vi "Download_LatexPackages_GetPackageList.vi"() -> (3 "Array 2":string[](array[string]))   [LabVIEW 2014]
uses:
  <vilib>/httpClient/LabVIEWHTTPClient.lvlib
  <vilib>/regexp/Match Regular Expression.xnode
panel:
  out "Array 3":string[](array[string])
  out "Array":i32[](array[numeric])
  out "Array String":string[][](array[string])
  out "body":string
  out "headers":string
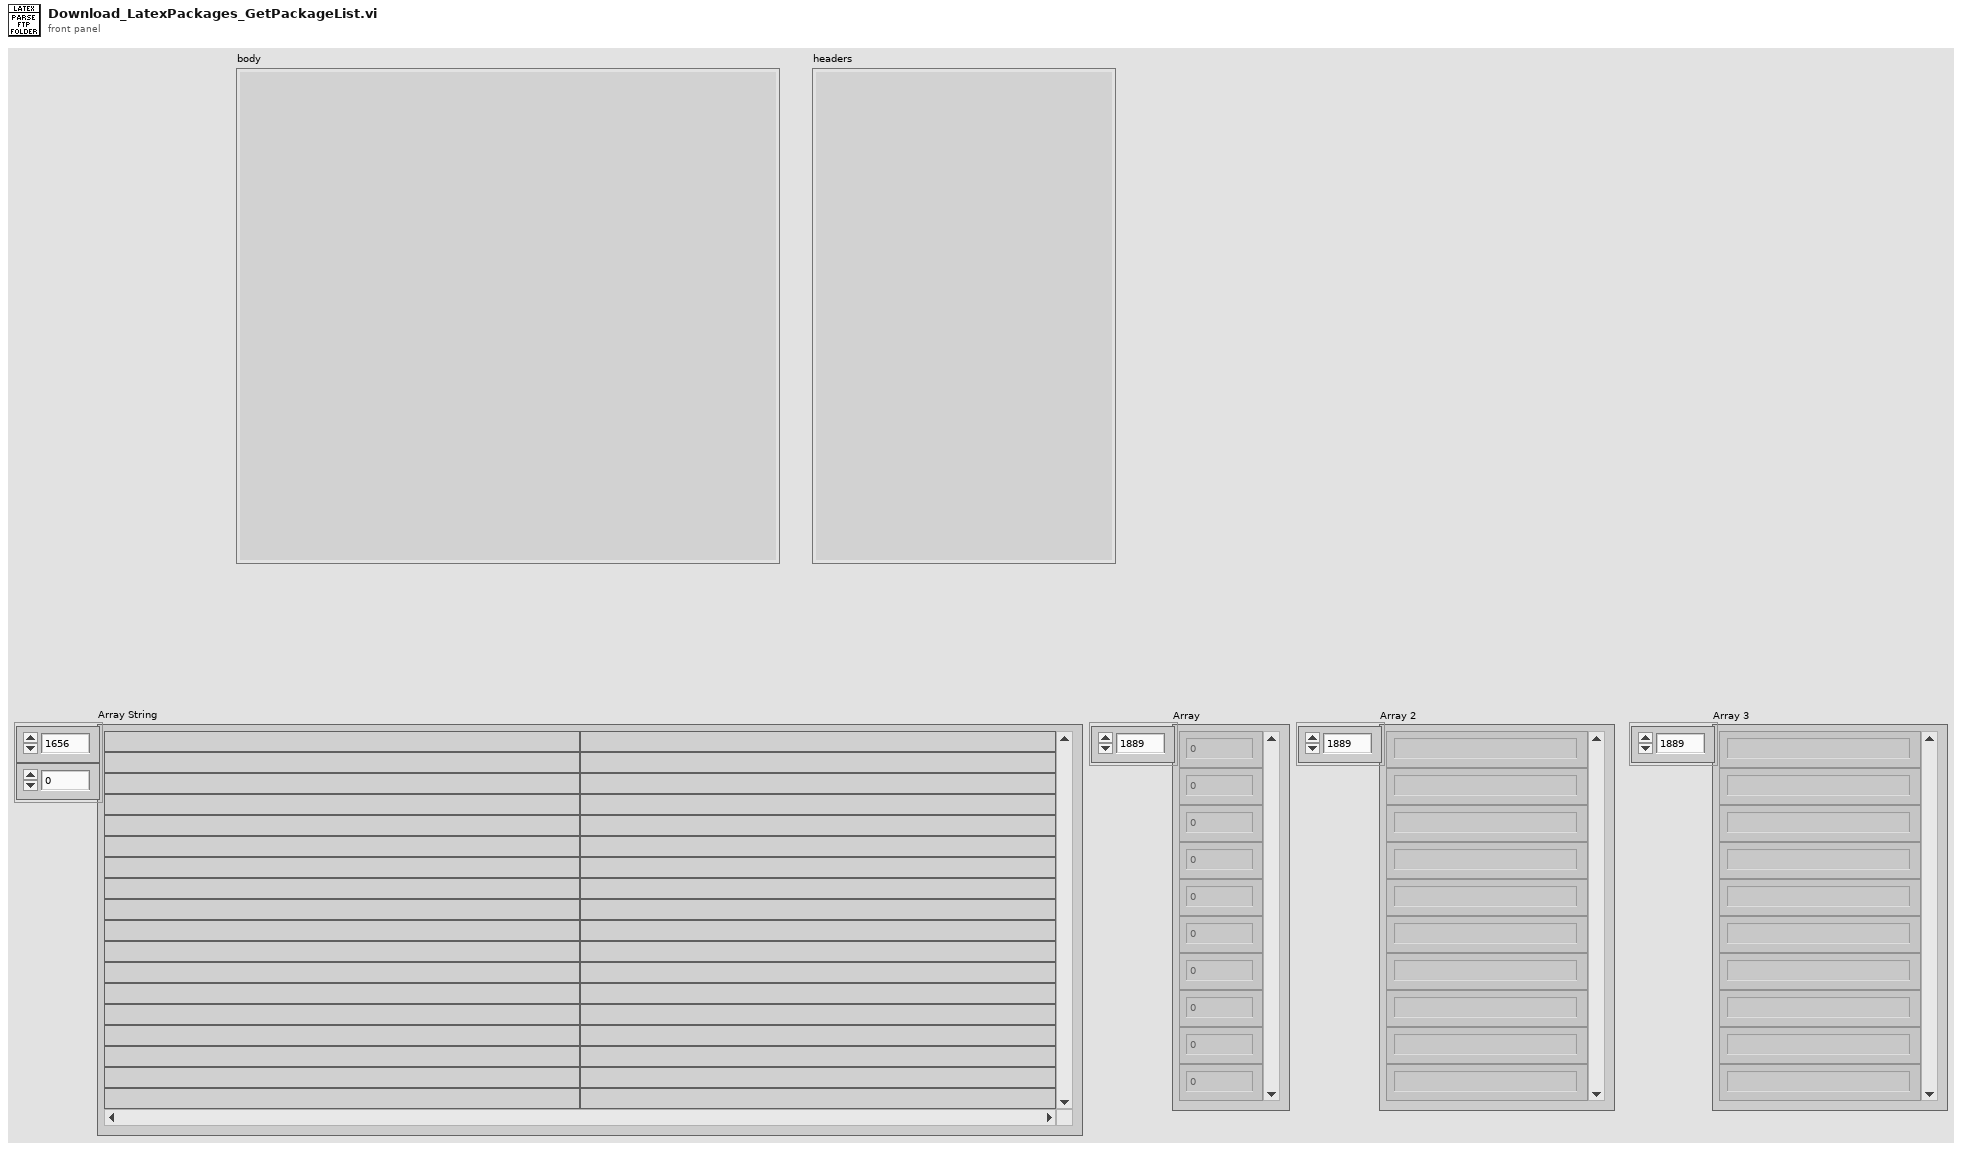
[diagram p1: front panel]
types:
  T1 = typedef "LabVIEWHTTPClient.lvlib/ClientHandle.ctl" = refnum<k1>
diagram:
  (unwired) "[a-zA-z0-9]+\\.zip" ("regular expression")
  w11 = "\nIndex of /ftp/pub/mirror/ctan/macros/latex/contrib\n\nIcon  Name                               Last modified      Size  Description[DIR] Parent Directory                                        -   \n[   ] 12many.zip                         09-Apr-2005 19:47  374K  \n[DIR] 12many/                            09-Apr-2005 19:47    -   \n[   ] ESIEEcv.zip                        29-Apr-2009 20:27  137K  \n[DIR] ESIEEcv/                           29-Apr-2009 20:33    -   \n[DIR] GuIT/                              19-Aug-2012 10:33    -   \n[   ] IEEEconf.zip                       05-Apr-2009 23:09  191K  \n[DIR] IEEEconf/                          05-Apr-2009 23:13    -   \n[   ] IEEEtran.zip                       28-Aug-2015 21:33  1.6M  \n[DIR] IEEEtran/                          28-Aug-2015 21:33    -   \n[   ] LingTrees.zip                      09-Mar-2006 02:00  177K  \n[DIR] LingTrees/                         09-Dec-2013 19:31    -   \n[   ] SIstyle.zip                        16-Jul-2008 15:58  387K  \n[DIR] SIstyle/                           16-Jul-2008 16:03    -   \n[   ] SIunits.zip                        02-Dec-2007 14:15  289K  \n[DIR] SIunits/                           02-Dec-2007 14:23    -   \n[   ] Tabbing.zip                        14-Feb-2010 11:53  215K  \n[DIR] Tabbing/                           14-Feb-2010 12:03    -   \n[   ] TeXemplar.zip                      28-Apr-2005 00:48  7.8K  \n[DIR] TeXemplar/                         01-Feb-2005 20:43    -   \n[   ] a0poster.zip                       28-Apr-2005 00:38  138K  \n[DIR] a0poster/                          01-Feb-2005 20:43    -   \n[DIR] a4/                                23-Jan-2006 08:44    -   \n[   ] a4wide.zip                         05-Jan-2011 01:38  131K  \n[DIR] a4wide/                            05-Jan-2011 02:03    -   \n[   ] a5comb.zip                         13-Feb-2010 22:17   90K  \n[DIR] a5comb/                            13-Feb-2010 22:23    -   \n[   ] aastex.zip                         02-Mar-2016 21:30  1.4M  \n[DIR] aastex/                            02-Mar-2016 21:30    -   \n[   ] abc.zip                            15-May-2016 20:08  281K  \n[DIR] abc/                               15-May-2016 20:08    -   \n[   ] abnt.zip                           31-Oct-2017 16:27   93K  \n[DIR] abnt/                              31-Oct-2017 16:27    -   \n[   ] abntex2.zip                        27-Feb-2016 15:29  6.5M  \n[DIR] abntex2/                           27-Feb-2016 15:29    -   \n[   ] abraces.zip                        31-Aug-2012 11:28  195K  \n[DIR] abraces/                           31-Aug-2012 11:33    -   \n[   ] abstract.zip                       02-Sep-2009 10:13  154K  \n[DIR] abstract/                          02-Sep-2009 10:23    -   \n[   ] achemso.zip                        05-Feb-2018 23:08  872K  \n[DIR] achemso/                           05-Feb-2018 23:08    -   \n[   ] acmart.zip                         07-Feb-2018 20:26  9.5M  \n[DIR] acmart/                            07-Feb-2018 20:26    -   \n[   ] acmconf.zip                        14-May-2008 20:12  103K  \n[DIR] acmconf/                           14-May-2008 19:13    -   \n[   ] acro.zip                           30-Jan-2018 20:37  601K  \n[DIR] acro/                              30-Jan-2018 20:37    -   \n[   ] acroflex.zip                       29-Aug-2016 17:01  1.3M  \n[DIR] acroflex/                          29-Aug-2016 17:01    -   \n[   ] acromake.zip                       15-Feb-2010 23:37  158K  \n[DIR] acromake/                          15-Feb-2010 23:43    -   \n[   ] acronym.zip                        21-Mar-2015 18:51  278K  \n[DIR] acronym/                           21-Mar-2015 18:51    -   \n[   ] acroterm.zip                       19-Nov-2010 14:07  159K  \n[DIR] acroterm/                          19-Nov-2010 14:13    -   \n[   ] acrotex.zip                        01-Mar-2018 17:18  2.9M  \n[DIR] acrotex/                           01-Mar-2018 17:18    -   \n[   ] actuarialangle.zip                 11-Apr-2017 18:43  108K  \n[DIR] actuarialangle/                    11-Apr-2017 18:43    -   \n[   ] actuarialsymbol.zip                14-Jun-2017 22:33  352K  \n[DIR] actuarialsymbol/                   14-Jun-2017 22:33    -   \n[   ] addfont.zip                        01-Sep-2016 13:30  105K  \n[DIR] addfont/                           01-Sep-2016 13:30    -   \n[   ] addlines.zip                       08-Jul-2015 05:24  139K  \n[DIR] addlines/                          08-Jul-2015 05:24    -   \n[   ] adfathesis.zip                     28-Apr-2005 00:49  148K  \n[DIR] adfathesis/                        01-Feb-2005 20:43    -   \n[   ] adjmulticol.zip                    24-Jan-2013 11:50  303K  \n[DIR] adjmulticol/                       24-Jan-2013 11:50    -   \n[   ] adjustbox.zip                      21-May-2012 17:04  789K  \n[DIR] adjustbox/                         21-May-2012 17:13    -   \n[   ] adrconv.zip                        04-Mar-2018 12:53  679K  \n[DIR] adrconv/                           04-Mar-2018 12:53    -   \n[   ] adrlist.zip                        14-May-2008 20:13   47K  \n[DIR] adrlist/                           14-May-2008 19:23    -   \n[   ] adtrees.zip                        20-Jan-2016 14:58  313K  \n[DIR] adtrees/                           20-Jan-2016 14:58    -   \n[   ] advdate.zip                        22-Nov-2010 08:58  145K  \n[DIR] advdate/                           22-Nov-2010 09:03    -   \n[   ] aeb_mlink.zip                      17-Feb-2016 16:07  238K  \n[DIR] aeb_mlink/                         17-Feb-2016 16:07    -   \n[   ] aeb_mobile.zip                     03-Jul-2012 11:37  894K  \n[DIR] aeb_mobile/                        03-Jul-2012 11:43    -   \n[DIR] aeb_pro/                           04-Mar-2018 05:48    -   \n[   ] aeb_tilebg.zip                     18-Feb-2016 20:34  2.3M  \n[DIR] aeb_tilebg/                        18-Feb-2016 20:34    -   \n[   ] aeguill.zip                        29-Apr-2009 20:28   32K  \n[DIR] aeguill/                           29-Apr-2009 20:33    -   \n[   ] afparticle.zip                     23-Dec-2014 21:11  607K  \n[DIR] afparticle/                        23-Dec-2014 21:11    -   \n[   ] afthesis.zip                       28-Jul-2008 22:25   52K  \n[DIR] afthesis/                          28-Jul-2008 21:33    -   \n[   ] aguplus.zip                        21-Feb-2010 22:10  395K  \n[DIR] aguplus/                           21-Feb-2010 22:13    -   \n[   ] aiaa.zip                           28-Apr-2005 00:49  1.0M  \n[DIR] aiaa/                              01-Feb-2005 20:43    -   \n[   ] akktex.zip                         25-Oct-2006 18:48   31K  \n[DIR] akktex/                            25-Oct-2006 18:53    -   \n[   ] akletter.zip                       28-Apr-2005 00:49  217K  \n[DIR] akletter/                          01-Feb-2005 20:43    -   \n[   ] alertmessage.zip                   04-Aug-2015 13:00  112K  \n[DIR] alertmessage/                      04-Aug-2015 13:00    -   \n[   ] alg.zip                            28-Apr-2005 00:49  6.9K  \n[DIR] alg/                               01-Feb-2005 20:43    -   \n[   ] algobox.zip                        04-Sep-2017 22:11  143K  \n[DIR] algobox/                           04-Sep-2017 22:11    -   \n[   ] algorithm2e.zip                    19-Jul-2017 09:50  586K  \n[DIR] algorithm2e/                       19-Jul-2017 09:50    -   \n[   ] algorithmicx.zip                   26-Aug-2009 07:31  179K  \n[DIR] algorithmicx/                      26-Aug-2009 07:31    -   \n[   ] algorithms.zip                     25-Aug-2009 13:09  304K  \n[DIR] algorithms/                        25-Aug-2009 13:13    -   \n[   ] aligned-overset.zip                29-Jan-2018 15:27  352K  \n[DIR] aligned-overset/                   29-Jan-2018 15:27    -   \n[   ] alnumsec.zip                       25-Sep-2007 14:55  129K  \n[DIR] alnumsec/                          25-Sep-2007 14:55    -   \n[   ] alterqcm.zip                       05-Jun-2011 21:03  1.3M  \n[DIR] alterqcm/                          05-Jun-2011 21:03    -   \n[   ] altfont.zip                        07-Dec-2006 01:00  181K  \n[DIR] altfont/                           16-Aug-2008 14:43    -   \n[   ] ametsoc.zip                        05-Jan-2015 19:14  414K  \n[DIR] ametsoc/                           05-Jan-2015 19:14    -   \n[   ] amsaddr.zip                        03-Apr-2013 11:32  193K  \n[DIR] amsaddr/                           03-Apr-2013 11:32    -   \n[   ] amsrefs.zip                        09-Mar-2013 15:03  2.1M  \n[DIR] amsrefs/                           09-Mar-2013 15:03    -   \n[   ] analogclock.zip                    22-Dec-2008 13:50   68K  \n[DIR] analogclock/                       22-Dec-2008 13:50    -   \n[   ] animate.zip                        28-Feb-2018 14:24  3.1M  \n[DIR] animate/                           28-Feb-2018 14:24    -   \n[   ] annot_pro.zip                      28-Aug-2017 12:42  1.7M  \n[DIR] annot_pro/                         28-Aug-2017 12:42    -   \n[   ] anonchap.zip                       14-Feb-2010 23:18  183K  \n[DIR] anonchap/                          14-Feb-2010 23:23    -   \n[   ] answers.zip                        24-Aug-2014 12:16  213K  \n[DIR] answers/                           24-Aug-2014 12:16    -   \n[DIR] anufinalexam/                      16-Jul-2012 11:17    -   \n[   ] anyfontsize.zip                    03-Apr-2010 23:16  181K  \n[DIR] anyfontsize/                       03-Apr-2010 23:16    -   \n[   ] anysize.zip                        01-Jun-2008 22:40   36K  \n[DIR] anysize/                           01-Jun-2008 21:43    -   \n[   ] aomart.zip                         16-Dec-2017 21:56  1.6M  \n[DIR] aomart/                            16-Dec-2017 21:56    -   \n[   ] apa.zip                            23-Dec-2008 13:04   49K  \n[DIR] apa/                               23-Dec-2008 13:13    -   \n[   ] apa6.zip                           20-Jun-2017 21:13  612K  \n[DIR] apa6/                              20-Jun-2017 21:13    -   \n[   ] apa6e.zip                          30-Dec-2012 12:36  249K  \n[DIR] apa6e/                             30-Dec-2012 12:43    -   \n[   ] apacite.zip                        22-Jul-2013 09:38  799K  \n[DIR] apacite/                           22-Jul-2013 09:38    -   \n[   ] appendix.zip                       08-Sep-2009 12:17  168K  \n[DIR] appendix/                          08-Sep-2009 12:23    -   \n[   ] apptools.zip                       29-Nov-2012 15:08   85K  \n[DIR] apptools/                          29-Nov-2012 15:08    -   \n[   ] apxproof.zip                       31-May-2017 11:16  449K  \n[DIR] apxproof/                          31-May-2017 11:16    -   \n[   ] arcs.zip                           28-Apr-2005 00:49   54K  \n[DIR] arcs/                              01-Feb-2005 20:43    -   \n[   ] arraysort.zip                      04-Sep-2013 23:38  305K  \n[DIR] arraysort/                         04-Sep-2013 23:43    -   \n[   ] arsclassica.zip                    31-Oct-2017 18:25  421K  \n[DIR] arsclassica/                       31-Oct-2017 18:25    -   \n[   ] articleingud.zip                   30-Oct-2015 17:00  423K  \n[DIR] articleingud/                      30-Oct-2015 17:00    -   \n[   ] artthreads.zip                     09-Apr-2016 18:30  108K  \n[DIR] artthreads/                        09-Apr-2016 18:30    -   \n[   ] arydshln.zip                       29-Apr-2016 14:56  923K  \n[DIR] arydshln/                          29-Apr-2016 14:56    -   \n[   ] asaetr.zip                         29-Apr-2009 20:29  122K  \n[DIR] asaetr/                            29-Apr-2009 20:33    -   \n[   ] ascelike.zip                       15-Feb-2013 11:40  125K  \n[DIR] ascelike/                          15-Feb-2013 11:43    -   \n[   ] asciilist.zip                      15-May-2016 14:03  387K  \n[DIR] asciilist/                         15-May-2016 14:03    -   \n[   ] ascmac.zip                         09-Mar-2018 16:24  175K  \n[DIR] ascmac/                            09-Mar-2018 16:24    -   \n[   ] askmaps.zip                        04-Dec-2013 19:14  306K  \n[DIR] askmaps/                           04-Dec-2013 19:14    -   \n[   ] aspectratio.zip                    27-Sep-2012 21:09  449K  \n[DIR] aspectratio/                       30-Jan-2012 17:56    -   \n[   ] assignment.zip                     28-Apr-2005 00:49   84K  \n[DIR] assignment/                        01-Feb-2005 20:43    -   \n[   ] assoccnt.zip                       29-Sep-2015 20:56  349K  \n[DIR] assoccnt/                          29-Sep-2015 20:56    -   \n[   ] asyfig.zip                         25-Sep-2012 13:20  225K  \n[DIR] asyfig/                            20-Mar-2010 11:13    -   \n[   ] attachfile.zip                     19-Sep-2016 09:46  359K  \n[DIR] attachfile/                        19-Sep-2016 09:46    -   \n[   ] aucklandthesis.zip                 19-Jun-2016 23:41  696K  \n[DIR] aucklandthesis/                    19-Jun-2016 23:41    -   \n[   ] aurl.zip                           12-Aug-2016 15:34   15K  \n[DIR] aurl/                              12-Aug-2016 15:34    -   \n[   ] authoraftertitle.zip               17-Dec-2011 14:31  113K  \n[DIR] authoraftertitle/                  17-Dec-2011 14:33    -   \n[   ] authorarchive.zip                  21-Feb-2018 07:57  208K  \n[DIR] authorarchive/                     21-Feb-2018 07:57    -   \n[   ] auto-pst-pdf-lua.zip               19-Mar-2018 09:09   70K  \n[DIR] auto-pst-pdf-lua/                  19-Mar-2018 09:09    -   \n[   ] auto-pst-pdf.zip                   26-Aug-2011 08:29  335K  \n[DIR] auto-pst-pdf/                      26-Aug-2011 08:29    -   \n[   ] autobreak.zip                      25-Feb-2017 06:11  540K  \n[DIR] autobreak/                         25-Feb-2017 06:11    -   \n[   ] autonum.zip                        18-Jan-2015 10:18  409K  \n[DIR] autonum/                           18-Jan-2015 10:18    -   \n[   ] autopdf.zip                        10-Dec-2013 19:56  235K  \n[DIR] autopdf/                           10-Dec-2013 19:56    -   \n[   ] avremu.zip                         14-Oct-2014 20:13  189K  \n[DIR] avremu/                            14-Oct-2014 20:13    -   \n[DIR] axodraw2/                          20-Feb-2018 19:13    -   \n[   ] b1encoding.zip                     03-Dec-2005 12:12  151K  \n[DIR] b1encoding/                        05-Dec-2005 20:21    -   \n[DIR] babel-contrib/                     30-Mar-2018 14:15    -   \n[   ] background.zip                     04-Mar-2014 20:59  121K  \n[DIR] background/                        04-Mar-2014 20:59    -   \n[   ] backnaur.zip                       12-Dec-2012 18:29  293K  \n[DIR] backnaur/                          12-Dec-2012 18:33    -   \n[   ] bangorcsthesis.zip                 16-Aug-2017 13:00  345K  \n[DIR] bangorcsthesis/                    16-Aug-2017 13:00    -   \n[   ] bangorexam.zip                     13-Feb-2018 10:02  245K  \n[DIR] bangorexam/                        13-Feb-2018 10:02    -   \n[   ] bankstatement.zip                  14-Nov-2015 18:53  132K  \n[DIR] bankstatement/                     14-Nov-2015 18:53    -   \n[   ] bashful.zip                        10-Mar-2012 20:42  559K  \n[DIR] bashful/                           10-Mar-2012 20:43    -   \n[   ] basicarith.zip                     27-Oct-2014 22:17  224K  \n[DIR] basicarith/                        27-Oct-2014 22:17    -   \n[   ] basque-book.zip                    11-Feb-2014 19:09  437K  \n[DIR] basque-book/                       11-Feb-2014 19:09    -   \n[   ] basque-date.zip                    10-Feb-2014 01:42  192K  \n[DIR] basque-date/                       10-Feb-2014 02:03    -   \n[DIR] bbding/                            23-Feb-2010 23:23    -   \n[   ] bbm.zip                            15-Feb-2010 23:27  403K  \n[DIR] bbm/                               15-Feb-2010 23:33    -   \n[   ] bchart.zip                         18-Apr-2017 22:02  147K  \n[DIR] bchart/                            18-Apr-2017 22:02    -   \n[   ] beamer-FUBerlin.zip                19-Aug-2015 20:36  595K  \n[DIR] beamer-FUBerlin/                   19-Aug-2015 20:36    -   \n[DIR] beamer-contrib/                    29-Jan-2018 23:21    -   \n[   ] beamer.zip                         20-Feb-2018 22:45  2.9M  \n[DIR] beamer/                            20-Feb-2018 22:45    -   \n[   ] beamerposter.zip                   22-Apr-2015 07:02   79K  \n[DIR] beamerposter/                      22-Apr-2015 07:02    -   \n[   ] begingreek.zip                     16-Feb-2015 20:30  698K  \n[DIR] begingreek/                        16-Feb-2015 20:30    -   \n[   ] begriff.zip                        27-May-2005 17:04   44K  \n[DIR] begriff/                           27-May-2005 19:13    -   \n[   ] beilstein.zip                      30-Jan-2018 22:13  1.4M  \n[DIR] beilstein/                         30-Jan-2018 22:13    -   \n[   ] betababel.zip                      10-Jul-2005 16:36  142K  \n[DIR] betababel/                         10-Jul-2005 17:43    -   \n[   ] beton.zip                          01-Jun-2008 22:49   67K  \n[DIR] beton/                             01-Jun-2008 21:53    -   \n[   ] bewerbung.zip                      14-Jul-2015 15:37  917K  \n[DIR] bewerbung/                         14-Jul-2015 15:37    -   \n[   ] bez123.zip                         08-Sep-2009 12:50  268K  \n[DIR] bez123/                            08-Sep-2009 12:53    -   \n[   ] bezos.zip                          25-Feb-2012 16:12  1.0M  \n[DIR] bezos/                             25-Feb-2012 16:12    -   \n[   ] bg.zip                             29-Apr-2009 20:36  120K  \n[DIR] bg/                                25-Sep-2012 13:28    -   \n[   ] bgteubner.zip                      05-May-2017 00:01  2.7M  \n[DIR] bgteubner/                         05-May-2017 00:01    -   \n[   ] bhcexam.zip                        07-Dec-2015 16:01   18K  \n[DIR] bhcexam/                           07-Dec-2015 16:01    -   \n[   ] bibarts.zip                        20-Mar-2016 21:17  1.2M  \n[DIR] bibarts/                           20-Mar-2016 21:17    -   \n[DIR] biblatex-contrib/                  29-Mar-2018 14:02    -   \n[   ] biblatex.zip                       04-Mar-2018 21:16   18M  \n[DIR] biblatex/                          04-Mar-2018 21:16    -   \n[   ] bibleref-french.zip                03-Nov-2014 15:44  716K  \n[DIR] bibleref-french/                   03-Nov-2014 15:44    -   \n[   ] bibleref-german.zip                02-Apr-2011 18:27  787K  \n[DIR] bibleref-german/                   02-Apr-2011 18:27    -   \n[   ] bibleref-lds.zip                   27-Feb-2012 12:33  274K  \n[DIR] bibleref-lds/                      27-Feb-2012 12:43    -   \n[   ] bibleref-mouth.zip                 27-Feb-2012 11:52  381K  \n[DIR] bibleref-mouth/                    27-Feb-2012 12:03    -   \n[   ] bibleref-parse.zip                 11-Apr-2011 08:18  109K  \n[DIR] bibleref-parse/                    11-Apr-2011 08:18    -   \n[   ] bibleref.zip                       01-Jul-2017 09:52  357K  \n[DIR] bibleref/                          01-Jul-2017 09:52    -   \n[   ] bibletext.zip                      02-Sep-2017 12:47  138K  \n[DIR] bibletext/                         02-Sep-2017 12:47    -   \n[   ] bibtopic.zip                       10-Sep-2006 02:00  263K  \n[DIR] bibtopic/                          16-Aug-2008 14:45    -   \n[   ] bibtopicprefix.zip                 31-Oct-2006 15:39  1.1M  \n[DIR] bibtopicprefix/                    31-Oct-2006 15:43    -   \n[   ] bibunits.zip                       30-Apr-2005 15:55  209K  \n[DIR] bibunits/                          01-Feb-2005 20:43    -   \n[   ] bidi.zip                           21-Feb-2018 14:23  3.7M  \n[DIR] bidi/                              21-Feb-2018 14:23    -   \n[   ] bigfoot.zip                        30-Aug-2015 19:08  824K  \n[DIR] bigfoot/                           30-Aug-2015 19:08    -   \n[   ] bigints.zip                        25-Sep-2012 13:39  114K  \n[DIR] bigints/                           26-Feb-2010 19:13    -   \n[   ] binomexp.zip                       11-Jan-2007 02:03   71K  \n[DIR] binomexp/                          11-Jan-2007 02:13    -   \n[   ] biochemistry-colors.zip            21-Apr-2017 19:48   80K  \n[DIR] biochemistry-colors/               21-Apr-2017 19:48    -   \n[   ] biocon.zip                         30-Apr-2005 15:55  289K  \n[DIR] biocon/                            01-Feb-2005 20:43    -   \n[   ] bitpattern.zip                     11-Dec-2015 09:58  177K  \n[DIR] bitpattern/                        11-Dec-2015 09:58    -   \n[   ] bizcard.zip                        29-Apr-2009 20:39   79K  \n[DIR] bizcard/                           29-Apr-2009 20:43    -   \n[   ] blindtext.zip                      06-Jan-2012 11:44  358K  \n[DIR] blindtext/                         06-Jan-2012 11:44    -   \n[   ] blkarray.zip                       28-Feb-2015 05:33  305K  \n[DIR] blkarray/                          28-Feb-2015 05:33    -   \n[   ] block.zip                          16-Feb-2010 20:55   60K  \n[DIR] block/                             16-Feb-2010 21:03    -   \n[   ] blowup.zip                         04-Jan-2018 12:34  368K  \n[DIR] blowup/                            04-Jan-2018 12:34    -   \n[   ] bnumexpr.zip                       05-Dec-2017 23:13  100K  \n[DIR] bnumexpr/                          05-Dec-2017 23:13    -   \n[   ] bohr.zip                           24-Jun-2015 13:04  417K  \n[DIR] bohr/                              24-Jun-2015 13:04    -   \n[   ] boites.zip                         23-Nov-2013 07:43  282K  \n[DIR] boites/                            23-Nov-2013 07:43    -   \n[   ] bold-extra.zip                     16-Feb-2010 21:08  213K  \n[DIR] bold-extra/                        16-Feb-2010 21:13    -   \n[   ] boldtensors.zip                    02-Jul-2007 16:52   56K  \n[DIR] boldtensors/                       02-Jul-2007 16:52    -   \n[   ] bondgraph.zip                      09-Mar-2011 19:57   51K  \n[DIR] bondgraph/                         09-Mar-2011 19:57    -   \n[   ] bondgraphs.zip                     23-Mar-2015 13:26  363K  \n[DIR] bondgraphs/                        23-Mar-2015 13:26    -   \n[   ] bookcover.zip                      21-Jan-2018 22:30  3.1M  \n[DIR] bookcover/                         21-Jan-2018 22:30    -   \n[   ] bookest.zip                        20-Mar-2008 11:06  245K  \n[DIR] bookest/                           20-Mar-2008 11:13    -   \n[   ] booklet.zip                        08-Sep-2009 12:22  231K  \n[DIR] booklet/                           08-Sep-2009 12:23    -   \n[   ] booktabs-de.zip                    30-Mar-2011 20:33  270K  \n[DIR] booktabs-de/                       30-Mar-2011 20:33    -   \n[   ] booktabs.zip                       29-Apr-2016 10:59  301K  \n[DIR] booktabs/                          29-Apr-2016 10:59    -   \n[   ] boolexpr.zip                       12-Apr-2010 11:36  162K  \n[DIR] boolexpr/                          12-Apr-2010 11:43    -   \n[   ] bophook.zip                        31-Dec-2006 15:38   49K  \n[DIR] bophook/                           31-Dec-2006 15:43    -   \n[   ] bosisio.zip                        12-Feb-2010 13:27  526K  \n[DIR] bosisio/                           12-Feb-2010 08:45    -   \n[   ] boxedminipage.zip                  16-Feb-2010 19:50  115K  \n[DIR] boxedminipage/                     16-Feb-2010 19:53    -   \n[   ] boxedminipage2e.zip                10-Mar-2015 11:32  207K  \n[DIR] boxedminipage2e/                   10-Mar-2015 11:32    -   \n[   ] boxhandler.zip                     18-Oct-2012 22:58  342K  \n[DIR] boxhandler/                        18-Oct-2012 22:58    -   \n[   ] bpchem.zip                         23-Aug-2017 16:00  354K  \n[DIR] bpchem/                            23-Aug-2017 16:00    -   \n[   ] br-lex.zip                         01-Aug-2017 22:38   61K  \n[DIR] br-lex/                            01-Aug-2017 22:38    -   \n[   ] bracketkey.zip                     19-Feb-2010 21:28  289K  \n[DIR] bracketkey/                        19-Feb-2010 21:33    -   \n[   ] braille.zip                        04-Dec-2010 12:39   69K  \n[DIR] braille/                           04-Dec-2010 12:43    -   \n[   ] braket.zip                         21-Feb-2010 19:34  212K  \n[DIR] braket/                            21-Feb-2010 19:43    -   \n[   ] brandeis-dissertation.zip          31-Oct-2013 19:18  256K  \n[DIR] brandeis-dissertation/             31-Oct-2013 19:18    -   \n[   ] brclc.zip                          30-Apr-2005 15:56   80K  \n[DIR] brclc/                             01-Feb-2005 20:43    -   \n[   ] breakcites.zip                     10-Jan-2011 19:04  145K  \n[DIR] breakcites/                        10-Jan-2011 19:13    -   \n[   ] breakurl.zip                       12-Apr-2013 10:25  117K  \n[DIR] breakurl/                          12-Apr-2013 10:25    -   \n[   ] bredzenie.zip                      15-May-2017 09:55  216K  \n[DIR] bredzenie/                         15-May-2017 09:55    -   \n[   ] breqn.zip                          28-Jan-2017 14:46  1.2M  \n[DIR] breqn/                             28-Jan-2017 14:46    -   \n[   ] bropd.zip                          14-Oct-2014 21:36   64K  \n[DIR] bropd/                             14-Oct-2014 21:36    -   \n[   ] bsheaders.zip                      15-Apr-2005 07:46  1.6K  \n[DIR] bsheaders/                         15-Apr-2005 09:13    -   \n[   ] bullcntr.zip                       08-Oct-2008 11:56  743K  \n[DIR] bullcntr/                          08-Oct-2008 11:56    -   \n[   ] business-research.zip              01-Dec-2011 10:57  370K  \n[DIR] business-research/                 02-Dec-2011 01:20    -   \n[   ] bussproofs.zip                     21-Aug-2012 20:15  115K  \n[DIR] bussproofs/                        21-Aug-2012 20:15    -   \n[   ] bxcalc.zip                         28-Jan-2018 18:16  338K  \n[DIR] bxcalc/                            28-Jan-2018 18:16    -   \n[   ] bxdvidriver.zip                    13-Feb-2017 17:53  4.5K  \n[DIR] bxdvidriver/                       13-Feb-2017 17:53    -   \n[   ] bxeepic.zip                        18-May-2013 20:51   18K  \n[DIR] bxeepic/                           18-May-2013 20:53    -   \n[   ] bxenclose.zip                      02-Apr-2016 12:35  3.3K  \n[DIR] bxenclose/                         02-Apr-2016 12:35    -   \n[   ] bxnewfont.zip                      02-May-2017 22:55  6.8K  \n[DIR] bxnewfont/                         02-May-2017 22:55    -   \n[   ] bxorigcapt.zip                     03-May-2017 22:28  3.6K  \n[DIR] bxorigcapt/                        03-May-2017 22:28    -   \n[   ] bxpapersize.zip                    08-Oct-2017 08:36  8.1K  \n[DIR] bxpapersize/                       08-Oct-2017 08:36    -   \n[   ] bxpdfver.zip                       11-Feb-2017 22:01   11K  \n[DIR] bxpdfver/                          11-Feb-2017 22:01    -   \n[   ] bxtexlogo.zip                      31-Mar-2018 10:20  420K  \n[DIR] bxtexlogo/                         31-Mar-2018 10:20    -   \n[   ] bytefield.zip                      19-Sep-2017 08:21  573K  \n[DIR] bytefield/                         19-Sep-2017 08:21    -   \n[   ] cachepic.zip                       01-Oct-2009 11:31  163K  \n[DIR] cachepic/                          01-Oct-2009 11:33    -   \n[   ] calcage.zip                        16-Sep-2012 12:24  277K  \n[DIR] calcage/                           16-Sep-2012 12:24    -   \n[   ] calctab.zip                        14-Jul-2009 21:54  405K  \n[DIR] calctab/                           14-Jul-2009 21:54    -   \n[   ] calculation.zip                    06-Jan-2015 20:40  107K  \n[DIR] calculation/                       06-Jan-2015 20:40    -   \n[   ] calculator.zip                     24-Feb-2014 14:22  579K  \n[DIR] calculator/                        24-Feb-2014 14:22    -   \n[   ] calendar.zip                       26-Jul-2005 10:26  479K  \n[DIR] calendar/                          01-Feb-2005 20:43    -   \n[DIR] calendar_barr/                     03-Apr-2010 14:15    -   \n[   ] calrsfs.zip                        20-Feb-2010 21:55  151K  \n[DIR] calrsfs/                           20-Feb-2010 22:03    -   \n[   ] cals.zip                           20-Jan-2017 11:10  526K  \n[DIR] cals/                              20-Jan-2017 11:10    -   \n[   ] calxxxx-yyyy.zip                   03-Jan-2018 08:27  419K  \n[DIR] calxxxx-yyyy/                      03-Jan-2018 08:27    -   \n[   ] calxxxx.zip                        31-Dec-2006 11:32   52K  \n[DIR] calxxxx/                           31-Dec-2006 11:33    -   \n[   ] camel.zip                          30-Apr-2005 15:56  105K  \n[DIR] camel/                             01-Feb-2005 20:43    -   \n[   ] cancel.zip                         30-Dec-2013 10:32  256K  \n[DIR] cancel/                            30-Dec-2013 10:32    -   \n[   ] canoniclayout.zip                  06-Nov-2011 17:04  472K  \n[DIR] canoniclayout/                     06-Nov-2011 17:13    -   \n[   ] capt-of.zip                        25-Sep-2012 13:42   75K  \n[DIR] capt-of/                           22-Jan-2010 17:43    -   \n[   ] captcont.zip                       31-Dec-2006 11:44  110K  \n[DIR] captcont/                          31-Dec-2006 11:53    -   \n[   ] captdef.zip                        06-Mar-2010 15:15  212K  \n[DIR] captdef/                           06-Mar-2010 15:23    -   \n[   ] caption.zip                        22-May-2016 21:20  2.0M  \n[DIR] caption/                           22-May-2016 21:20    -   \n[   ] carbohydrates.zip                  02-Dec-2015 12:19  477K  \n[DIR] carbohydrates/                     02-Dec-2015 12:19    -   \n[   ] carlisle.zip                       11-May-2010 22:08   34K  \n[DIR] carlisle/                          11-May-2010 22:13    -   \n[   ] cascadilla.zip                     18-Jan-2012 11:58   98K  \n[DIR] cascadilla/                        18-Jan-2012 11:58    -   \n[   ] cases.zip                          20-Feb-2010 22:54  303K  \n[DIR] cases/                             20-Feb-2010 23:03    -   \n[   ] catchfilebetweentags.zip           19-Feb-2011 16:39  151K  \n[DIR] catchfilebetweentags/              19-Feb-2011 16:43    -   \n[   ] catechis.zip                       14-Jan-2018 10:32  402K  \n[DIR] catechis/                          14-Jan-2018 10:32    -   \n[   ] catoptions.zip                     30-Aug-2014 10:15   63K  \n[DIR] catoptions/                        30-Aug-2014 10:15    -   \n[   ] ccaption.zip                       07-Aug-2011 14:46  493K  \n[DIR] ccaption/                          07-Aug-2011 14:53    -   \n[   ] ccfonts.zip                        21-Feb-2010 01:25  193K  \n[DIR] ccfonts/                           21-Feb-2010 02:03    -   \n[   ] cchess.zip                         30-Apr-2005 15:56   15K  \n[DIR] cchess/                            01-Feb-2005 20:43    -   \n[   ] cclicenses.zip                     30-May-2005 14:36   84K  \n[DIR] cclicenses/                        30-May-2005 16:43    -   \n[   ] cd-cover.zip                       21-Feb-2010 01:35  311K  \n[DIR] cd-cover/                          21-Feb-2010 02:03    -   \n[   ] cd.zip                             27-Jun-2014 12:21   82K  \n[DIR] cd/                                27-Jun-2014 12:23    -   \n[   ] cdpbundl.zip                       12-Feb-2018 06:13  829K  \n[DIR] cdpbundl/                          12-Feb-2018 06:13    -   \n[   ] cell.zip                           14-Dec-2010 22:28   12K  \n[DIR] cell/                              14-Dec-2010 22:33    -   \n[   ] cellspace.zip                      13-Aug-2017 17:02  329K  \n[DIR] cellspace/                         13-Aug-2017 17:02    -   \n[   ] cellwise.zip                       08-Sep-2012 13:55  2.1K  \n[DIR] cellwise/                          08-Sep-2012 14:03    -   \n[   ] censor.zip                         31-Jul-2013 09:45  182K  \n[DIR] censor/                            31-Jul-2013 09:45    -   \n[   ] cesenaexam.zip                     05-Aug-2017 09:52  508K  \n[DIR] cesenaexam/                        05-Aug-2017 09:52    -   \n[   ] cfr-initials.zip                   06-Apr-2015 07:10  683K  \n[DIR] cfr-initials/                      06-Apr-2015 07:10    -   \n[   ] cfr-lm.zip                         02-Feb-2015 11:49  3.6M  \n[DIR] cfr-lm/                            02-Feb-2015 11:49    -   \n[   ] changebar.zip                      11-Mar-2018 17:34  745K  \n[DIR] changebar/                         11-Mar-2018 17:34    -   \n[   ] changelayout.zip                   15-Oct-2009 18:09   61K  \n[DIR] changelayout/                      15-Oct-2009 18:13    -   \n[   ] changepage.zip                     20-Oct-2009 20:40  281K  \n[DIR] changepage/                        20-Oct-2009 20:43    -   \n[   ] changes.zip                        28-Apr-2015 00:00  535K  \n[DIR] changes/                           28-Apr-2015 00:00    -   \n[   ] chappg.zip                         30-May-2009 11:04  193K  \n[DIR] chappg/                            30-May-2009 11:13    -   \n[   ] chapterfolder.zip                  25-Nov-2005 11:19  186K  \n[DIR] chapterfolder/                     16-Aug-2008 14:45    -   \n[   ] chbibref.zip                       21-Feb-2010 11:17  166K  \n[DIR] chbibref/                          21-Feb-2010 11:23    -   \n[   ] cheatsheet.zip                     18-Aug-2017 04:52  400K  \n[DIR] cheatsheet/                        18-Aug-2017 04:52    -   \n[   ] checklistings.zip                  04-Sep-2015 18:08  369K  \n[DIR] checklistings/                     04-Sep-2015 18:08    -   \n[   ] chemarrow.zip                      21-Feb-2010 18:49  433K  \n[DIR] chemarrow/                         21-Feb-2010 18:53    -   \n[   ] chemcompounds.zip                  05-Dec-2006 16:10  118K  \n[DIR] chemcompounds/                     05-Dec-2006 16:13    -   \n[   ] chemcono.zip                       21-Feb-2010 19:06  235K  \n[DIR] chemcono/                          21-Feb-2010 19:13    -   \n[   ] chemexec.zip                       06-Mar-2011 17:27  369K  \n[DIR] chemexec/                          06-Mar-2011 17:27    -   \n[   ] chemfig.zip                        08-Mar-2018 20:41  2.2M  \n[DIR] chemfig/                           08-Mar-2018 20:41    -   \n[   ] chemformula.zip                    23-Mar-2017 14:37  970K  \n[DIR] chemformula/                       23-Mar-2017 14:37    -   \n[   ] chemgreek.zip                      20-Dec-2016 12:45  720K  \n[DIR] chemgreek/                         20-Dec-2016 12:45    -   \n[   ] chemmacros.zip                     29-Aug-2017 12:53  1.1M  \n[DIR] chemmacros/                        29-Aug-2017 12:53    -   \n[   ] chemnum.zip                        14-Apr-2016 13:35  795K  \n[DIR] chemnum/                           14-Apr-2016 13:35    -   \n[   ] chemschemex.zip                    23-Feb-2018 21:14  316K  \n[DIR] chemschemex/                       23-Feb-2018 21:14    -   \n[   ] chemsec.zip                        15-Mar-2018 19:50  260K  \n[DIR] chemsec/                           15-Mar-2018 19:50    -   \n[   ] chemstyle.zip                      05-Jul-2013 11:10  291K  \n[DIR] chemstyle/                         05-Jul-2013 11:10    -   \n[   ] chemsym.zip                        23-Dec-2005 15:51  308K  \n[DIR] chemsym/                           13-Aug-2008 12:33    -   \n[   ] chess-problem-diagrams.zip         08-Jan-2016 10:22  313K  \n[DIR] chess-problem-diagrams/            08-Jan-2016 10:22    -   \n[   ] chessboard.zip                     01-May-2014 22:27  656K  \n[DIR] chessboard/                        01-May-2014 22:27    -   \n[   ] chessfss.zip                       10-Jan-2008 19:02  1.7M  \n[DIR] chessfss/                          10-Jan-2008 19:03    -   \n[   ] chet.zip                           19-Aug-2017 23:08  176K  \n[DIR] chet/                              19-Aug-2017 23:08    -   \n[   ] chextras.zip                       20-Jul-2012 14:21  134K  \n[DIR] chextras/                          20-Jul-2012 14:21    -   \n[   ] childdoc.zip                       17-Jan-2018 14:10  252K  \n[DIR] childdoc/                          17-Jan-2018 14:10    -   \n[   ] china2e.zip                        30-Apr-2005 15:56  106K  \n[DIR] china2e/                           01-Feb-2005 20:43    -   \n[   ] chkfloat.zip                       19-Aug-2012 23:58   46K  \n[DIR] chkfloat/                          20-Aug-2012 02:03    -   \n[   ] chletter.zip                       11-Oct-2010 07:19  146K  \n[DIR] chletter/                          11-Oct-2010 07:19    -   \n[   ] chngcntr.zip                       22-Feb-2010 20:14  229K  \n[DIR] chngcntr/                          22-Feb-2010 20:23    -   \n[   ] chronology.zip                     23-Jul-2015 07:01   14K  \n[DIR] chronology/                        23-Jul-2015 07:01    -   \n[   ] chronosys.zip                      28-May-2012 13:33  247K  \n[DIR] chronosys/                         28-May-2012 13:33    -   \n[   ] chscite.zip                        16-Dec-2012 17:14  195K  \n[DIR] chscite/                           16-Dec-2012 17:23    -   \n[   ] circle.zip                         22-Feb-2010 19:46  177K  \n[DIR] circle/                            22-Feb-2010 19:53    -   \n[   ] cite.zip                           03-Mar-2015 14:34  242K  \n[DIR] cite/                              03-Mar-2015 14:34    -   \n[DIR] citeref/                           30-Jul-2005 12:44    -   \n[   ] cje.zip                            23-Feb-2018 14:39  651K  \n[DIR] cje/                               23-Feb-2018 14:39    -   \n[   ] cjw.zip                            25-Sep-2012 14:09  519K  \n[DIR] cjw/                               25-Dec-2008 20:23    -   \n[   ] classics.zip                       03-Feb-2013 19:05  205K  \n[DIR] classics/                          03-Feb-2013 19:13    -   \n[   ] classicthesis.zip                  22-Oct-2017 10:02  583K  \n[DIR] classicthesis/                     22-Oct-2017 10:02    -   \n[   ] cleanthesis.zip                    27-Aug-2015 10:17  1.3M  \n[DIR] cleanthesis/                       27-Aug-2015 10:17    -   \n[   ] clefval.zip                        28-Dec-2009 11:06  335K  \n[DIR] clefval/                           28-Dec-2009 11:13    -   \n[   ] cleveref.zip                       05-Mar-2018 09:34  468K  \n[DIR] cleveref/                          05-Mar-2018 09:34    -   \n[   ] clipboard.zip                      19-Jan-2013 09:43   37K  \n[DIR] clipboard/                         19-Jan-2013 09:53    -   \n[   ] clock.zip                          30-Apr-2005 15:57   75K  \n[DIR] clock/                             23-Jan-2006 08:44    -   \n[   ] clrscode.zip                       29-Mar-2007 22:40   36K  \n[DIR] clrscode/                          29-Mar-2007 22:43    -   \n[   ] clrscode3e.zip                     09-Aug-2014 05:42   72K  \n[DIR] clrscode3e/                        09-Aug-2014 05:42    -   \n[   ] cmap.zip                           06-Sep-2008 23:52   15K  \n[DIR] cmap/                              06-Sep-2008 22:53    -   \n[   ] cmcyralt.zip                       25-Sep-2012 14:11   25K  \n[DIR] cmcyralt/                          01-Feb-2005 20:43    -   \n[   ] cmdstring.zip                      24-Apr-2007 13:52  339K  \n[DIR] cmdstring/                         24-Apr-2007 13:53    -   \n[   ] cmdtrack.zip                       19-Dec-2012 17:05  133K  \n[DIR] cmdtrack/                          19-Dec-2012 17:13    -   \n[   ] cmpj.zip                           10-May-2017 15:11  607K  \n[DIR] cmpj/                              10-May-2017 15:11    -   \n[   ] cmsd.zip                           30-Apr-2005 15:57  3.7K  \n[DIR] cmsd/                              01-Feb-2005 20:43    -   \n[   ] cnbwp.zip                          02-Jan-2014 08:30  799K  \n[DIR] cnbwp/                             02-Jan-2014 08:30    -   \n[   ] cnltx.zip                          17-Aug-2015 17:02  823K  \n[DIR] cnltx/                             17-Aug-2015 17:02    -   \n[   ] cntdwn.zip                         26-Nov-2014 17:56  119K  \n[DIR] cntdwn/                            26-Nov-2014 17:56    -   \n[   ] cntformats.zip                     20-Jul-2014 15:20  420K  \n[DIR] cntformats/                        20-Jul-2014 15:20    -   \n[   ] cntperchap.zip                     01-Jun-2015 07:20  268K  \n[DIR] cntperchap/                        01-Jun-2015 07:20    -   \n[   ] codedoc.zip                        30-Mar-2010 11:24  409K  \n[DIR] codedoc/                           30-Mar-2010 11:33    -   \n[   ] codepage.zip                       25-Sep-2012 14:14  291K  \n[DIR] codepage/                          18-Jan-2011 23:33    -   \n[   ] codesection.zip                    27-Jun-2014 23:12  371K  \n[DIR] codesection/                       27-Jun-2014 23:13    -   \n[   ] codicefiscaleitaliano.zip          28-Sep-2012 18:32  221K  \n[DIR] codicefiscaleitaliano/             06-May-2012 15:13    -   \n[   ] collcell.zip                       27-Feb-2011 19:07  230K  \n[DIR] collcell/                          27-Feb-2011 19:07    -   \n[   ] collectbox.zip                     21-May-2012 18:04  271K  \n[DIR] collectbox/                        21-May-2012 18:04    -   \n[   ] collref.zip                        17-Jan-2018 14:20  272K  \n[DIR] collref/                           17-Jan-2018 14:20    -   \n[   ] colordoc.zip                       14-May-2010 01:22  183K  \n[DIR] colordoc/                          14-May-2010 02:03    -   \n[   ] colorinfo.zip                      30-Apr-2005 15:57  2.6K  \n[DIR] colorinfo/                         01-Feb-2005 20:43    -   \n[   ] coloring.zip                       11-May-2016 07:30   27K  \n[DIR] coloring/                          11-May-2016 07:30    -   \n[   ] colorspace.zip                     06-Oct-2016 16:23  120K  \n[DIR] colorspace/                        06-Oct-2016 16:23    -   \n[   ] colortbl.zip                       25-Sep-2012 14:18  557K  \n[DIR] colortbl/                          14-Feb-2012 10:53    -   \n[   ] colorwav.zip                       14-Apr-2007 15:25  102K  \n[DIR] colorwav/                          14-Apr-2007 15:33    -   \n[   ] colorweb.zip                       21-Aug-2013 16:57  1.6M  \n[DIR] colorweb/                          21-Aug-2013 16:57    -   \n[   ] colourchange.zip                   16-Mar-2011 00:08  230K  \n[DIR] colourchange/                      16-Mar-2011 02:03    -   \n[   ] combelow.zip                       24-May-2010 13:32   96K  \n[DIR] combelow/                          24-May-2010 13:33    -   \n[   ] combine.zip                        10-Jul-2010 15:28  484K  \n[DIR] combine/                           10-Jul-2010 15:33    -   \n[   ] combinedgraphics.zip               16-Jul-2012 17:05  440K  \n[DIR] combinedgraphics/                  16-Jul-2012 17:05    -   \n[   ] comicsans.zip                      20-Dec-2013 09:37  314K  \n[DIR] comicsans/                         20-Dec-2013 09:37    -   \n[   ] comma.zip                          11-May-2010 22:05  151K  \n[DIR] comma/                             11-May-2010 22:13    -   \n[   ] commath.zip                        18-Jul-2006 17:09  104K  \n[DIR] commath/                           18-Jul-2006 17:13    -   \n[   ] comment.zip                        25-Aug-2016 07:37  532K  \n[DIR] comment/                           25-Aug-2016 07:37    -   \n[DIR] compactbib/                        03-Apr-2010 14:15    -   \n[   ] complexity.zip                     16-Sep-2017 18:06  264K  \n[DIR] complexity/                        16-Sep-2017 18:06    -   \n[   ] computational-complexity.zip       19-Jul-2017 19:03  888K  \n[DIR] computational-complexity/          19-Jul-2017 19:03    -   \n[   ] concepts.zip                       05-Jan-2013 23:50  317K  \n[DIR] concepts/                          05-Jan-2013 23:53    -   \n[   ] concmath.zip                       22-Feb-2010 22:20  352K  \n[DIR] concmath/                          22-Feb-2010 22:23    -   \n[   ] concprog.zip                       30-Apr-2005 15:57  5.0K  \n[DIR] concprog/                          01-Feb-2005 20:43    -   \n[DIR] conferences/                       25-Sep-2012 14:23    -   \n[   ] constants.zip                      30-Mar-2008 13:33   99K  \n[DIR] constants/                         30-Mar-2008 13:43    -   \n[   ] conteq.zip                         17-Jul-2015 20:45  390K  \n[DIR] conteq/                            17-Jul-2015 20:45    -   \n[   ] continue.zip                       06-Jan-2016 06:12  337K  \n[DIR] continue/                          06-Jan-2016 06:12    -   \n[   ] contour.zip                        30-Apr-2005 16:13  159K  \n[DIR] contour/                           30-Apr-2005 16:13    -   \n[   ] contracard.zip                     24-Sep-2013 20:45  190K  \n[DIR] contracard/                        24-Sep-2013 20:45    -   \n[   ] conv-xkv.zip                       20-Mar-2017 15:08   84K  \n[DIR] conv-xkv/                          20-Mar-2017 15:08    -   \n[   ] cooking-units.zip                  23-Oct-2017 19:07  629K  \n[DIR] cooking-units/                     23-Oct-2017 19:07    -   \n[   ] cooking.zip                        09-Dec-2006 15:39   67K  \n[DIR] cooking/                           09-Dec-2006 15:43    -   \n[   ] cookingsymbols.zip                 28-Dec-2014 20:48  377K  \n[DIR] cookingsymbols/                    28-Dec-2014 20:48    -   \n[   ] cookybooky.zip                     13-Oct-2009 09:50  1.0M  \n[DIR] cookybooky/                        13-Oct-2009 09:50    -   \n[   ] cool.zip                           30-Dec-2006 22:39  436K  \n[DIR] cool/                              30-Dec-2006 22:43    -   \n[   ] coollist.zip                       20-Sep-2009 16:02  116K  \n[DIR] coollist/                          20-Sep-2009 16:03    -   \n[   ] coolstr.zip                        09-Sep-2009 20:14  122K  \n[DIR] coolstr/                           09-Sep-2009 20:23    -   \n[   ] coolthms.zip                       08-Feb-2013 10:59  116K  \n[DIR] coolthms/                          08-Feb-2013 11:03    -   \n[   ] cooltooltips.zip                   15-Mar-2006 13:48  199K  \n[DIR] cooltooltips/                      15-Mar-2006 14:13    -   \n[   ] coordsys.zip                       06-Feb-2006 20:57  276K  \n[DIR] coordsys/                          16-Aug-2008 14:45    -   \n[   ] copyedit.zip                       21-Jul-2015 13:41  309K  \n[DIR] copyedit/                          21-Jul-2015 13:41    -   \n[   ] copyrightbox.zip                   11-Dec-2011 18:33  2.9M  \n[DIR] copyrightbox/                      11-Dec-2011 18:33    -   \n[   ] correctmathalign.zip               04-Apr-2017 05:27  570K  \n[DIR] correctmathalign/                  04-Apr-2017 05:27    -   \n[   ] corridx.zip                        23-May-2005 22:29  178K  \n[DIR] corridx/                           23-May-2005 22:29    -   \n[   ] coseoul.zip                        06-Sep-2011 15:26  160K  \n[DIR] coseoul/                           06-Sep-2011 15:26    -   \n[   ] counttexruns.zip                   31-Aug-2012 13:56  228K  \n[DIR] counttexruns/                      31-Aug-2012 13:56    -   \n[   ] courseoutline.zip                  30-Apr-2005 15:57  5.6K  \n[DIR] courseoutline/                     23-Jan-2006 08:43    -   \n[   ] coursepaper.zip                    30-Apr-2005 15:57  6.0K  \n[DIR] coursepaper/                       23-Jan-2006 08:43    -   \n[   ] coverpage.zip                      24-Feb-2006 12:28  294K  \n[DIR] coverpage/                         24-Feb-2006 12:28    -   \n[   ] covington.zip                      25-May-2017 12:31  523K  \n[DIR] covington/                         25-May-2017 12:31    -   \n[   ] cprotect.zip                       27-Jan-2011 21:19  584K  \n[DIR] cprotect/                          27-Jan-2011 21:23    -   \n[   ] cpssp.zip                          06-Jun-2009 14:55  518K  \n[DIR] cpssp/                             06-Jun-2009 15:03    -   \n[   ] cquthesis.zip                      06-Mar-2018 20:51  1.1M  \n[DIR] cquthesis/                         06-Mar-2018 20:51    -   \n[   ] crbox.zip                          04-Apr-2013 12:44   30K  \n[DIR] crbox/                             04-Apr-2013 12:44    -   \n[   ] crop.zip                           10-Jul-2009 18:41  215K  \n[DIR] crop/                              10-Jul-2009 18:43    -   \n[   ] crossreference.zip                 01-Jan-2007 15:04   41K  \n[DIR] crossreference/                    01-Jan-2007 15:13    -   \n[   ] crossreftools.zip                  18-Mar-2018 17:07  344K  \n[DIR] crossreftools/                     18-Mar-2018 17:07    -   \n[   ] crosswrd.zip                       01-Feb-2010 16:51  229K  \n[DIR] crosswrd/                          01-Feb-2010 16:53    -   \n[   ] cryptocode.zip                     23-Apr-2015 07:04  652K  \n[DIR] cryptocode/                        23-Apr-2015 07:04    -   \n[   ] csbulletin.zip                     19-Feb-2017 09:59  270K  \n[DIR] csbulletin/                        19-Feb-2017 09:59    -   \n[   ] csquotes.zip                       11-Feb-2018 12:38  328K  \n[DIR] csquotes/                          11-Feb-2018 12:38    -   \n[   ] css-colors.zip                     21-Apr-2017 19:12  2.0M  \n[DIR] css-colors/                        21-Apr-2017 19:12    -   \n[   ] csvsimple.zip                      01-Jul-2016 18:26  756K  \n[DIR] csvsimple/                         01-Jul-2016 18:26    -   \n[   ] ctable.zip                         18-Oct-2015 21:44  761K  \n[DIR] ctable/                            18-Oct-2015 21:44    -   \n[   ] cuisine.zip                        27-Jun-2014 19:06  261K  \n[DIR] cuisine/                           27-Jun-2014 19:06    -   \n[   ] currency.zip                       28-May-2017 15:36  659K  \n[DIR] currency/                          28-May-2017 15:36    -   \n[   ] currfile.zip                       23-Apr-2016 21:10  177K  \n[DIR] currfile/                          23-Apr-2016 21:10    -   \n[   ] currvita.zip                       09-Dec-2006 15:56  103K  \n[DIR] currvita/                          09-Dec-2006 16:03    -   \n[   ] cursor.zip                         01-Jan-2007 17:19   16K  \n[DIR] cursor/                            01-Jan-2007 17:23    -   \n[   ] curve.zip                          14-Dec-2010 18:10  273K  \n[DIR] curve/                             14-Dec-2010 18:13    -   \n[   ] curve2e.zip                        11-Jul-2015 19:54  665K  \n[DIR] curve2e/                           11-Jul-2015 19:54    -   \n[   ] curves.zip                         09-Sep-2017 10:51  334K  \n[DIR] curves/                            09-Sep-2017 10:51    -   \n[   ] custom-bib.zip                     18-Nov-2011 11:11  880K  \n[DIR] custom-bib/                        18-Nov-2011 11:11    -   \n[   ] cutwin.zip                         27-Sep-2012 21:04  308K  \n[DIR] cutwin/                            04-Oct-2010 12:13    -   \n[   ] cv.zip                             30-Jun-2008 23:28   55K  \n[DIR] cv/                                30-Jun-2008 22:33    -   \n[   ] cv4tw.zip                          12-Jul-2014 08:49  135K  \n[DIR] cv4tw/                             12-Jul-2014 08:49    -   \n[   ] cvsty.zip                          30-Apr-2005 15:57  3.9K  \n[DIR] cvsty/                             01-Feb-2005 20:43    -   \n[   ] cweb.zip                           19-Jan-2013 01:32  368K  \n[DIR] cweb/                              19-Jan-2013 02:03    -   \n[   ] cyber.zip                          01-Mar-2018 06:12  253K  \n[DIR] cyber/                             01-Mar-2018 06:12    -   \n[   ] cybercic.zip                       24-Jun-2015 08:09  193K  \n[DIR] cybercic/                          24-Jun-2015 08:09    -   \n[   ] dashbox.zip                        05-Aug-2011 01:17  158K  \n[DIR] dashbox/                           05-Aug-2011 01:17    -   \n[   ] dashrule.zip                       30-Mar-2013 10:17  234K  \n[DIR] dashrule/                          30-Mar-2013 10:17    -   \n[   ] dashundergaps.zip                  25-Sep-2012 14:34  133K  \n[DIR] dashundergaps/                     07-Jul-2011 10:33    -   \n[   ] dataref.zip                        06-Jan-2017 12:58  247K  \n[DIR] dataref/                           06-Jan-2017 12:58    -   \n[   ] datatool.zip                       12-Nov-2017 18:01  2.7M  \n[DIR] datatool/                          12-Nov-2017 18:01    -   \n[   ] dateiliste.zip                     13-Oct-2012 20:21  258K  \n[DIR] dateiliste/                        13-Oct-2012 20:21    -   \n[   ] datenumber.zip                     22-Oct-2006 13:31  110K  \n[DIR] datenumber/                        22-Oct-2006 12:33    -   \n[   ] datepicker-pro.zip                 07-May-2016 19:13  717K  \n[DIR] datepicker-pro/                    07-May-2016 19:13    -   \n[   ] dates.zip                          30-Apr-2005 15:57   24K  \n[DIR] dates/                             01-Feb-2005 20:43    -   \n[DIR] datetime2-contrib/                 21-Mar-2018 20:07    -   \n[   ] datetime2.zip                      12-Jul-2016 15:09  1.0M  \n[DIR] datetime2/                         12-Jul-2016 15:09    -   \n[   ] dblfloatfix.zip                    29-Jan-2013 13:45  216K  \n[DIR] dblfloatfix/                       29-Jan-2013 13:53    -   \n[   ] dccpaper.zip                       20-Oct-2017 14:39  411K  \n[DIR] dccpaper/                          20-Oct-2017 14:39    -   \n[   ] decimal.zip                        05-Jun-2011 22:02  162K  \n[DIR] decimal/                           05-Jun-2011 22:02    -   \n[   ] decorule.zip                       07-Aug-2011 14:11  409K  \n[DIR] decorule/                          07-Aug-2011 14:13    -   \n[   ] deleq.zip                          24-Dec-2005 14:13  282K  \n[DIR] deleq/                             18-Aug-2008 11:13    -   \n[   ] delim.zip                          15-Sep-2011 20:19  294K  \n[DIR] delim/                             15-Sep-2011 20:19    -   \n[   ] delimseasy.zip                     05-Feb-2016 19:29  232K  \n[DIR] delimseasy/                        05-Feb-2016 19:29    -   \n[   ] delimset.zip                       17-Jan-2018 14:20  320K  \n[DIR] delimset/                          17-Jan-2018 14:20    -   \n[   ] denisbdoc.zip                      01-Jan-2017 22:00   20K  \n[DIR] denisbdoc/                         01-Jan-2017 22:00    -   \n[   ] designcon.zip                      18-Sep-2012 07:42   69K  \n[DIR] designcon/                         18-Sep-2012 07:42    -   \n[   ] dfgproposal.zip                    15-Apr-2016 14:28  1.3M  \n[DIR] dfgproposal/                       15-Apr-2016 14:28    -   \n[   ] dhua.zip                           20-Sep-2011 00:24  327K  \n[DIR] dhua/                              20-Sep-2011 00:24    -   \n[   ] diadia.zip                         20-May-2015 19:04  449K  \n[DIR] diadia/                            20-May-2015 19:04    -   \n[   ] diagbox.zip                        28-Dec-2016 09:39  278K  \n[DIR] diagbox/                           28-Dec-2016 09:39    -   \n[   ] diagmac.zip                        30-Apr-2009 00:07   69K  \n[DIR] diagmac/                           30-Apr-2009 02:03    -   \n[   ] diagmac2.zip                       16-May-2009 23:48  222K  \n[DIR] diagmac2/                          16-May-2009 23:53    -   \n[   ] diagnose.zip                       30-Apr-2005 15:58   82K  \n[DIR] diagnose/                          01-Feb-2005 20:43    -   \n[   ] dialogl.zip                        25-Jan-2013 11:16  775K  \n[DIR] dialogl/                           25-Jan-2013 11:16    -   \n[   ] dichokey.zip                       23-Feb-2010 23:24  208K  \n[DIR] dichokey/                          23-Feb-2010 23:33    -   \n[   ] diffcoeff.zip                      27-Jun-2016 20:44  954K  \n[DIR] diffcoeff/                         27-Jun-2016 20:44    -   \n[   ] digiconfigs.zip                    22-Jun-2006 17:28  121K  \n[DIR] digiconfigs/                       22-Jun-2006 17:33    -   \n[   ] dijkstra.zip                       09-Sep-2017 20:33  371K  \n[DIR] dijkstra/                          09-Sep-2017 20:33    -   \n[   ] dinbrief.zip                       27-Jul-2007 17:03  473K  \n[DIR] dinbrief/                          27-Jul-2007 17:03    -   \n[   ] dirtytalk.zip                      21-Nov-2010 18:23  388K  \n[DIR] dirtytalk/                         21-Nov-2010 18:33    -   \n[   ] disser.zip                         06-Mar-2017 17:12  217K  \n[DIR] disser/                            06-Mar-2017 17:12    -   \n[   ] dithesis.zip                       18-Jun-2014 20:17  208K  \n[DIR] dithesis/                          18-Jun-2014 20:17    -   \n[   ] divine.zip                         12-Mar-2013 11:05  280K  \n[DIR] divine/                            12-Mar-2013 11:05    -   \n[   ] dlfltxb.zip                        04-Mar-2010 23:25  721K  \n[DIR] dlfltxb/                           04-Mar-2010 23:33    -   \n[   ] dnaseq.zip                         23-Feb-2010 23:31  207K  \n[DIR] dnaseq/                            23-Feb-2010 23:33    -   \n[   ] doclicense.zip                     17-Feb-2018 15:48  612K  \n[DIR] doclicense/                        17-Feb-2018 15:48    -   \n[   ] docmfp.zip                         02-Sep-2009 16:52  155K  \n[DIR] docmfp/                            02-Sep-2009 16:53    -   \n[   ] docmute.zip                        22-Mar-2012 21:44  147K  \n[DIR] docmute/                           22-Mar-2012 21:44    -   \n[   ] doctools.zip                       28-Jun-2014 00:36  598K  \n[DIR] doctools/                          28-Jun-2014 02:03    -   \n[   ] documentation.zip                  30-Nov-2011 16:52   95K  \n[DIR] documentation/                     30-Nov-2011 16:52    -   \n[   ] doi.zip                            24-Jul-2007 23:55  2.3K  \n[DIR] doi/                               25-Jul-2007 02:03    -   \n[   ] doipubmed.zip                      20-Aug-2007 19:00   79K  \n[DIR] doipubmed/                         20-Aug-2007 18:03    -   \n[   ] dot2texi.zip                       07-May-2012 19:21  274K  \n[DIR] dot2texi/                          07-May-2012 19:21    -   \n[   ] dotarrow.zip                       12-Feb-2008 15:56   77K  \n[DIR] dotarrow/                          12-Feb-2008 16:03    -   \n[   ] dotseqn.zip                        23-Feb-2010 23:32  134K  \n[DIR] dotseqn/                           23-Feb-2010 23:33    -   \n[   ] dottex.zip                         22-Aug-2007 13:31   93K  \n[DIR] dottex/                            22-Aug-2007 13:31    -   \n[   ] download.zip                       25-May-2013 01:16  146K  \n[DIR] download/                          25-May-2013 02:03    -   \n[   ] dox.zip                            06-Dec-2017 21:46  140K  \n[DIR] dox/                               06-Dec-2017 21:46    -   \n[   ] dpfloat.zip                        23-Feb-2010 23:58  191K  \n[DIR] dpfloat/                           24-Feb-2010 02:03    -   \n[   ] dprogress.zip                      21-Feb-2008 17:20   67K  \n[DIR] dprogress/                         21-Feb-2008 17:23    -   \n[   ] dps.zip                            18-Oct-2006 18:36  127K  \n[DIR] dps/                               18-Oct-2006 18:43    -   \n[   ] drac.zip                           14-Aug-2008 13:31  711K  \n[DIR] drac/                              14-Aug-2008 13:33    -   \n[   ] draftcopy.zip                      10-Dec-2007 13:51  125K  \n[DIR] draftcopy/                         10-Dec-2007 13:53    -   \n[   ] draftfigure.zip                    20-Jul-2017 04:40  162K  \n[DIR] draftfigure/                       20-Jul-2017 04:40    -   \n[   ] draftmark.zip                      03-Nov-2009 14:53  247K  \n[DIR] draftmark/                         03-Nov-2009 15:03    -   \n[   ] draftwatermark.zip                 10-Jun-2015 19:26   97K  \n[DIR] draftwatermark/                    10-Jun-2015 19:26    -   \n[   ] dramatist.zip                      19-Dec-2014 05:43  444K  \n[DIR] dramatist/                         19-Dec-2014 05:43    -   \n[   ] drawmatrix.zip                     05-Jun-2017 22:36  309K  \n[DIR] drawmatrix/                        05-Jun-2017 22:36    -   \n[   ] drawstack.zip                      19-Dec-2012 17:46  105K  \n[DIR] drawstack/                         19-Dec-2012 17:46    -   \n[   ] droit-fr.zip                       20-Feb-2016 19:58  292K  \n[DIR] droit-fr/                          20-Feb-2016 19:58    -   \n[   ] dropping.zip                       23-Dec-2005 15:14   92K  \n[DIR] dropping/                          23-Jan-2006 08:43    -   \n[   ] drs.zip                            03-Jul-2010 20:20  102K  \n[DIR] drs/                               03-Jul-2010 20:23    -   \n[   ] dtk.zip                            07-Jun-2017 13:41  109K  \n[DIR] dtk/                               07-Jun-2017 13:41    -   \n[   ] dtxdescribe.zip                    30-Mar-2018 10:38  604K  \n[DIR] dtxdescribe/                       30-Mar-2018 10:38    -   \n[   ] ducksay.zip                        30-Oct-2017 08:07  228K  \n[DIR] ducksay/                           30-Oct-2017 08:07    -   \n[   ] duckuments.zip                     19-Mar-2018 22:43  727K  \n[DIR] duckuments/                        19-Mar-2018 22:43    -   \n[   ] duerer-latex.zip                   23-Sep-2006 14:35  149K  \n[DIR] duerer-latex/                      23-Sep-2006 14:43    -   \n[   ] dvdcoll.zip                        30-Apr-2008 11:48  296K  \n[DIR] dvdcoll/                           30-Apr-2008 11:48    -   \n[   ] dvgloss.zip                        13-Feb-2013 09:12  208K  \n[DIR] dvgloss/                           13-Feb-2013 09:12    -   \n[   ] dynamicnumber.zip                  27-Oct-2015 13:34  159K  \n[DIR] dynamicnumber/                     27-Oct-2015 13:34    -   \n[   ] dyntree.zip                        20-Aug-2006 02:25  135K  \n[DIR] dyntree/                           20-Aug-2006 02:33    -   \n[   ] ean13isbn.zip                      22-Jun-2008 19:59  310K  \n[DIR] ean13isbn/                         22-Jun-2008 20:03    -   \n[   ] easy-todo.zip                      14-Jan-2014 11:41  137K  \n[DIR] easy-todo/                         14-Jan-2014 11:43    -   \n[   ] easy.zip                           25-Sep-2012 14:41  630K  \n[DIR] easy/                              17-Jun-2009 12:03    -   \n[   ] easyfig.zip                        30-Mar-2018 20:41  176K  \n[DIR] easyfig/                           30-Mar-2018 20:41    -   \n[   ] easyformat.zip                     09-Jun-2017 19:18   51K  \n[DIR] easyformat/                        09-Jun-2017 19:18    -   \n[   ] easylist.zip                       12-Jan-2014 16:33  597K  \n[DIR] easylist/                          12-Jan-2014 16:43    -   \n[   ] easyreview.zip                     11-Sep-2015 20:51  325K  \n[DIR] easyreview/                        11-Sep-2015 20:51    -   \n[   ] ebezier.zip                        01-Mar-2005 10:48  304K  \n[DIR] ebezier/                           01-Mar-2005 10:47    -   \n[   ] ebook.zip                          22-Mar-2013 10:45  1.8K  \n[DIR] ebook/                             22-Mar-2013 10:53    -   \n[   ] ebproof.zip                        17-May-2017 18:27  234K  \n[DIR] ebproof/                           17-May-2017 18:27    -   \n[   ] ebsthesis.zip                      05-Jan-2007 00:41  254K  \n[DIR] ebsthesis/                         05-Jan-2007 02:03    -   \n[   ] ecards.zip                         23-Sep-2016 14:29  3.0M  \n[DIR] ecards/                            23-Sep-2016 14:29    -   \n[   ] ecclesiastic.zip                   21-Aug-2015 17:50  368K  \n[DIR] ecclesiastic/                      21-Aug-2015 17:50    -   \n[   ] eclbip.zip                         01-Jun-2008 23:12   34K  \n[DIR] eclbip/                            01-Jun-2008 22:13    -   \n[   ] econometrics.zip                   15-Jan-2016 12:53  190K  \n[DIR] econometrics/                      15-Jan-2016 12:53    -   \n[   ] ecv.zip                            23-Dec-2011 13:48  342K  \n[DIR] ecv/                               23-Dec-2011 13:48    -   \n[   ] ed.zip                             29-Jan-2012 15:53  294K  \n[DIR] ed/                                29-Jan-2012 15:53    -   \n[   ] edfnotes.zip                       27-Feb-2011 18:59  302K  \n[DIR] edfnotes/                          27-Feb-2011 18:59    -   \n[   ] edmargin.zip                       05-Sep-2012 08:34  307K  \n[DIR] edmargin/                          05-Sep-2012 08:43    -   \n[   ] ednotes.zip                        03-Apr-2008 15:10  1.0M  \n[DIR] ednotes/                           03-Apr-2008 15:10    -   \n[   ] eemeir.zip                         20-Feb-2007 01:58  142K  \n[DIR] eemeir/                            20-Feb-2007 02:03    -   \n[   ] eepic.zip                          09-Jul-2009 13:01  116K  \n[DIR] eepic/                             09-Jul-2009 13:03    -   \n[   ] efbox.zip                          20-Mar-2014 00:29  146K  \n[DIR] efbox/                             20-Mar-2014 02:03    -   \n[   ] egameps.zip                        21-Sep-2006 19:22  143K  \n[DIR] egameps/                           21-Sep-2006 19:23    -   \n[   ] egplot.zip                         30-Nov-2010 13:49  481K  \n[DIR] egplot/                            30-Nov-2010 13:53    -   \n[   ] eiad.zip                           30-Apr-2005 15:58  9.3K  \n[DIR] eiad/                              01-Feb-2005 20:43    -   \n[   ] ejpecp.zip                         06-Sep-2016 13:12  299K  \n[DIR] ejpecp/                            06-Sep-2016 13:12    -   \n[   ] ekaia.zip                          25-Nov-2016 17:16  528K  \n[DIR] ekaia/                             25-Nov-2016 17:16    -   \n[   ] elbioimp.zip                       18-Mar-2011 14:25  291K  \n[DIR] elbioimp/                          18-Mar-2011 14:25    -   \n[   ] eledform.zip                       13-Aug-2015 14:16  130K  \n[DIR] eledform/                          13-Aug-2015 14:16    -   \n[   ] eledmac.zip                        25-Sep-2017 19:01  2.0M  \n[DIR] eledmac/                           25-Sep-2017 19:01    -   \n[   ] elements.zip                       31-Jan-2018 15:53  408K  \n[DIR] elements/                          31-Jan-2018 15:53    -   \n[   ] ellipsis.zip                       30-Apr-2005 15:58   98K  \n[DIR] ellipsis/                          01-Feb-2005 20:43    -   \n[   ] elmath.zip                         30-Apr-2005 15:58   66K  \n[DIR] elmath/                            01-Feb-2005 20:43    -   \n[   ] elocalloc.zip                      15-Dec-2016 10:21  151K  \n[DIR] elocalloc/                         15-Dec-2016 10:21    -   \n[   ] elpres.zip                         24-Jan-2018 05:04  211K  \n[DIR] elpres/                            24-Jan-2018 05:04    -   \n[   ] elsarticle.zip                     18-Sep-2009 13:33  1.0M  \n[DIR] elsarticle/                        18-Sep-2009 13:43    -   \n[   ] elteikthesis.zip                   17-May-2011 17:07  3.3M  \n[DIR] elteikthesis/                      17-May-2011 17:07    -   \n[   ] eltex.zip                          23-Jun-2009 15:40  194K  \n[DIR] eltex/                             23-Jun-2009 15:40    -   \n[   ] elzcards.zip                       10-Jul-2017 13:28  167K  \n[DIR] elzcards/                          10-Jul-2017 13:28    -   \n[   ] emarks.zip                         01-Nov-2011 20:17  2.2M  \n[DIR] emarks/                            01-Nov-2011 20:23    -   \n[   ] embedall.zip                       14-Oct-2013 15:46  154K  \n[DIR] embedall/                          14-Oct-2013 15:53    -   \n[   ] embrac.zip                         06-Jul-2017 13:07  461K  \n[DIR] embrac/                            06-Jul-2017 13:07    -   \n[   ] emf.zip                            09-Sep-2016 11:08  318K  \n[DIR] emf/                               09-Sep-2016 11:08    -   \n[   ] emisa.zip                          24-Feb-2018 13:13  878K  \n[DIR] emisa/                             24-Feb-2018 13:13    -   \n[   ] emp.zip                            06-Aug-2011 23:17  225K  \n[DIR] emp/                               06-Aug-2011 23:23    -   \n[   ] emptypage.zip                      30-Apr-2010 19:00   52K  \n[DIR] emptypage/                         30-Apr-2010 19:03    -   \n[   ] emulateapj.zip                     05-Dec-2012 13:28  165K  \n[DIR] emulateapj/                        05-Dec-2012 13:33    -   \n[   ] endfloat.zip                       24-Mar-2018 22:18  206K  \n[DIR] endfloat/                          24-Mar-2018 22:18    -   \n[   ] endheads.zip                       08-Apr-2017 06:54  230K  \n[DIR] endheads/                          08-Apr-2017 06:54    -   \n[   ] endiagram.zip                      29-Jun-2014 01:02  638K  \n[DIR] endiagram/                         29-Jun-2014 02:03    -   \n[   ] endnotes.zip                       24-Feb-2010 18:33  259K  \n[DIR] endnotes/                          24-Feb-2010 18:43    -   \n[   ] engpron.zip                        28-Dec-2009 11:22  2.2M  \n[DIR] engpron/                           28-Dec-2009 11:23    -   \n[   ] engrec.zip                         07-May-2008 21:59  272K  \n[DIR] engrec/                            07-May-2008 22:03    -   \n[   ] engtlc.zip                         18-Dec-2012 12:09  780K  \n[DIR] engtlc/                            18-Dec-2012 12:13    -   \n[   ] enotez.zip                         24-Apr-2017 19:46  462K  \n[DIR] enotez/                            24-Apr-2017 19:46    -   \n[   ] enumitem-zref.zip                  19-Feb-2011 16:04  719K  \n[DIR] enumitem-zref/                     19-Feb-2011 16:13    -   \n[   ] enumitem.zip                       28-Sep-2011 17:35  348K  \n[DIR] enumitem/                          28-Sep-2011 17:35    -   \n[   ] envbig.zip                         11-Nov-2008 20:14  1.3K  \n[DIR] envbig/                            11-Nov-2008 20:23    -   \n[   ] environ.zip                        04-May-2014 12:13  158K  \n[DIR] environ/                           04-May-2014 12:23    -   \n[   ] envlab.zip                         02-Jun-2008 00:08  363K  \n[DIR] envlab/                            01-Jun-2008 23:13    -   \n[   ] epic.zip                           09-Jul-2009 13:00  179K  \n[DIR] epic/                              09-Jul-2009 13:03    -   \n[   ] epigraph.zip                       02-Sep-2009 17:07  170K  \n[DIR] epigraph/                          02-Sep-2009 17:13    -   \n[   ] epsdice.zip                        26-Sep-2012 17:56   72K  \n[DIR] epsdice/                           15-Feb-2007 14:08    -   \n[   ] epspdfconversion.zip               02-Jun-2010 10:37  416K  \n[DIR] epspdfconversion/                  02-Jun-2010 10:37    -   \n[   ] eq-save.zip                        27-Aug-2017 07:10  271K  \n[DIR] eq-save/                           27-Aug-2017 07:10    -   \n[   ] eq2db.zip                          02-Jan-2016 14:26  177K  \n[DIR] eq2db/                             02-Jan-2016 14:26    -   \n[   ] eqell.zip                          08-Jun-2011 08:22  179K  \n[DIR] eqell/                             08-Jun-2011 08:22    -   \n[   ] eqexam.zip                         02-Mar-2018 17:07  2.8M  \n[DIR] eqexam/                            02-Mar-2018 17:07    -   \n[   ] eqlist.zip                         26-Nov-2013 21:34   71K  \n[DIR] eqlist/                            26-Nov-2013 21:34    -   \n[   ] eqnalign.zip                       19-Feb-2017 20:45  285K  \n[DIR] eqnalign/                          19-Feb-2017 20:45    -   \n[   ] eqnarray.zip                       02-Dec-2010 01:04  106K  \n[DIR] eqnarray/                          02-Dec-2010 02:03    -   \n[   ] eqnnumwarn.zip                     09-Oct-2017 19:55   94K  \n[DIR] eqnnumwarn/                        09-Oct-2017 19:55    -   \n[   ] eqparbox.zip                       04-Sep-2017 06:01  226K  \n[DIR] eqparbox/                          04-Sep-2017 06:01    -   \n[   ] erdc.zip                           24-Jul-2009 22:08  706K  \n[DIR] erdc/                              24-Jul-2009 22:13    -   \n[   ] errata.zip                         09-Nov-2007 10:40  153K  \n[DIR] errata/                            09-Nov-2007 10:40    -   \n[   ] esami.zip                          14-Mar-2018 14:07  1.5M  \n[DIR] esami/                             14-Mar-2018 14:07    -   \n[   ] esdiff.zip                         13-Feb-2011 18:27   85K  \n[DIR] esdiff/                            13-Feb-2011 18:33    -   \n[   ] esint.zip                          25-Oct-2006 19:28  108K  \n[DIR] esint/                             25-Oct-2006 19:43    -   \n[   ] esk.zip                            05-May-2010 09:06  424K  \n[DIR] esk/                               05-May-2010 09:06    -   \n[   ] eskd.zip                           30-Apr-2005 15:59  297K  \n[DIR] eskd/                              01-Feb-2005 20:43    -   \n[   ] eskdx.zip                          13-May-2011 19:47  531K  \n[DIR] eskdx/                             13-May-2011 19:53    -   \n[   ] eso-pic.zip                        22-Jul-2015 20:20  255K  \n[DIR] eso-pic/                           22-Jul-2015 20:20    -   \n[   ] estcpmm.zip                        04-Mar-2010 23:17  360K  \n[DIR] estcpmm/                           04-Mar-2010 23:23    -   \n[   ] esvect.zip                         08-Nov-2013 16:26  137K  \n[DIR] esvect/                            08-Nov-2013 16:26    -   \n[   ] etaremune.zip                      01-Jun-2005 09:22   80K  \n[DIR] etaremune/                         01-Jun-2005 09:22    -   \n[   ] etdipa.zip                         22-Feb-2015 16:09  1.7M  \n[DIR] etdipa/                            22-Feb-2015 16:09    -   \n[   ] etex-pkg.zip                       01-Aug-2016 18:30  6.3K  \n[DIR] etex-pkg/                          01-Aug-2016 18:30    -   \n[   ] etextools.zip                      14-Dec-2010 01:38  1.0M  \n[DIR] etextools/                         14-Dec-2010 02:03    -   \n[DIR] ethiop/                            05-Oct-2004 09:09    -   \n[   ] etoc.zip                           23-Feb-2018 23:24  1.3M  \n[DIR] etoc/                              23-Feb-2018 23:24    -   \n[   ] etoolbox.zip                       11-Feb-2018 09:55  238K  \n[DIR] etoolbox/                          11-Feb-2018 09:55    -   \n[   ] euenc.zip                          18-Sep-2010 19:54  147K  \n[DIR] euenc/                             18-Sep-2010 20:03    -   \n[   ] eukdate.zip                        17-Mar-2009 19:27  113K  \n[DIR] eukdate/                           17-Mar-2009 19:33    -   \n[   ] euler.zip                          28-Feb-2010 17:31  241K  \n[DIR] euler/                             28-Feb-2010 17:33    -   \n[   ] euproposal.zip                     15-Apr-2016 14:28  1.3M  \n[DIR] euproposal/                        15-Apr-2016 14:28    -   \n[   ] euro.zip                           07-Mar-2005 16:23  215K  \n[DIR] euro/                              07-Mar-2005 16:21    -   \n[   ] eurofont.zip                       01-Oct-2007 15:46   61K  \n[DIR] eurofont/                          01-Feb-2005 20:43    -   \n[   ] europasscv.zip                     19-Nov-2017 23:23  484K  \n[DIR] europasscv/                        19-Nov-2017 23:23    -   \n[   ] europecv.zip                       27-Jun-2014 08:43  765K  \n[DIR] europecv/                          27-Jun-2014 08:53    -   \n[DIR] europs/                            03-Apr-2010 22:03    -   \n[DIR] eurosans/                          28-Feb-2010 19:13    -   \n[   ] everyhook.zip                      26-Nov-2014 21:11  120K  \n[DIR] everyhook/                         26-Nov-2014 21:11    -   \n[   ] everypage.zip                      19-Feb-2008 19:19   20K  \n[DIR] everypage/                         19-Feb-2008 19:23    -   \n[   ] exam-n.zip                         20-Dec-2016 13:07  1.0M  \n[DIR] exam-n/                            20-Dec-2016 13:07    -   \n[   ] exam.zip                           17-Dec-2017 18:50  564K  \n[DIR] exam/                              17-Dec-2017 18:50    -   \n[   ] examdesign.zip                     06-Sep-2006 01:36  412K  \n[DIR] examdesign/                        06-Sep-2006 02:03    -   \n[   ] examplep.zip                       04-Feb-2010 01:43  434K  \n[DIR] examplep/                          04-Feb-2010 02:03    -   \n[   ] exams.zip                          23-May-2011 10:44   20K  \n[DIR] exams/                             23-May-2011 10:53    -   \n[   ] exceltex.zip                       08-May-2006 22:03   15K  \n[DIR] exceltex/                          08-May-2006 22:13    -   \n[   ] excludeonly.zip                    28-Feb-2010 19:16  214K  \n[DIR] excludeonly/                       28-Feb-2010 19:23    -   \n[   ] exercise.zip                       21-Oct-2014 17:31  325K  \n[DIR] exercise/                          21-Oct-2014 17:31    -   \n[   ] exercisebank.zip                   01-Apr-2018 10:18  157K  \n[DIR] exercisebank/                      01-Apr-2018 10:18    -   \n[   ] exercises.zip                      19-Sep-2015 20:42  360K  \n[DIR] exercises/                         19-Sep-2015 20:42    -   \n[   ] exp-testopt.zip                    06-Mar-2009 15:18   96K  \n[DIR] exp-testopt/                       06-Mar-2009 15:18    -   \n[   ] expdlist.zip                       23-Jun-2008 17:20  154K  \n[DIR] expdlist/                          23-Jun-2008 16:23    -   \n[   ] expex.zip                          26-May-2017 16:32  487K  \n[DIR] expex/                             26-May-2017 16:32    -   \n[   ] export.zip                         11-Jul-2012 13:44  286K  \n[DIR] export/                            11-Jul-2012 13:53    -   \n[   ] exsheets.zip                       09-Feb-2017 10:12  717K  \n[DIR] exsheets/                          09-Feb-2017 10:12    -   \n[   ] exsol.zip                          05-Jun-2016 07:59  663K  \n[DIR] exsol/                             05-Jun-2016 07:59    -   \n[   ] extarrows.zip                      15-May-2008 15:19   29K  \n[DIR] extarrows/                         15-May-2008 15:23    -   \n[   ] extpfeil.zip                       31-Oct-2009 19:35  118K  \n[DIR] extpfeil/                          31-Oct-2009 19:43    -   \n[   ] extract.zip                        08-May-2005 18:01  202K  \n[DIR] extract/                           08-May-2005 18:01    -   \n[   ] extsizes.zip                       28-Feb-2010 19:12  224K  \n[DIR] extsizes/                          28-Feb-2010 19:13    -   \n[   ] fac.zip                            30-Apr-2005 15:59   22K  \n[DIR] fac/                               01-Feb-2005 20:43    -   \n[   ] facsimile.zip                      30-Apr-2005 15:59   40K  \n[DIR] facsimile/                         01-Feb-2005 20:43    -   \n[   ] factura.zip                        13-Mar-2018 17:09  2.8M  \n[DIR] factura/                           13-Mar-2018 17:09    -   \n[   ] faktor.zip                         11-Apr-2006 18:44   85K  \n[DIR] faktor/                            11-Apr-2006 19:13    -   \n[   ] famt.zip                           10-May-2012 11:32  731K  \n[DIR] famt/                              10-May-2012 11:32    -   \n[   ] fancybox.zip                       15-May-2010 22:17  280K  \n[DIR] fancybox/                          15-May-2010 22:23    -   \n[   ] fancyhandout.zip                   22-Jan-2018 19:46   73K  \n[DIR] fancyhandout/                      22-Jan-2018 19:46    -   \n[   ] fancyhdr.zip                       30-Jun-2017 08:22  396K  \n[DIR] fancyhdr/                          30-Jun-2017 08:22    -   \n[   ] fancylabel.zip                     23-Feb-2018 21:23  234K  \n[DIR] fancylabel/                        23-Feb-2018 21:23    -   \n[   ] fancynum.zip                       08-Oct-2006 10:52   64K  \n[DIR] fancynum/                          16-Aug-2008 14:45    -   \n[   ] fancypar.zip                       26-Sep-2012 17:58  114K  \n[DIR] fancypar/                          25-Apr-2010 21:53    -   \n[   ] fancyref.zip                       05-Dec-2006 14:33  123K  \n[DIR] fancyref/                          05-Dec-2006 14:43    -   \n[   ] fancyslides.zip                    12-Feb-2015 20:41  3.8M  \n[DIR] fancyslides/                       12-Feb-2015 20:41    -   \n[   ] fancytabs.zip                      27-Jun-2016 10:01  184K  \n[DIR] fancytabs/                         27-Jun-2016 10:01    -   \n[   ] fancytooltips.zip                  26-Sep-2012 18:02  1.5M  \n[DIR] fancytooltips/                     03-Jun-2012 19:13    -   \n[   ] fancyvrb.zip                       25-May-2010 20:13  482K  \n[DIR] fancyvrb/                          25-May-2010 20:13    -   \n[   ] fax.zip                            06-Oct-2006 02:00   64K  \n[DIR] fax/                               16-Aug-2008 14:45    -   \n[   ] fbithesis.zip                      07-Feb-2011 02:44  816K  \n[DIR] fbithesis/                         07-Feb-2011 02:44    -   \n[   ] fc_arith.zip                       22-Mar-2017 16:19  1.0M  \n[DIR] fc_arith/                          22-Mar-2017 16:19    -   \n[   ] fcavtex.zip                        07-Aug-2015 07:16  342K  \n[DIR] fcavtex/                           07-Aug-2015 07:16    -   \n[   ] fcltxdoc.zip                       01-Nov-2011 17:37  649K  \n[DIR] fcltxdoc/                          01-Nov-2011 17:43    -   \n[   ] fcolumn.zip                        27-Sep-2015 21:04  255K  \n[DIR] fcolumn/                           27-Sep-2015 21:04    -   \n[   ] fei.zip                            02-Mar-2018 21:15  301K  \n[DIR] fei/                               02-Mar-2018 21:15    -   \n[   ] fetchbibpes.zip                    10-Jan-2017 14:42  502K  \n[DIR] fetchbibpes/                       10-Jan-2017 14:42    -   \n[   ] fetchcls.zip                       08-Sep-2017 17:57  124K  \n[DIR] fetchcls/                          08-Sep-2017 17:57    -   \n[   ] feupphdteses.zip                   17-Jun-2013 13:39  226K  \n[DIR] feupphdteses/                      17-Jun-2013 13:43    -   \n[DIR] feyn/                              03-Nov-2017 16:40    -   \n[   ] feynmf.zip                         28-Feb-2010 19:35  542K  \n[DIR] feynmf/                            28-Feb-2010 19:43    -   \n[   ] feynmp-auto.zip                    03-May-2013 17:16  370K  \n[DIR] feynmp-auto/                       03-May-2013 17:16    -   \n[   ] ffslides.zip                       19-Nov-2015 15:50  2.7M  \n[DIR] ffslides/                          19-Nov-2015 15:50    -   \n[   ] fgruler.zip                        16-Jan-2017 15:40  253K  \n[DIR] fgruler/                           16-Jan-2017 15:40    -   \n[   ] fifo-stack.zip                     25-Mar-2014 13:29  252K  \n[DIR] fifo-stack/                        25-Mar-2014 13:29    -   \n[   ] figbib.zip                         30-Apr-2005 15:59  138K  \n[DIR] figbib/                            23-Jan-2006 08:43    -   \n[   ] figsize.zip                        30-Apr-2005 15:59   90K  \n[DIR] figsize/                           01-Feb-2005 20:43    -   \n[   ] filecontents.zip                   09-Oct-2011 16:36  237K  \n[DIR] filecontents/                      09-Oct-2011 16:36    -   \n[   ] filecontentsdef.zip                20-Sep-2016 11:26   81K  \n[DIR] filecontentsdef/                   20-Sep-2016 11:26    -   \n[   ] filedate.zip                       27-Mar-2013 15:00  562K  \n[DIR] filedate/                          27-Mar-2013 15:03    -   \n[   ] filehook.zip                       13-Oct-2011 08:50  264K  \n[DIR] filehook/                          13-Oct-2011 08:53    -   \n[   ] fileinfo.zip                       02-Dec-2012 12:47  1.0M  \n[DIR] fileinfo/                          02-Dec-2012 12:47    -   \n[   ] filemod.zip                        20-Sep-2011 18:39  276K  \n[DIR] filemod/                           20-Sep-2011 18:39    -   \n[   ] fink.zip                           19-Oct-2011 13:13   89K  \n[DIR] fink/                              19-Oct-2011 13:13    -   \n[   ] finstrut.zip                       14-Mar-2011 19:12  180K  \n[DIR] finstrut/                          14-Mar-2011 19:12    -   \n[   ] fitbox.zip                         16-Aug-2015 21:39  395K  \n[DIR] fitbox/                            16-Aug-2015 21:39    -   \n[   ] fithesis.zip                       12-Feb-2018 00:17   31M  \n[DIR] fithesis/                          12-Feb-2018 00:17    -   \n[   ] fitr.zip                           09-Apr-2016 17:20  677K  \n[DIR] fitr/                              09-Apr-2016 17:20    -   \n[   ] fix2col.zip                        03-Nov-2015 15:12  212K  \n[DIR] fix2col/                           03-Nov-2015 21:18    -   \n[   ] fixcmex.zip                        10-Nov-2015 19:12  196K  \n[DIR] fixcmex/                           10-Nov-2015 19:12    -   \n[   ] fixfoot.zip                        20-Feb-2010 00:28   53K  \n[DIR] fixfoot/                           20-Feb-2010 02:03    -   \n[   ] fixltxhyph.zip                     02-Apr-2012 21:13  393K  \n[DIR] fixltxhyph/                        02-Apr-2012 21:13    -   \n[   ] fixme.zip                          05-Mar-2017 21:18  367K  \n[DIR] fixme/                             05-Mar-2017 21:18    -   \n[   ] fixmetodonotes.zip                 28-Apr-2013 23:21  5.6K  \n[DIR] fixmetodonotes/                    28-Apr-2013 23:21    -   \n[   ] fjodor.zip                         26-Oct-2010 18:57  446K  \n[DIR] fjodor/                            26-Oct-2010 19:03    -   \n[   ] flabels.zip                        28-Feb-2010 21:41  346K  \n[DIR] flabels/                           28-Feb-2010 21:43    -   \n[   ] flacards.zip                       16-Jan-2010 13:19  159K  \n[DIR] flacards/                          16-Jan-2010 13:23    -   \n[   ] flagderiv.zip                      26-Aug-2005 18:03  194K  \n[DIR] flagderiv/                         26-Aug-2005 18:13    -   \n[   ] flashcards.zip                     14-Aug-2010 01:33  139K  \n[DIR] flashcards/                        14-Aug-2010 02:03    -   \n[   ] flashmovie.zip                     17-Nov-2010 20:16  1.3M  \n[DIR] flashmovie/                        17-Nov-2010 20:23    -   \n[   ] fldigigal.zip                      29-Dec-2010 18:15  6.1M  \n[DIR] fldigigal/                         29-Dec-2010 18:23    -   \n[   ] flipbook.zip                       07-Mar-2012 15:36  511K  \n[DIR] flipbook/                          07-Mar-2012 15:36    -   \n[   ] flippdf.zip                        03-Jul-2006 16:16   15K  \n[DIR] flippdf/                           03-Jul-2006 16:23    -   \n[   ] float.zip                          05-Dec-2006 13:14  125K  \n[DIR] float/                             05-Dec-2006 13:23    -   \n[   ] floatflt.zip                       29-Feb-2012 15:31  305K  \n[DIR] floatflt/                          29-Feb-2012 15:33    -   \n[   ] floatrow.zip                       22-Jun-2009 22:09  1.4M  \n[DIR] floatrow/                          03-Apr-2010 22:03    -   \n[   ] flowfram.zip                       30-Sep-2014 16:18  2.0M  \n[DIR] flowfram/                          30-Sep-2014 16:18    -   \n[   ] fltpage.zip                        09-Aug-2006 13:32   80K  \n[DIR] fltpage/                           09-Aug-2006 13:03    -   \n[   ] fltpoint.zip                       30-Apr-2005 16:00  191K  \n[DIR] fltpoint/                          01-Feb-2005 20:43    -   \n[   ] fmp.zip                            30-Apr-2005 16:00  137K  \n[DIR] fmp/                               01-Feb-2005 20:43    -   \n[   ] fmtcount.zip                       27-Dec-2017 23:38  464K  \n[DIR] fmtcount/                          27-Dec-2017 23:38    -   \n[   ] fn2end.zip                         26-Sep-2012 18:05   24K  \n[DIR] fn2end/                            29-Dec-2008 15:53    -   \n[   ] fnbreak.zip                        02-Jan-2012 14:00  205K  \n[DIR] fnbreak/                           02-Jan-2012 14:00    -   \n[   ] fncychap.zip                       26-Sep-2012 18:08  486K  \n[DIR] fncychap/                          10-Dec-2010 10:23    -   \n[   ] fncylab.zip                        07-Mar-2010 16:47  199K  \n[DIR] fncylab/                           07-Mar-2010 16:53    -   \n[   ] fnpara.zip                         11-Mar-2012 01:01  173K  \n[DIR] fnpara/                            11-Mar-2012 02:03    -   \n[   ] fnpct.zip                          14-Apr-2016 21:15  579K  \n[DIR] fnpct/                             14-Apr-2016 21:15    -   \n[   ] fnspe.zip                          20-Sep-2017 10:19  171K  \n[DIR] fnspe/                             20-Sep-2017 10:19    -   \n[   ] fnumprint.zip                      19-Feb-2013 09:18  251K  \n[DIR] fnumprint/                         19-Feb-2013 09:18    -   \n[   ] foilhtml.zip                       30-Apr-2005 16:00   18K  \n[DIR] foilhtml/                          01-Feb-2005 20:43    -   \n[   ] foiltex.zip                        29-Jan-2008 18:25  372K  \n[DIR] foiltex/                           29-Jan-2008 18:33    -   \n[   ] fontaxes.zip                       24-Mar-2014 07:19  124K  \n[DIR] fontaxes/                          24-Mar-2014 07:19    -   \n[   ] fontspec.zip                       09-Nov-2017 13:08  1.3M  \n[DIR] fontspec/                          09-Nov-2017 13:08    -   \n[   ] fonttable.zip                      14-Jul-2017 12:44  316K  \n[DIR] fonttable/                         14-Jul-2017 12:44    -   \n[   ] footbib.zip                        20-Feb-2010 20:54  218K  \n[DIR] footbib/                           20-Feb-2010 21:03    -   \n[   ] footmisc.zip                       06-Jun-2011 16:27  336K  \n[DIR] footmisc/                          06-Jun-2011 16:33    -   \n[   ] footmisx.zip                       01-Dec-2016 22:39   21K  \n[DIR] footmisx/                          01-Dec-2016 22:39    -   \n[   ] footnotebackref.zip                01-Jul-2012 15:34  111K  \n[DIR] footnotebackref/                   01-Jul-2012 15:34    -   \n[   ] footnotehyper.zip                  23-Jan-2018 22:18   69K  \n[DIR] footnotehyper/                     23-Jan-2018 22:18    -   \n[   ] footnoterange.zip                  19-Feb-2012 14:44  381K  \n[DIR] footnoterange/                     19-Feb-2012 14:44    -   \n[   ] footnpag.zip                       06-Jan-2007 01:00   69K  \n[DIR] footnpag/                          16-Aug-2008 14:45    -   \n[   ] forarray.zip                       22-Jun-2008 11:31  273K  \n[DIR] forarray/                          22-Jun-2008 11:31    -   \n[   ] foreign.zip                        26-Sep-2012 14:31   87K  \n[DIR] foreign/                           26-Sep-2012 14:31    -   \n[   ] forloop.zip                        19-Sep-2006 14:23   72K  \n[DIR] forloop/                           19-Sep-2006 14:43    -   \n[   ] forms16be.zip                      30-Aug-2017 17:12  1.3M  \n[DIR] forms16be/                         30-Aug-2017 17:12    -   \n[   ] formula.zip                        28-Feb-2010 21:57  340K  \n[DIR] formula/                           28-Feb-2010 22:03    -   \n[   ] formular.zip                       17-Jun-2005 12:02  140K  \n[DIR] formular/                          17-Jun-2005 12:02    -   \n[   ] fouridx.zip                        21-Nov-2013 22:42  208K  \n[DIR] fouridx/                           21-Nov-2013 22:42    -   \n[   ] fp.zip                             30-Apr-2005 16:13   33K  \n[DIR] fp/                                30-Apr-2005 16:13    -   \n[   ] fragments.zip                      20-Oct-2008 21:33  2.6K  \n[DIR] fragments/                         20-Oct-2008 20:43    -   \n[DIR] fraktur/                           03-Apr-2010 23:06    -   \n[   ] framed.zip                         01-Jun-2012 12:44  240K  \n[DIR] framed/                            01-Jun-2012 12:53    -   \n[   ] frankenstein.zip                   25-Nov-2006 01:00  2.1M  \n[DIR] frankenstein/                      02-Mar-2007 20:08    -   \n[DIR] frcursive/                         09-Nov-2011 16:03    -   \n[   ] frege.zip                          15-Aug-2012 12:04  146K  \n[DIR] frege/                             15-Aug-2012 12:04    -   \n[   ] fribrief.zip                       30-Apr-2005 16:00   11K  \n[DIR] fribrief/                          01-Feb-2005 20:43    -   \n[   ] frletter.zip                       27-Oct-2007 16:23  1.9K  \n[DIR] frletter/                          27-Oct-2007 16:33    -   \n[   ] frontespizio.zip                   21-Sep-2011 15:36  709K  \n[DIR] frontespizio/                      21-Sep-2011 15:43    -   \n[   ] ftcap.zip                          28-Feb-2010 22:56  207K  \n[DIR] ftcap/                             28-Feb-2010 23:03    -   \n[   ] ftnxtra.zip                        04-Apr-2013 15:04   26K  \n[DIR] ftnxtra/                           04-Apr-2013 15:13    -   \n[   ] fullblck.zip                       12-Sep-2008 12:18   42K  \n[DIR] fullblck/                          12-Sep-2008 11:23    -   \n[   ] fullminipage.zip                   07-Jul-2014 17:21  253K  \n[DIR] fullminipage/                      07-Jul-2014 17:23    -   \n[   ] fullpict.zip                       30-Apr-2005 16:00  5.2K  \n[DIR] fullpict/                          05-Jan-2007 22:33    -   \n[   ] fullwidth.zip                      28-Nov-2011 11:47  281K  \n[DIR] fullwidth/                         28-Nov-2011 11:47    -   \n[   ] functan.zip                        30-Apr-2005 16:00  155K  \n[DIR] functan/                           01-Feb-2005 20:43    -   \n[DIR] fundus/                            16-Jul-2012 11:12    -   \n[   ] fvextra.zip                        09-Jul-2017 23:27  721K  \n[DIR] fvextra/                           09-Jul-2017 23:27    -   \n[   ] fwlw.zip                           26-Sep-2012 18:22   39K  \n[DIR] fwlw/                              28-Feb-2011 15:03    -   \n[   ] g-brief.zip                        26-Jan-2011 09:55  148K  \n[DIR] g-brief/                           26-Jan-2011 09:55    -   \n[   ] gaceta.zip                         16-May-2008 14:06  210K  \n[DIR] gaceta/                            16-May-2008 14:13    -   \n[   ] galois.zip                         22-Mar-2006 14:36   94K  \n[DIR] galois/                            22-Mar-2006 14:43    -   \n[   ] gamebook.zip                       29-Nov-2011 16:31  225K  \n[DIR] gamebook/                          29-Nov-2011 16:31    -   \n[   ] gatech-thesis.zip                  26-Sep-2012 18:17  176K  \n[DIR] gatech-thesis/                     26-Jul-2010 16:53    -   \n[   ] gauss.zip                          26-Oct-2011 16:38  131K  \n[DIR] gauss/                             26-Oct-2011 16:38    -   \n[   ] gb4e.zip                           03-Jul-2010 20:04  156K  \n[DIR] gb4e/                              03-Jul-2010 20:13    -   \n[   ] gcard.zip                          22-Aug-2007 12:38  128K  \n[DIR] gcard/                             22-Aug-2007 11:43    -   \n[   ] gender.zip                         08-Mar-2015 07:36  307K  \n[DIR] gender/                            08-Mar-2015 07:36    -   \n[DIR] gene/                              21-Jul-2017 07:56    -   \n[   ] genealogytree.zip                  08-Dec-2017 13:53  4.7M  \n[DIR] genealogytree/                     08-Dec-2017 13:53    -   \n[   ] genmpage.zip                       16-Sep-2006 16:17   78K  \n[DIR] genmpage/                          16-Sep-2006 16:23    -   \n[   ] gentombow.zip                      16-Mar-2018 17:43  506K  \n[DIR] gentombow/                         16-Mar-2018 17:43    -   \n[   ] geometry-de.zip                    29-Mar-2011 21:09  443K  \n[DIR] geometry-de/                       29-Mar-2011 21:09    -   \n[   ] geometry.zip                       24-Mar-2018 21:48  471K  \n[DIR] geometry/                          24-Mar-2018 21:48    -   \n[   ] germkorr.zip                       28-Jul-2009 11:31  171K  \n[DIR] germkorr/                          03-Aug-2009 00:55    -   \n[   ] getfiledate.zip                    26-Nov-2009 13:24  106K  \n[DIR] getfiledate/                       26-Nov-2009 13:33    -   \n[   ] getitems.zip                       11-Jan-2016 21:25  203K  \n[DIR] getitems/                          11-Jan-2016 21:25    -   \n[   ] getmap.zip                         20-Jun-2016 19:10  2.2M  \n[DIR] getmap/                            20-Jun-2016 19:10    -   \n[   ] ghab.zip                           04-Apr-2013 16:35   28K  \n[DIR] ghab/                              04-Apr-2013 16:43    -   \n[   ] ghsystem.zip                       16-Jul-2016 15:58  2.9M  \n[DIR] ghsystem/                          16-Jul-2016 15:58    -   \n[   ] gincltex.zip                       05-Sep-2011 20:38  169K  \n[DIR] gincltex/                          05-Sep-2011 20:38    -   \n[   ] ginpenc.zip                        29-Dec-2011 22:43  199K  \n[DIR] ginpenc/                           29-Dec-2011 22:43    -   \n[   ] gitinfo.zip                        14-May-2014 22:25   84K  \n[DIR] gitinfo/                           14-May-2014 22:33    -   \n[   ] gitinfo2.zip                       21-Nov-2015 06:16  139K  \n[DIR] gitinfo2/                          21-Nov-2015 06:16    -   \n[   ] gitlog.zip                         22-Nov-2015 09:20  100K  \n[DIR] gitlog/                            22-Nov-2015 09:20    -   \n[   ] gloss-occitan.zip                  06-Feb-2016 15:18   74K  \n[DIR] gloss-occitan/                     06-Feb-2016 15:18    -   \n[   ] gloss.zip                          25-Jun-2005 13:09  111K  \n[DIR] gloss/                             25-Jun-2005 15:15    -   \n[   ] glossaries-danish.zip              25-Nov-2014 06:47  122K  \n[DIR] glossaries-danish/                 25-Nov-2014 06:47    -   \n[   ] glossaries-dutch.zip               28-Nov-2014 13:35  152K  \n[DIR] glossaries-dutch/                  28-Nov-2014 13:35    -   \n[   ] glossaries-english.zip             25-Nov-2014 05:13  121K  \n[DIR] glossaries-english/                25-Nov-2014 05:13    -   \n[   ] glossaries-extra.zip               07-Mar-2018 06:35  5.2M  \n[DIR] glossaries-extra/                  07-Mar-2018 06:35    -   \n[   ] glossaries-finnish.zip             04-Apr-2016 10:42  137K  \n[DIR] glossaries-finnish/                04-Apr-2016 10:42    -   \n[   ] glossaries-french.zip              04-Jan-2017 23:14  191K  \n[DIR] glossaries-french/                 04-Jan-2017 23:14    -   \n[   ] glossaries-german.zip              25-Nov-2014 05:22  122K  \n[DIR] glossaries-german/                 25-Nov-2014 05:22    -   \n[   ] glossaries-irish.zip               25-Nov-2014 05:26  127K  \n[DIR] glossaries-irish/                  25-Nov-2014 05:26    -   \n[   ] glossaries-italian.zip             25-Nov-2014 05:31  122K  \n[DIR] glossaries-italian/                25-Nov-2014 05:31    -   \n[   ] glossaries-magyar.zip              25-Nov-2014 05:34  129K  \n[DIR] glossaries-magyar/                 25-Nov-2014 05:34    -   \n[   ] glossaries-polish.zip              25-Nov-2014 05:38  126K  \n[DIR] glossaries-polish/                 25-Nov-2014 05:38    -   \n[   ] glossaries-portuges.zip            15-Jan-2015 19:26  162K  \n[DIR] glossaries-portuges/               15-Jan-2015 19:26    -   \n[   ] glossaries-serbian.zip             25-Nov-2014 08:07  127K  \n[DIR] glossaries-serbian/                25-Nov-2014 08:07    -   \n[   ] glossaries-spanish.zip             25-Nov-2014 08:36  126K  \n[DIR] glossaries-spanish/                25-Nov-2014 08:36    -   \n[   ] glossaries-swedish.zip             05-Mar-2016 21:19  140K  \n[DIR] glossaries-swedish/                05-Mar-2016 21:19    -   \n[   ] glossaries.zip                     07-Mar-2018 17:49  6.0M  \n[DIR] glossaries/                        07-Mar-2018 17:49    -   \n[   ] gmdoc-enhance.zip                  23-Feb-2009 13:57  141K  \n[DIR] gmdoc-enhance/                     23-Feb-2009 13:57    -   \n[   ] gmdoc.zip                          26-Sep-2012 18:30  1.1M  \n[DIR] gmdoc/                             02-Feb-2011 20:20    -   \n[   ] gmiflink.zip                       13-Aug-2008 14:35   87K  \n[DIR] gmiflink/                          13-Aug-2008 14:53    -   \n[   ] gmp.zip                            10-Mar-2011 23:52  807K  \n[DIR] gmp/                               10-Mar-2011 23:53    -   \n[   ] gmutils.zip                        14-Oct-2011 15:56  1.7M  \n[DIR] gmutils/                           14-Oct-2011 15:56    -   \n[   ] gmverb.zip                         26-Sep-2012 18:32  222K  \n[DIR] gmverb/                            14-Oct-2011 16:18    -   \n[   ] gmverse.zip                        26-Sep-2012 18:34  118K  \n[DIR] gmverse/                           04-Sep-2008 17:27    -   \n[   ] gnuplottex.zip                     21-Aug-2016 22:09  415K  \n[DIR] gnuplottex/                        21-Aug-2016 22:09    -   \n[   ] gotoh.zip                          07-Jul-2017 08:36  291K  \n[DIR] gotoh/                             07-Jul-2017 08:36    -   \n[DIR] gradback/                          03-Apr-2010 15:21    -   \n[   ] gradientframe.zip                  13-Feb-2011 14:59  236K  \n[DIR] gradientframe/                     13-Feb-2011 14:59    -   \n[   ] gradstudentresume.zip              12-Nov-2015 15:40  4.4K  \n[DIR] gradstudentresume/                 12-Nov-2015 15:40    -   \n[   ] grant.zip                          22-Aug-2016 18:19  113K  \n[DIR] grant/                             22-Aug-2016 18:19    -   \n[   ] graphbox.zip                       17-Jan-2018 14:03  275K  \n[DIR] graphbox/                          17-Jan-2018 14:04    -   \n[   ] graphics-cfg.zip                   14-Jun-2016 20:56  2.0K  \n[DIR] graphics-cfg/                      14-Jun-2016 20:56    -   \n[   ] graphics-def.zip                   09-Jan-2018 10:42   22K  \n[DIR] graphics-def/                      09-Jan-2018 10:42    -   \n[   ] graphicx-psmin.zip                 22-Sep-2005 10:16   99K  \n[DIR] graphicx-psmin/                    22-Sep-2005 10:16    -   \n[   ] graphicxbox.zip                    10-Jan-2014 15:22  608K  \n[DIR] graphicxbox/                       10-Jan-2014 15:22    -   \n[   ] graphicxpsd.zip                    29-Jan-2018 18:03  727K  \n[DIR] graphicxpsd/                       29-Jan-2018 18:03    -   \n[   ] graphicxsp.zip                     19-Feb-2016 12:45  683K  \n[DIR] graphicxsp/                        19-Feb-2016 12:45    -   \n[   ] graphviz.zip                       25-Aug-2013 09:13   96K  \n[DIR] graphviz/                          25-Aug-2013 09:13    -   \n[   ] grayhints.zip                      20-Mar-2017 14:32  366K  \n[DIR] grayhints/                         20-Mar-2017 14:32    -   \n[   ] greekdates.zip                     30-Jul-2008 19:06  105K  \n[DIR] greekdates/                        30-Jul-2008 19:13    -   \n[   ] grfpaste.zip                       06-Mar-2010 16:30  371K  \n[DIR] grfpaste/                          06-Mar-2010 14:43    -   \n[   ] grid-system.zip                    16-Feb-2014 20:01   58K  \n[DIR] grid-system/                       16-Feb-2014 20:01    -   \n[   ] grid.zip                           16-Jun-2009 13:24  138K  \n[DIR] grid/                              16-Jun-2009 13:33    -   \n[   ] gridset.zip                        17-Jun-2009 23:31  113K  \n[DIR] gridset/                           17-Jun-2009 23:31    -   \n[   ] gridslides.zip                     28-Nov-2017 17:27  648K  \n[DIR] gridslides/                        28-Nov-2017 17:27    -   \n[   ] grnumalt.zip                       02-Feb-2006 17:39  161K  \n[DIR] grnumalt/                          02-Feb-2006 17:43    -   \n[   ] grundgesetze.zip                   17-Jun-2014 18:34  226K  \n[DIR] grundgesetze/                      17-Jun-2014 18:34    -   \n[   ] gs1.zip                            15-Jul-2017 21:54  1.0M  \n[DIR] gs1/                               15-Jul-2017 21:54    -   \n[   ] gsemthesis.zip                     09-Feb-2015 13:13  298K  \n[DIR] gsemthesis/                        09-Feb-2015 13:13    -   \n[   ] gtrcrd.zip                         25-Dec-2013 08:25  148K  \n[DIR] gtrcrd/                            25-Dec-2013 08:25    -   \n[   ] gtrlib-largetrees.zip              19-Feb-2017 13:56  313K  \n[DIR] gtrlib-largetrees/                 19-Feb-2017 13:56    -   \n[   ] gu.zip                             20-Jan-2007 01:39  721K  \n[DIR] gu/                                20-Jan-2007 02:03    -   \n[   ] guitar.zip                         27-Nov-2013 01:03   98K  \n[DIR] guitar/                            27-Nov-2013 02:03    -   \n[   ] guitarchordschemes.zip             17-Aug-2016 09:46  419K  \n[DIR] guitarchordschemes/                17-Aug-2016 09:46    -   \n[   ] gzt.zip                            16-Feb-2017 13:22  555K  \n[DIR] gzt/                               16-Feb-2017 13:22    -   \n[   ] h2020proposal.zip                  21-Sep-2015 16:40  440K  \n[DIR] h2020proposal/                     21-Sep-2015 16:40    -   \n[   ] ha-prosper.zip                     04-Sep-2005 18:07  293K  \n[DIR] ha-prosper/                        04-Sep-2005 17:13    -   \n[   ] hagenberg-thesis.zip               28-Oct-2017 18:21  5.5M  \n[DIR] hagenberg-thesis/                  28-Oct-2017 18:21    -   \n[   ] halloweenmath.zip                  25-Apr-2017 15:10  907K  \n[DIR] halloweenmath/                     25-Apr-2017 15:10    -   \n[   ] handout.zip                        21-Apr-2017 20:43  208K  \n[DIR] handout/                           21-Apr-2017 20:43    -   \n[   ] hang.zip                           19-Feb-2017 05:39   56K  \n[DIR] hang/                              19-Feb-2017 05:39    -   \n[   ] hanging.zip                        02-Sep-2009 17:47  152K  \n[DIR] hanging/                           02-Sep-2009 17:53    -   \n[   ] har2nat.zip                        03-Apr-2010 23:16  212K  \n[DIR] har2nat/                           03-Apr-2010 23:16    -   \n[   ] hardwrap.zip                       12-Feb-2011 10:23  128K  \n[DIR] hardwrap/                          12-Feb-2011 10:33    -   \n[   ] harmony.zip                        06-May-2007 10:45  139K  \n[DIR] harmony/                           06-May-2007 10:45    -   \n[   ] harnon-cv.zip                      19-May-2012 15:26   52K  \n[DIR] harnon-cv/                         19-May-2012 15:33    -   \n[   ] harpoon.zip                        24-Sep-2008 01:39   20K  \n[DIR] harpoon/                           24-Sep-2008 02:03    -   \n[   ] harvard.zip                        30-Jan-2009 13:32  123K  \n[DIR] harvard/                           30-Jan-2009 13:33    -   \n[   ] hausarbeit-jura.zip                13-Sep-2016 19:50  340K  \n[DIR] hausarbeit-jura/                   13-Sep-2016 19:50    -   \n[   ] havannah.zip                       21-Feb-2015 16:13  223K  \n[DIR] havannah/                          21-Feb-2015 16:13    -   \n[   ] hc.zip                             30-Apr-2005 16:01   76K  \n[DIR] hc/                                16-Aug-2008 14:46    -   \n[   ] he-she.zip                         07-Jun-2016 19:09  210K  \n[DIR] he-she/                            07-Jun-2016 19:09    -   \n[   ] hecthese.zip                       29-Nov-2017 21:46  501K  \n[DIR] hecthese/                          29-Nov-2017 21:46    -   \n[   ] hep.zip                            14-Dec-2005 12:38  3.5K  \n[DIR] hep/                               14-Dec-2005 12:44    -   \n[   ] hepnames.zip                       02-Dec-2014 13:56  1.4M  \n[DIR] hepnames/                          02-Dec-2014 13:56    -   \n[   ] hepparticles.zip                   02-Dec-2014 14:03   87K  \n[DIR] hepparticles/                      02-Dec-2014 14:03    -   \n[   ] hepthesis.zip                      12-Dec-2017 12:43  870K  \n[DIR] hepthesis/                         12-Dec-2017 12:43    -   \n[   ] hepunits.zip                       28-Sep-2007 01:43   77K  \n[DIR] hepunits/                          28-Sep-2007 02:03    -   \n[   ] here.zip                           22-Nov-2009 16:58  866   \n[DIR] here/                              22-Nov-2009 17:03    -   \n[   ] hexgame.zip                        21-Sep-2007 02:54   31K  \n[DIR] hexgame/                           21-Sep-2007 03:03    -   \n[   ] hhtensor.zip                       29-Dec-2011 22:40  355K  \n[DIR] hhtensor/                          29-Dec-2011 22:40    -   \n[   ] hilowres.zip                       30-Apr-2005 16:01  4.5K  \n[DIR] hilowres/                          16-Aug-2008 14:46    -   \n[   ] histogr.zip                        15-Sep-2006 09:32   96K  \n[DIR] histogr/                           15-Sep-2006 08:33    -   \n[   ] hitec.zip                          07-Nov-2008 01:13   22K  \n[DIR] hitec/                             07-Nov-2008 02:03    -   \n[   ] hithesis.zip                       07-Feb-2018 15:10  1.0M  \n[DIR] hithesis/                          07-Feb-2018 15:10    -   \n[   ] hletter.zip                        17-Apr-2013 11:54  2.6M  \n[DIR] hletter/                           17-Apr-2013 11:54    -   \n[   ] horoscop.zip                       16-May-2013 23:02  750K  \n[DIR] horoscop/                          16-May-2013 23:02    -   \n[   ] hpsdiss.zip                        30-Apr-2005 16:01  123K  \n[DIR] hpsdiss/                           01-Feb-2005 20:43    -   \n[   ] hrefhide.zip                       29-Apr-2011 13:10  431K  \n[DIR] hrefhide/                          29-Apr-2011 13:10    -   \n[   ] hulipsum.zip                       03-Mar-2018 19:28  202K  \n[DIR] hulipsum/                          03-Mar-2018 19:28    -   \n[   ] hustthesis.zip                     20-Nov-2016 19:36  911K  \n[DIR] hustthesis/                        20-Nov-2016 19:36    -   \n[   ] hvfloat.zip                        22-Dec-2017 21:26  408K  \n[DIR] hvfloat/                           22-Dec-2017 21:26    -   \n[   ] hvindex.zip                        12-Dec-2017 10:15   76K  \n[DIR] hvindex/                           12-Dec-2017 10:15    -   \n[   ] hypdvips.zip                       22-Jun-2014 21:53  1.3M  \n[DIR] hypdvips/                          22-Jun-2014 21:53    -   \n[   ] hyper.zip                          06-Mar-2010 16:45  314K  \n[DIR] hyper/                             06-Mar-2010 16:53    -   \n[   ] hypernat.zip                       06-Mar-2010 16:49  184K  \n[DIR] hypernat/                          06-Mar-2010 16:53    -   \n[   ] hyperref.zip                       07-Feb-2018 05:35  4.3M  \n[DIR] hyperref/                          07-Feb-2018 05:35    -   \n[   ] hyperxmp.zip                       15-Dec-2017 11:44  665K  \n[DIR] hyperxmp/                          15-Dec-2017 11:44    -   \n[   ] hyphenat.zip                       02-Sep-2009 17:52  161K  \n[DIR] hyphenat/                          02-Sep-2009 17:53    -   \n[   ] idxcmds.zip                        13-Aug-2015 13:02  406K  \n[DIR] idxcmds/                           13-Aug-2015 13:02    -   \n[   ] idxlayout.zip                      01-Apr-2012 20:35  341K  \n[DIR] idxlayout/                         01-Apr-2012 20:35    -   \n[   ] ieeepes.zip                        06-Mar-2010 17:19  256K  \n[DIR] ieeepes/                           06-Mar-2010 17:23    -   \n[   ] ifacmtg.zip                        26-Mar-2006 00:09  392K  \n[DIR] ifacmtg/                           28-May-2009 13:03    -   \n[   ] ifetex.zip                         31-Mar-2018 21:00  144K  \n[DIR] ifetex/                            31-Mar-2018 21:00    -   \n[   ] iffont.zip                         11-Nov-2015 07:13   31K  \n[DIR] iffont/                            11-Nov-2015 07:13    -   \n[   ] ifmslide.zip                       13-Dec-2010 20:00  553K  \n[DIR] ifmslide/                          13-Dec-2010 20:00    -   \n[   ] ifmtarg.zip                        10-Jul-2010 16:37  169K  \n[DIR] ifmtarg/                           10-Jul-2010 16:43    -   \n[   ] ifnextok.zip                       27-Jun-2011 12:37  244K  \n[DIR] ifnextok/                          27-Jun-2011 12:37    -   \n[   ] ifoddpage.zip                      23-Apr-2016 21:20  135K  \n[DIR] ifoddpage/                         23-Apr-2016 21:20    -   \n[   ] ifplatform.zip                     13-Oct-2017 14:58  153K  \n[DIR] ifplatform/                        13-Oct-2017 14:58    -   \n[   ] iftex.zip                          04-Apr-2013 17:51   31K  \n[DIR] iftex/                             04-Apr-2013 17:53    -   \n[   ] ifthenx.zip                        01-Apr-2012 16:49  5.5K  \n[DIR] ifthenx/                           01-Apr-2012 16:53    -   \n[   ] iitem.zip                          02-Apr-2013 20:53  374K  \n[DIR] iitem/                             02-Apr-2013 20:53    -   \n[   ] ijmart.zip                         26-Jun-2013 19:46  944K  \n[DIR] ijmart/                            26-Jun-2013 19:46    -   \n[   ] ijsra.zip                          24-Jul-2017 22:47  693K  \n[DIR] ijsra/                             24-Jul-2017 22:47    -   \n[   ] imac.zip                           06-Mar-2010 17:29  127K  \n[DIR] imac/                              06-Mar-2010 17:33    -   \n[   ] image-gallery.zip                  04-Oct-2007 15:00  1.4M  \n[DIR] image-gallery/                     04-Oct-2007 15:00    -   \n[   ] imakeidx.zip                       15-Oct-2016 23:27  524K  \n[DIR] imakeidx/                          15-Oct-2016 23:27    -   \n[   ] impnattypo.zip                     06-Mar-2015 06:57  164K  \n[DIR] impnattypo/                        06-Mar-2015 06:57    -   \n[   ] import.zip                         06-Mar-2010 17:35  241K  \n[DIR] import/                            06-Mar-2010 17:43    -   \n[   ] imtekda.zip                        01-Apr-2010 21:19  658K  \n[DIR] imtekda/                           01-Apr-2010 21:23    -   \n[   ] incgraph.zip                       12-Mar-2015 20:22  2.0M  \n[DIR] incgraph/                          12-Mar-2015 20:22    -   \n[   ] index.zip                          30-Apr-2005 16:01  185K  \n[DIR] index/                             01-Feb-2005 20:43    -   \n[   ] indextools.zip                     22-Nov-2015 13:03  617K  \n[DIR] indextools/                        22-Nov-2015 13:03    -   \n[   ] indxcite.zip                       11-Oct-2008 18:12   64K  \n[DIR] indxcite/                          11-Oct-2008 17:13    -   \n[   ] inlinedef.zip                      10-Jul-2008 14:09  147K  \n[DIR] inlinedef/                         10-Jul-2008 14:13    -   \n[   ] inputtrc.zip                       11-Oct-2012 15:33  341K  \n[DIR] inputtrc/                          11-Oct-2012 15:33    -   \n[   ] interactiveanimation.zip           06-Jun-2013 17:57  4.2M  \n[DIR] interactiveanimation/              06-Jun-2013 18:03    -   \n[   ] interactiveworkbook.zip            30-Apr-2005 16:01  475K  \n[DIR] interactiveworkbook/               01-Feb-2005 20:43    -   \n[   ] interfaces.zip                     19-Feb-2011 16:28  849K  \n[DIR] interfaces/                        19-Feb-2011 16:33    -   \n[   ] interval.zip                       04-Aug-2014 13:08  307K  \n[DIR] interval/                          04-Aug-2014 13:13    -   \n[   ] intopdf.zip                        16-Mar-2018 20:06  406K  \n[DIR] intopdf/                           16-Mar-2018 20:06    -   \n[   ] inversepath.zip                    06-Aug-2008 02:03   77K  \n[DIR] inversepath/                       06-Aug-2008 02:03    -   \n[   ] invoice.zip                        04-Oct-2011 11:31  142K  \n[DIR] invoice/                           04-Oct-2011 11:31    -   \n[   ] invoice2.zip                       17-Jan-2018 06:27  620K  \n[DIR] invoice2/                          17-Jan-2018 06:27    -   \n[   ] ionumbers.zip                      15-Apr-2014 20:05  486K  \n[DIR] ionumbers/                         15-Apr-2014 20:05    -   \n[   ] iscram.zip                         14-Nov-2017 20:08  268K  \n[DIR] iscram/                            14-Nov-2017 20:08    -   \n[   ] isodate.zip                        05-Jan-2010 10:27  446K  \n[DIR] isodate/                           05-Jan-2010 10:27    -   \n[   ] isodoc.zip                         16-Jan-2016 13:28  2.4M  \n[DIR] isodoc/                            16-Jan-2016 13:28    -   \n[   ] isomath.zip                        12-Sep-2012 17:42  658K  \n[DIR] isomath/                           12-Sep-2012 17:42    -   \n[   ] isonums.zip                        06-Mar-2010 20:42  199K  \n[DIR] isonums/                           06-Mar-2010 20:43    -   \n[   ] isopt.zip                          09-Oct-2017 15:00   61K  \n[DIR] isopt/                             09-Oct-2017 15:00    -   \n[   ] isorot.zip                         30-Apr-2005 16:01  138K  \n[DIR] isorot/                            16-Aug-2008 14:46    -   \n[DIR] isostds/                           03-Apr-2010 22:40    -   \n[   ] isotope.zip                        26-Aug-2011 14:42  3.6K  \n[DIR] isotope/                           26-Aug-2011 14:42    -   \n[   ] issuulinks.zip                     23-Mar-2012 11:59  371K  \n[DIR] issuulinks/                        23-Mar-2012 11:59    -   \n[   ] itnumpar.zip                       04-Apr-2007 02:50  134K  \n[DIR] itnumpar/                          04-Apr-2007 02:53    -   \n[   ] iwhdp.zip                          02-Jun-2015 17:35  428K  \n[DIR] iwhdp/                             02-Jun-2015 17:35    -   \n[   ] jacow.zip                          14-Apr-2016 08:52  1.7M  \n[DIR] jacow/                             14-Apr-2016 08:52    -   \n[   ] jasthesis.zip                      15-Dec-2006 10:58   38K  \n[DIR] jasthesis/                         15-Dec-2006 11:03    -   \n[   ] javadoc.zip                        24-May-2008 22:17  1.1M  \n[DIR] javadoc/                           24-May-2008 22:23    -   \n[   ] jeopardy.zip                       08-Apr-2010 01:30  1.4M  \n[DIR] jeopardy/                          08-Apr-2010 02:03    -   \n[DIR] jhep/                              03-Apr-2010 15:21    -   \n[   ] jj_game.zip                        15-Dec-2016 20:32  1.7M  \n[DIR] jj_game/                           15-Dec-2016 20:32    -   \n[   ] jkmath.zip                         25-Mar-2018 09:52  125K  \n[DIR] jkmath/                            25-Mar-2018 09:52    -   \n[   ] jknappen.zip                       30-Apr-2005 16:01   18K  \n[DIR] jknappen/                          16-Aug-2008 14:46    -   \n[   ] jkthesis.zip                       30-Apr-2005 16:02  176K  \n[DIR] jkthesis/                          01-Feb-2005 20:43    -   \n[   ] jlabels.zip                        17-Dec-2011 11:00   28K  \n[DIR] jlabels/                           17-Dec-2011 11:00    -   \n[   ] jmlr.zip                           01-Aug-2017 19:03  1.9M  \n[DIR] jmlr/                              01-Aug-2017 19:03    -   \n[   ] jpsj.zip                           09-Mar-2007 01:00  159K  \n[DIR] jpsj/                              16-Aug-2008 14:46    -   \n[   ] jsclasses.zip                      11-Mar-2018 11:39  959K  \n[DIR] jsclasses/                         11-Mar-2018 11:39    -   \n[   ] jslectureplanner.zip               12-Mar-2017 11:23  1.3M  \n[DIR] jslectureplanner/                  12-Mar-2017 11:23    -   \n[   ] jumplines.zip                      02-Jun-2015 06:59  252K  \n[DIR] jumplines/                         02-Jun-2015 06:59    -   \n[   ] jura.zip                           25-May-2006 02:00  230K  \n[DIR] jura/                              16-Aug-2008 14:46    -   \n[   ] juraabbrev.zip                     30-Apr-2005 16:02  454K  \n[DIR] juraabbrev/                        01-Feb-2005 20:43    -   \n[   ] jurabib.zip                        08-Jan-2007 14:07  685K  \n[DIR] jurabib/                           08-Jan-2007 14:13    -   \n[   ] juramisc.zip                       26-Nov-2007 12:06  1.5M  \n[DIR] juramisc/                          26-Nov-2007 12:06    -   \n[   ] jurarsp.zip                        06-Mar-2006 15:41  157K  \n[DIR] jurarsp/                           06-Mar-2006 15:43    -   \n[   ] jvlisting.zip                      18-Nov-2011 01:13  198K  \n[DIR] jvlisting/                         18-Nov-2011 02:03    -   \n[DIR] kalender/                          09-Jun-2008 23:53    -   \n[   ] kantlipsum.zip                     20-Nov-2017 16:22  585K  \n[DIR] kantlipsum/                        20-Nov-2017 16:22    -   \n[   ] karnaugh.zip                       07-Feb-2011 09:59  145K  \n[DIR] karnaugh/                          07-Feb-2011 10:03    -   \n[   ] kdgdocs.zip                        02-Nov-2011 21:58  863K  \n[DIR] kdgdocs/                           02-Nov-2011 22:03    -   \n[   ] kerntest.zip                       28-Apr-2005 14:20  668K  \n[DIR] kerntest/                          28-Apr-2005 15:43    -   \n[   ] keycommand.zip                     03-May-2010 01:04  366K  \n[DIR] keycommand/                        03-May-2010 02:03    -   \n[   ] keyfloat.zip                       12-May-2017 13:43  889K  \n[DIR] keyfloat/                          12-May-2017 13:43    -   \n[   ] keyreader.zip                      06-Nov-2012 19:43  237K  \n[DIR] keyreader/                         06-Nov-2012 19:53    -   \n[   ] keystroke.zip                      23-Apr-2010 13:32   43K  \n[DIR] keystroke/                         23-Apr-2010 13:32    -   \n[   ] keyval2e.zip                       26-Aug-2011 08:39  316K  \n[DIR] keyval2e/                          26-Aug-2011 08:43    -   \n[   ] keyvaltable.zip                    22-May-2016 14:21  318K  \n[DIR] keyvaltable/                       22-May-2016 14:21    -   \n[   ] kix.zip                            04-Mar-2011 11:05  122K  \n[DIR] kix/                               04-Mar-2011 11:13    -   \n[   ] knittingpattern.zip                25-Feb-2010 20:25  137K  \n[DIR] knittingpattern/                   25-Feb-2010 20:33    -   \n[   ] knowledge.zip                      18-Feb-2018 12:25  734K  \n[DIR] knowledge/                         18-Feb-2018 12:25    -   \n[   ] koi8.zip                           30-Apr-2005 16:02  3.0K  \n[DIR] koi8/                              01-Feb-2005 20:43    -   \n[   ] koma-moderncvclassic.zip           04-Jan-2012 21:03  190K  \n[DIR] koma-moderncvclassic/              04-Jan-2012 21:03    -   \n[   ] koma-script-SFS.zip                31-May-2005 14:45   40K  \n[DIR] koma-script-SFS/                   31-May-2005 17:13    -   \n[   ] koma-script.zip                    13-Sep-2017 08:00  8.5M  \n[DIR] koma-script/                       13-Sep-2017 08:00    -   \n[   ] komacv-rg.zip                      30-Aug-2017 22:48  1.0M  \n[DIR] komacv-rg/                         30-Aug-2017 22:48    -   \n[   ] komacv.zip                         17-Apr-2017 20:23  1.0M  \n[DIR] komacv/                            17-Apr-2017 20:23    -   \n[   ] ksp-thesis.zip                     10-Dec-2015 13:48  161K  \n[DIR] ksp-thesis/                        10-Dec-2015 13:48    -   \n[   ] ktv-texdata.zip                    30-Apr-2005 16:02  213K  \n[DIR] ktv-texdata/                       01-Feb-2005 20:43    -   \n[   ] ku-template.zip                    28-Nov-2017 10:40  421K  \n[DIR] ku-template/                       28-Nov-2017 10:40    -   \n[   ] l3build.zip                        26-Mar-2018 14:54  715K  \n[DIR] l3build/                           26-Mar-2018 14:54    -   \n[   ] l3experimental.zip                 05-Mar-2018 23:10  3.2M  \n[DIR] l3experimental/                    05-Mar-2018 23:10    -   \n[   ] l3kernel.zip                       05-Mar-2018 22:57  8.1M  \n[DIR] l3kernel/                          05-Mar-2018 22:57    -   \n[   ] l3packages.zip                     21-Feb-2018 22:29  2.0M  \n[DIR] l3packages/                        21-Feb-2018 22:29    -   \n[   ] labbook.zip                        30-Mar-2008 21:34  230K  \n[DIR] labbook/                           30-Mar-2008 20:43    -   \n[   ] labels.zip                         06-Jul-2007 01:55  201K  \n[DIR] labels/                            06-Jul-2007 02:03    -   \n[   ] labelschanged.zip                  11-Dec-2017 10:12  194K  \n[DIR] labelschanged/                     11-Dec-2017 10:12    -   \n[   ] labyrinth.zip                      12-Apr-2014 16:43  225K  \n[DIR] labyrinth/                         12-Apr-2014 16:43    -   \n[   ] lapdf.zip                          02-Sep-2011 07:44  2.7M  \n[DIR] lapdf/                             02-Sep-2011 07:44    -   \n[   ] lastbib.zip                        17-Jul-2012 20:24  1.2K  \n[DIR] lastbib/                           17-Jul-2012 20:33    -   \n[   ] lastpackage.zip                    28-Jun-2014 07:32  250K  \n[DIR] lastpackage/                       28-Jun-2014 07:32    -   \n[   ] lastpage.zip                       30-Mar-2015 14:38  549K  \n[DIR] lastpage/                          30-Mar-2015 14:38    -   \n[DIR] latex-tds/                         11-Nov-2014 23:01    -   \n[   ] latexdemo.zip                      28-Jun-2014 15:06  453K  \n[DIR] latexdemo/                         28-Jun-2014 15:06    -   \n[   ] latexgit.zip                       24-Aug-2016 20:20  433K  \n[DIR] latexgit/                          24-Aug-2016 20:20    -   \n[   ] layaureo.zip                       30-Apr-2005 16:03  135K  \n[DIR] layaureo/                          01-Feb-2005 20:43    -   \n[   ] layouts.zip                        02-Sep-2009 18:07  529K  \n[DIR] layouts/                           02-Sep-2009 18:13    -   \n[   ] lazylist.zip                       30-Dec-2006 10:33  121K  \n[DIR] lazylist/                          30-Dec-2006 10:43    -   \n[   ] lccaps.zip                         24-Jan-2018 18:55  149K  \n[DIR] lccaps/                            24-Jan-2018 18:55    -   \n[   ] lcd.zip                            30-Apr-2005 16:03   73K  \n[DIR] lcd/                               01-Feb-2005 20:43    -   \n[   ] lcg.zip                            19-Aug-2013 14:40  249K  \n[DIR] lcg/                               19-Aug-2013 14:43    -   \n[   ] lcyw.zip                           18-Jul-2008 13:30  114K  \n[DIR] lcyw/                              18-Jul-2008 13:33    -   \n[   ] leading.zip                        15-Dec-2008 13:17   87K  \n[DIR] leading/                           15-Dec-2008 13:23    -   \n[   ] leadsheets.zip                     26-Sep-2017 16:39  964K  \n[DIR] leadsheets/                        26-Sep-2017 16:39    -   \n[   ] leaflet.zip                        17-Mar-2017 11:48  339K  \n[DIR] leaflet/                           17-Mar-2017 11:48    -   \n[   ] ledmac.zip                         06-Aug-2016 16:03  2.6M  \n[DIR] ledmac/                            06-Aug-2016 16:03    -   \n[   ] leftidx.zip                        08-Jan-2007 18:47   55K  \n[DIR] leftidx/                           08-Jan-2007 18:53    -   \n[   ] leipzig.zip                        17-Jun-2017 09:49  602K  \n[DIR] leipzig/                           17-Jun-2017 09:49    -   \n[   ] lengthconvert.zip                  22-Jun-2013 23:38  436K  \n[DIR] lengthconvert/                     22-Jun-2013 23:38    -   \n[   ] lettre.zip                         04-Aug-2017 13:52  1.0M  \n[DIR] lettre/                            04-Aug-2017 13:52    -   \n[   ] lettrine.zip                       01-Sep-2015 14:09  522K  \n[DIR] lettrine/                          01-Sep-2015 14:09    -   \n[   ] levy.zip                           30-Apr-2005 16:03  7.1K  \n[DIR] levy/                              01-Feb-2005 20:43    -   \n[   ] lewis.zip                          23-May-2006 14:43   41K  \n[DIR] lewis/                             23-May-2006 15:13    -   \n[   ] lexikon.zip                        06-Mar-2010 21:06  178K  \n[DIR] lexikon/                           06-Mar-2010 21:13    -   \n[   ] lexitex.zip                        30-Apr-2005 16:03   98K  \n[DIR] lexitex/                           23-Jan-2006 08:44    -   \n[   ] lexref.zip                         11-Jan-2015 13:54  381K  \n[DIR] lexref/                            11-Jan-2015 13:54    -   \n[   ] lgreek.zip                         24-Mar-2011 10:50  202K  \n[DIR] lgreek/                            24-Mar-2011 10:53    -   \n[   ] lhcyr.zip                          30-Apr-2005 16:03   77K  \n[DIR] lhcyr/                             01-Feb-2005 20:43    -   \n[   ] lhelp.zip                          30-Apr-2005 16:03  246K  \n[DIR] lhelp/                             01-Feb-2005 20:43    -   \n[   ] libertine.zip                      22-Oct-2012 15:43  1.4K  \n[DIR] libertine/                         22-Oct-2012 15:53    -   \n[   ] libgreek.zip                       23-Sep-2012 17:22   52K  \n[DIR] libgreek/                          23-Sep-2012 17:22    -   \n[   ] lifia-th.zip                       25-Dec-2007 18:38  237K  \n[DIR] lifia-th/                          25-Dec-2007 18:43    -   \n[   ] limecv.zip                         25-Nov-2017 15:26  616K  \n[DIR] limecv/                            25-Nov-2017 15:26    -   \n[   ] linegoal.zip                       25-Feb-2011 20:01  151K  \n[DIR] linegoal/                          25-Feb-2011 20:03    -   \n[   ] lineno.zip                         16-Feb-2011 15:53  794K  \n[DIR] lineno/                            16-Feb-2011 15:53    -   \n[   ] ling-macros.zip                    13-Oct-2016 17:50  303K  \n[DIR] ling-macros/                       13-Oct-2016 17:50    -   \n[   ] linguex.zip                        28-May-2013 23:09  276K  \n[DIR] linguex/                           28-May-2013 23:13    -   \n[   ] linop.zip                          06-Jun-2016 17:29  223K  \n[DIR] linop/                             06-Jun-2016 17:29    -   \n[   ] lion-msc.zip                       17-Mar-2017 15:05  2.1M  \n[DIR] lion-msc/                          17-Mar-2017 15:05    -   \n[   ] lipsum.zip                         29-Jul-2014 10:26  444K  \n[DIR] lipsum/                            29-Jul-2014 10:26    -   \n[   ] lisp-on-tex.zip                    25-Oct-2015 11:01  396K  \n[DIR] lisp-on-tex/                       25-Oct-2015 11:01    -   \n[   ] listbib.zip                        06-Mar-2010 21:31  360K  \n[DIR] listbib/                           06-Mar-2010 21:33    -   \n[   ] listing.zip                        07-Mar-2010 15:49  254K  \n[DIR] listing/                           07-Mar-2010 15:53    -   \n[   ] listings-ext.zip                   29-Jun-2010 22:02  124K  \n[DIR] listings-ext/                      29-Jun-2010 22:02    -   \n[   ] listings.zip                       04-Jun-2015 23:58  1.4M  \n[DIR] listings/                          04-Jun-2015 23:58    -   \n[   ] listlbls.zip                       04-Aug-2014 17:11   77K  \n[DIR] listlbls/                          04-Aug-2014 17:13    -   \n[   ] listliketab.zip                    30-Apr-2005 16:03  127K  \n[DIR] listliketab/                       01-Feb-2005 20:43    -   \n[   ] listofanswers.zip                  11-Nov-2012 12:31  494K  \n[DIR] listofanswers/                     11-Nov-2012 12:31    -   \n[   ] listofsymbols.zip                  22-Nov-2009 18:07   59K  \n[DIR] listofsymbols/                     22-Nov-2009 18:07    -   \n[   ] liturg.zip                         02-Sep-2008 21:35  121K  \n[DIR] liturg/                            02-Sep-2008 20:13    -   \n[   ] lkproof.zip                        07-Oct-2010 09:12  254K  \n[DIR] lkproof/                           07-Oct-2010 09:13    -   \n[   ] llncsconf.zip                      21-Feb-2018 08:07  124K  \n[DIR] llncsconf/                         21-Feb-2018 08:07    -   \n[   ] lmacs.zip                          31-May-2012 16:31   41K  \n[DIR] lmacs/                             31-May-2012 16:33    -   \n[   ] lmake.zip                          02-Mar-2012 00:25  272K  \n[DIR] lmake/                             02-Mar-2012 02:03    -   \n[   ] lni.zip                            15-Jan-2018 20:23  732K  \n[DIR] lni/                               15-Jan-2018 20:23    -   \n[   ] locality.zip                       12-Nov-2010 14:04  179K  \n[DIR] locality/                          12-Nov-2010 14:13    -   \n[   ] localloc.zip                       11-Jun-2005 13:33  247K  \n[DIR] localloc/                          23-Jan-2006 08:44    -   \n[   ] logbox.zip                         01-Nov-2011 18:29  586K  \n[DIR] logbox/                            01-Nov-2011 18:33    -   \n[   ] logical-markup-utils.zip           10-May-2009 21:27   16K  \n[DIR] logical-markup-utils/              10-May-2009 21:33    -   \n[   ] logicproof.zip                     21-Mar-2014 08:11   61K  \n[DIR] logicproof/                        21-Mar-2014 08:11    -   \n[   ] logpap.zip                         30-Apr-2005 16:03   91K  \n[DIR] logpap/                            01-Feb-2005 20:43    -   \n[   ] logreq.zip                         05-Aug-2010 08:51   12K  \n[DIR] logreq/                            05-Aug-2010 08:53    -   \n[   ] longdivision.zip                   06-Feb-2017 17:12   30K  \n[DIR] longdivision/                      06-Feb-2017 17:12    -   \n[   ] longfbox.zip                       06-Dec-2015 06:44  365K  \n[DIR] longfbox/                          06-Dec-2015 06:44    -   \n[   ] longfigure.zip                     12-Jun-2014 20:40  445K  \n[DIR] longfigure/                        16-Jun-2014 18:34    -   \n[   ] longnamefilelist.zip               01-Oct-2012 09:34  309K  \n[DIR] longnamefilelist/                  01-Oct-2012 09:34    -   \n[   ] loops.zip                          24-May-2013 00:50   21K  \n[DIR] loops/                             24-May-2013 02:03    -   \n[   ] lpic.zip                           23-Dec-2010 20:13  108K  \n[DIR] lpic/                              23-Dec-2010 20:23    -   \n[   ] lplfitch.zip                       30-Jun-2013 11:08  229K  \n[DIR] lplfitch/                          30-Jun-2013 11:13    -   \n[   ] lps.zip                            03-Feb-2011 16:08  177K  \n[DIR] lps/                               03-Feb-2011 16:08    -   \n[   ] lroundrect.zip                     20-Feb-2016 09:23  253K  \n[DIR] lroundrect/                        20-Feb-2016 09:23    -   \n[   ] lsc.zip                            23-Feb-2006 16:03  201K  \n[DIR] lsc/                               23-Feb-2006 16:14    -   \n[   ] lstaddons.zip                      03-May-2012 16:46  392K  \n[DIR] lstaddons/                         03-May-2012 16:53    -   \n[   ] lstbayes.zip                       27-Jun-2016 07:03  274K  \n[DIR] lstbayes/                          27-Jun-2016 07:03    -   \n[   ] lt3graph.zip                       26-Nov-2017 00:38  573K  \n[DIR] lt3graph/                          26-Nov-2017 00:38    -   \n[   ] ltablex.zip                        13-Aug-2014 20:53  228K  \n[DIR] ltablex/                           13-Aug-2014 20:53    -   \n[   ] ltabptch.zip                       21-Mar-2010 21:39  267K  \n[DIR] ltabptch/                          21-Mar-2010 21:43    -   \n[   ] ltxdockit.zip                      28-Mar-2011 16:16  8.7K  \n[DIR] ltxdockit/                         28-Mar-2011 16:23    -   \n[   ] ltxindex.zip                       06-Jun-2008 15:20   84K  \n[DIR] ltxindex/                          06-Jun-2008 15:23    -   \n[   ] ltxkeys.zip                        22-Nov-2012 12:54  794K  \n[DIR] ltxkeys/                           22-Nov-2012 13:03    -   \n[   ] ltxnew.zip                         02-Mar-2011 16:05  170K  \n[DIR] ltxnew/                            02-Mar-2011 16:13    -   \n[   ] ltxtools.zip                       19-Dec-2011 23:27   66K  \n[DIR] ltxtools/                          19-Dec-2011 23:33    -   \n[   ] lucold.zip                         30-Apr-2005 16:03   25K  \n[DIR] lucold/                            01-Feb-2005 20:43    -   \n[   ] lwarp.zip                          01-Apr-2018 14:37  2.2M  \n[DIR] lwarp/                             01-Apr-2018 14:37    -   \n[DIR] lyx/                               11-Sep-2006 18:33    -   \n[   ] macroswap.zip                      21-Aug-2013 23:08  161K  \n[DIR] macroswap/                         21-Aug-2013 23:13    -   \n[   ] mafr.zip                           20-Sep-2006 14:23   63K  \n[DIR] mafr/                              20-Sep-2006 14:33    -   \n[   ] magaz.zip                          29-Nov-2011 10:24  231K  \n[DIR] magaz/                             29-Nov-2011 10:33    -   \n[   ] mailing.zip                        30-Apr-2005 16:03   62K  \n[DIR] mailing/                           01-Feb-2005 20:43    -   \n[   ] mailmerge.zip                      25-Sep-2009 13:29   95K  \n[DIR] mailmerge/                         25-Sep-2009 13:33    -   \n[   ] makebarcode.zip                    29-Jul-2008 21:18  274K  \n[DIR] makebarcode/                       29-Jul-2008 21:23    -   \n[   ] makebase.zip                       10-May-2016 19:04  454K  \n[DIR] makebase/                          10-May-2016 19:04    -   \n[   ] makebox.zip                        30-Apr-2005 16:03  270K  \n[DIR] makebox/                           01-Feb-2005 20:43    -   \n[   ] makecell.zip                       06-Jan-2008 22:18  458K  \n[DIR] makecell/                          03-Apr-2010 22:03    -   \n[   ] makecmds.zip                       03-Sep-2009 08:34  120K  \n[DIR] makecmds/                          03-Sep-2009 08:43    -   \n[DIR] makedtx/                           21-Feb-2018 20:25    -   \n[   ] makeglos.zip                       30-Apr-2005 16:13   11K  \n[DIR] makeglos/                          30-Apr-2005 16:13    -   \n[   ] maker.zip                          16-Jul-2017 08:07  208K  \n[DIR] maker/                             16-Jul-2017 08:07    -   \n[   ] mandi.zip                          27-Mar-2018 05:45  1.3M  \n[DIR] mandi/                             27-Mar-2018 05:45    -   \n[   ] manfnt.zip                         30-Apr-2005 16:03  7.4K  \n[DIR] manfnt/                            01-Feb-2005 20:43    -   \n[   ] manuscript.zip                     21-Jan-2015 17:24   57K  \n[DIR] manuscript/                        21-Jan-2015 17:24    -   \n[   ] mapcodes.zip                       30-Apr-2005 16:03   27K  \n[DIR] mapcodes/                          01-Feb-2005 20:43    -   \n[   ] maple.zip                          30-Apr-2005 16:03   11K  \n[DIR] maple/                             01-Feb-2005 20:43    -   \n[   ] margbib.zip                        03-May-2005 22:08  189K  \n[DIR] margbib/                           23-Jan-2006 08:44    -   \n[   ] marginfit.zip                      10-Jul-2017 20:35  213K  \n[DIR] marginfit/                         10-Jul-2017 20:35    -   \n[   ] marginfix.zip                      08-Sep-2013 19:05  258K  \n[DIR] marginfix/                         08-Sep-2013 19:05    -   \n[   ] marginnote.zip                     22-Apr-2017 12:29  304K  \n[DIR] marginnote/                        22-Apr-2017 12:29    -   \n[   ] matc3.zip                          06-Apr-2013 15:08  433K  \n[DIR] matc3/                             06-Apr-2013 15:08    -   \n[   ] matc3mem.zip                       09-Dec-2014 15:59  387K  \n[DIR] matc3mem/                          09-Dec-2014 15:59    -   \n[   ] mathalfa.zip                       24-Feb-2017 08:41  950K  \n[DIR] mathalfa/                          24-Feb-2017 08:41    -   \n[   ] mathastext.zip                     06-Nov-2016 20:12  573K  \n[DIR] mathastext/                        06-Nov-2016 20:12    -   \n[   ] mathcomp.zip                       19-Jan-2006 16:18  166K  \n[DIR] mathcomp/                          16-Aug-2008 14:46    -   \n[   ] mathexam.zip                       18-Aug-2007 21:41  155K  \n[DIR] mathexam/                          18-Aug-2007 21:43    -   \n[   ] mathfam256.zip                     22-Jan-2018 18:27   87K  \n[DIR] mathfam256/                        22-Jan-2018 18:27    -   \n[   ] mathfixs.zip                       17-Jan-2018 13:37  296K  \n[DIR] mathfixs/                          17-Jan-2018 13:37    -   \n[   ] mathpartir.zip                     25-Feb-2016 04:54  276K  \n[DIR] mathpartir/                        25-Feb-2016 04:54    -   \n[   ] mathpunctspace.zip                 27-Feb-2018 20:44  413K  \n[DIR] mathpunctspace/                    27-Feb-2018 20:44    -   \n[   ] mathtools.zip                      08-Jan-2018 14:58  1.0M  \n[DIR] mathtools/                         08-Jan-2018 14:58    -   \n[   ] matlab-prettifier.zip              19-Jun-2014 15:43  669K  \n[DIR] matlab-prettifier/                 19-Jun-2014 15:53    -   \n[   ] mattens.zip                        30-Mar-2010 00:20  711K  \n[DIR] mattens/                           30-Mar-2010 02:03    -   \n[   ] mattex.zip                         11-Feb-2012 16:57  330K  \n[DIR] mattex/                            11-Feb-2012 17:03    -   \n[   ] maybemath.zip                      05-Aug-2008 15:54   61K  \n[DIR] maybemath/                         05-Aug-2008 15:03    -   \n[   ] mbenotes.zip                       02-Oct-2013 17:41  263K  \n[DIR] mbenotes/                          02-Oct-2013 17:43    -   \n[   ] mcaption.zip                       13-Mar-2009 20:04  126K  \n[DIR] mcaption/                          13-Mar-2009 20:13    -   \n[   ] mceinleger.zip                     30-Apr-2005 16:04   44K  \n[DIR] mceinleger/                        01-Feb-2005 20:43    -   \n[   ] mcexam.zip                         27-Dec-2017 11:01  248K  \n[DIR] mcexam/                            27-Dec-2017 11:01    -   \n[   ] mcite.zip                          02-Oct-2005 19:31  146K  \n[DIR] mcite/                             23-Jan-2006 08:44    -   \n[   ] mciteplus.zip                      13-Sep-2013 13:02  457K  \n[DIR] mciteplus/                         13-Sep-2013 13:02    -   \n[   ] mcmthesis.zip                      01-Feb-2016 08:21  499K  \n[DIR] mcmthesis/                         01-Feb-2016 08:21    -   \n[   ] mdframed.zip                       02-Jul-2013 16:16  1.8M  \n[DIR] mdframed/                          02-Jul-2013 16:23    -   \n[   ] mdwfonts.zip                       13-Dec-2007 13:29  197K  \n[DIR] mdwfonts/                          13-Dec-2007 13:33    -   \n[   ] mdwtools.zip                       23-Jun-2008 17:23  1.8M  \n[DIR] mdwtools/                          16-Aug-2008 14:46    -   \n[   ] media9.zip                         29-Mar-2018 18:07  7.1M  \n[DIR] media9/                            29-Mar-2018 18:07    -   \n[   ] medstarbeamer.zip                  12-Nov-2015 08:37  3.6K  \n[DIR] medstarbeamer/                     12-Nov-2015 08:37    -   \n[   ] meetingmins.zip                    10-Oct-2013 14:14  745K  \n[DIR] meetingmins/                       10-Oct-2013 14:23    -   \n[   ] memexsupp.zip                      20-Mar-2008 17:47  121K  \n[DIR] memexsupp/                         20-Mar-2008 17:53    -   \n[   ] memoir.zip                         16-May-2016 11:02  3.2M  \n[DIR] memoir/                            16-May-2016 11:02    -   \n[   ] memory.zip                         13-May-2013 20:04   32K  \n[DIR] memory/                            13-May-2013 20:04    -   \n[   ] mensa-tex.zip                      05-Dec-2017 22:26  252K  \n[DIR] mensa-tex/                         05-Dec-2017 22:26    -   \n[   ] mentis.zip                         01-Mar-2006 16:36  157K  \n[DIR] mentis/                            01-Mar-2006 16:36    -   \n[   ] menu.zip                           04-Mar-2009 01:02  120K  \n[DIR] menu/                              04-Mar-2009 02:03    -   \n[   ] menukeys.zip                       08-Aug-2016 11:09  566K  \n[DIR] menukeys/                          08-Aug-2016 11:09    -   \n[   ] messagebubbles.zip                 06-Mar-2012 11:33   66K  \n[DIR] messagebubbles/                    06-Mar-2012 11:33    -   \n[   ] metalogo.zip                       29-May-2010 14:20   88K  \n[DIR] metalogo/                          29-May-2010 14:23    -   \n[   ] method.zip                         14-Mar-2010 23:12  338K  \n[DIR] method/                            14-Mar-2010 23:13    -   \n[   ] metre.zip                          30-Apr-2005 16:04  190K  \n[DIR] metre/                             01-Feb-2005 20:43    -   \n[   ] metrix.zip                         21-Mar-2016 18:50  517K  \n[DIR] metrix/                            21-Mar-2016 18:50    -   \n[   ] mff.zip                            21-Jul-2007 13:30  227K  \n[DIR] mff/                               21-Jul-2007 12:33    -   \n[   ] mfirstuc.zip                       14-Nov-2017 13:52  680K  \n[DIR] mfirstuc/                          14-Nov-2017 13:52    -   \n[   ] mflogo.zip                         14-Mar-2010 23:37  358K  \n[DIR] mflogo/                            14-Mar-2010 23:43    -   \n[   ] mfnfss.zip                         10-Dec-2017 22:52  473K  \n[DIR] mfnfss/                            10-Dec-2017 22:52    -   \n[   ] mfpic4ode.zip                      07-Apr-2010 18:47  631K  \n[DIR] mfpic4ode/                         07-Apr-2010 18:53    -   \n[   ] mftinc.zip                         30-Apr-2005 16:04  266K  \n[DIR] mftinc/                            01-Feb-2005 20:43    -   \n[   ] mhchem.zip                         24-Jul-2017 22:53  453K  \n[DIR] mhchem/                            24-Jul-2017 22:53    -   \n[   ] mhequ.zip                          26-Aug-2015 07:16  101K  \n[DIR] mhequ/                             26-Aug-2015 07:16    -   \n[DIR] mhs/                               03-Apr-2010 15:21    -   \n[   ] microtype.zip                      15-Jan-2018 18:28  1.7M  \n[DIR] microtype/                         15-Jan-2018 18:28    -   \n[   ] midpage.zip                        15-Mar-2010 10:42  185K  \n[DIR] midpage/                           15-Mar-2010 10:53    -   \n[   ] miller.zip                         30-Aug-2005 19:11  259K  \n[DIR] miller/                            23-Jan-2006 08:44    -   \n[   ] milog.zip                          03-Jul-2016 16:42  477K  \n[DIR] milog/                             03-Jul-2016 16:42    -   \n[   ] minibox.zip                        21-Jun-2013 10:13  276K  \n[DIR] minibox/                           21-Jun-2013 10:23    -   \n[   ] minidocument.zip                   11-Apr-2017 12:53  186K  \n[DIR] minidocument/                      11-Apr-2017 12:53    -   \n[   ] minipage-marginpar.zip             07-Apr-2008 22:16   88K  \n[DIR] minipage-marginpar/                07-Apr-2008 22:16    -   \n[   ] miniplot.zip                       14-Mar-2010 23:55  174K  \n[DIR] miniplot/                          15-Mar-2010 02:03    -   \n[   ] minitoc.zip                        13-Jul-2015 19:51  614K  \n[DIR] minitoc/                           13-Jul-2015 19:51    -   \n[   ] minorrevision.zip                  15-Nov-2013 20:42  163K  \n[DIR] minorrevision/                     15-Nov-2013 20:42    -   \n[   ] minted.zip                         19-Jul-2017 21:23  831K  \n[DIR] minted/                            19-Jul-2017 21:23    -   \n[   ] minutes.zip                        30-Sep-2016 11:32  406K  \n[DIR] minutes/                           30-Sep-2016 11:32    -   \n[   ] misc.zip                           16-Dec-2012 19:28   29K  \n[DIR] misc/                              16-Dec-2012 19:33    -   \n[   ] mkstmpdad.zip                      14-Dec-2016 18:11  1.0M  \n[DIR] mkstmpdad/                         14-Dec-2016 18:11    -   \n[   ] mla-paper.zip                      30-Dec-2010 15:00  3.7K  \n[DIR] mla-paper/                         30-Dec-2010 15:03    -   \n[   ] mlbib.zip                          22-Aug-2008 16:24  127K  \n[DIR] mlbib/                             22-Aug-2008 15:33    -   \n[   ] mlist.zip                          04-Jul-2009 13:06  200K  \n[DIR] mlist/                             04-Jul-2009 13:13    -   \n[   ] mltex.zip                          30-Apr-2005 16:04   13K  \n[DIR] mltex/                             01-Feb-2005 20:43    -   \n[   ] mmap.zip                           25-Aug-2008 10:56   56K  \n[DIR] mmap/                              25-Aug-2008 10:03    -   \n[   ] mnotes.zip                         05-Nov-2014 14:06  211K  \n[DIR] mnotes/                            05-Nov-2014 14:06    -   \n[   ] mnras.zip                          27-May-2015 16:51  278K  \n[DIR] mnras/                             27-May-2015 16:51    -   \n[   ] moderncv.zip                       29-Jul-2015 10:01  1.7M  \n[DIR] moderncv/                          29-Jul-2015 10:01    -   \n[   ] modernposter.zip                   04-Jan-2018 10:09  374K  \n[DIR] modernposter/                      04-Jan-2018 10:09    -   \n[   ] moderntimeline.zip                 31-Aug-2015 18:31  184K  \n[DIR] moderntimeline/                    31-Aug-2015 18:31    -   \n[   ] modiagram.zip                      23-Sep-2015 13:00  620K  \n[DIR] modiagram/                         23-Sep-2015 13:00    -   \n[   ] modref.zip                         03-Feb-2009 14:31  160K  \n[DIR] modref/                            03-Feb-2009 14:33    -   \n[   ] modroman.zip                       09-Apr-2010 17:08  1.5M  \n[DIR] modroman/                          09-Apr-2010 17:13    -   \n[   ] modular.zip                        01-May-2017 07:39  144K  \n[DIR] modular/                           01-May-2017 07:39    -   \n[   ] monofill.zip                       31-Oct-2012 10:32  293K  \n[DIR] monofill/                          31-Oct-2012 10:32    -   \n[   ] moodle.zip                         12-Jan-2016 09:28  314K  \n[DIR] moodle/                            12-Jan-2016 09:28    -   \n[   ] moreenum.zip                       03-Nov-2011 12:57  217K  \n[DIR] moreenum/                          03-Nov-2011 13:03    -   \n[   ] morefloats.zip                     22-Jul-2015 20:50  496K  \n[DIR] morefloats/                        22-Jul-2015 20:50    -   \n[   ] morehelp.zip                       30-Apr-2005 16:04  8.8K  \n[DIR] morehelp/                          01-Feb-2005 20:43    -   \n[   ] morehype.zip                       10-Nov-2015 17:12  2.5M  \n[DIR] morehype/                          10-Nov-2015 17:12    -   \n[   ] moresize.zip                       20-Mar-2010 18:38  252K  \n[DIR] moresize/                          20-Mar-2010 18:43    -   \n[   ] moreverb.zip                       18-Apr-2011 21:52  121K  \n[DIR] moreverb/                          18-Apr-2011 21:53    -   \n[   ] morewrites.zip                     20-Apr-2017 21:00  1.3M  \n[DIR] morewrites/                        20-Apr-2017 21:00    -   \n[   ] movie15.zip                        17-May-2012 12:54  542K  \n[DIR] movie15/                           17-May-2012 12:54    -   \n[   ] mparhack.zip                       22-Oct-2006 17:44   70K  \n[DIR] mparhack/                          22-Oct-2006 16:53    -   \n[   ] mpdinbrief.zip                     09-Sep-2008 12:07  363K  \n[DIR] mpdinbrief/                        09-Sep-2008 11:13    -   \n[   ] mpgraphics.zip                     04-Apr-2013 12:48  191K  \n[DIR] mpgraphics/                        04-Apr-2013 12:48    -   \n[   ] mpostinl.zip                       01-Mar-2018 06:06  337K  \n[DIR] mpostinl/                          01-Mar-2018 06:06    -   \n[   ] ms.zip                             29-Oct-2011 09:51  2.2M  \n[DIR] ms/                                29-Oct-2011 09:50    -   \n[   ] msc.zip                            02-Jun-2008 14:36  441K  \n[DIR] msc/                               02-Jun-2008 14:43    -   \n[   ] msg.zip                            10-Nov-2006 08:49  1.1M  \n[DIR] msg/                               16-Aug-2008 14:46    -   \n[   ] mslapa.zip                         20-Mar-2010 18:53  281K  \n[DIR] mslapa/                            20-Mar-2010 19:03    -   \n[   ] msu-thesis.zip                     20-Dec-2017 08:02  432K  \n[DIR] msu-thesis/                        20-Dec-2017 08:02    -   \n[   ] mtgreek.zip                        21-Apr-2010 23:22  160K  \n[DIR] mtgreek/                           21-Apr-2010 23:23    -   \n[   ] mucproc.zip                        09-Mar-2017 18:27  335K  \n[DIR] mucproc/                           09-Mar-2017 18:27    -   \n[   ] mugsthesis.zip                     08-Aug-2014 00:02  360K  \n[DIR] mugsthesis/                        08-Aug-2014 02:03    -   \n[   ] multenum.zip                       20-Mar-2011 18:41  108K  \n[DIR] multenum/                          20-Mar-2011 18:43    -   \n[   ] multiaudience.zip                  03-Aug-2015 07:15  693K  \n[DIR] multiaudience/                     03-Aug-2015 07:15    -   \n[   ] multibbl.zip                       30-Apr-2005 16:04   80K  \n[DIR] multibbl/                          01-Feb-2005 20:43    -   \n[   ] multibib.zip                       10-Dec-2008 20:41  219K  \n[DIR] multibib/                          10-Dec-2008 20:41    -   \n[   ] multibibliography.zip              25-Jun-2013 10:21  485K  \n[DIR] multibibliography/                 25-Jun-2013 10:23    -   \n[   ] multibox.zip                       22-Apr-2010 00:07  202K  \n[DIR] multibox/                          22-Apr-2010 02:03    -   \n[   ] multicap.zip                       15-Dec-2006 15:19   99K  \n[DIR] multicap/                          15-Dec-2006 15:23    -   \n[   ] multidef.zip                       20-Apr-2016 06:03  195K  \n[DIR] multidef/                          20-Apr-2016 06:03    -   \n[   ] multienv.zip                       21-May-2012 00:34  207K  \n[DIR] multienv/                          21-May-2012 02:03    -   \n[   ] multilang.zip                      30-Aug-2017 20:57  420K  \n[DIR] multilang/                         30-Aug-2017 20:57    -   \n[   ] multiobjective.zip                 18-Aug-2008 16:20   98K  \n[DIR] multiobjective/                    18-Aug-2008 16:23    -   \n[   ] multirow.zip                       25-Nov-2016 20:35  611K  \n[DIR] multirow/                          25-Nov-2016 20:35    -   \n[   ] musicography.zip                   31-Oct-2017 19:10  262K  \n[DIR] musicography/                      31-Oct-2017 19:10    -   \n[   ] musixguit.zip                      07-Mar-2011 21:29  164K  \n[DIR] musixguit/                         07-Mar-2011 21:29    -   \n[   ] musuos.zip                         17-Dec-2011 18:06  513K  \n[DIR] musuos/                            17-Dec-2011 18:06    -   \n[   ] muthesis.zip                       06-Sep-2011 06:39  9.2K  \n[DIR] muthesis/                          19-Apr-2012 04:45    -   \n[   ] mversion.zip                       26-Mar-2013 22:52  154K  \n[DIR] mversion/                          26-Mar-2013 22:53    -   \n[   ] mwcls.zip                          13-May-2017 22:27  175K  \n[DIR] mwcls/                             13-May-2017 22:27    -   \n[   ] mwe.zip                            30-Mar-2018 18:30  1.5M  \n[DIR] mwe/                               30-Mar-2018 18:30    -   \n[   ] mweights.zip                       30-Mar-2017 19:45  2.0K  \n[DIR] mweights/                          30-Mar-2017 19:45    -   \n[DIR] mwrite/                            03-Apr-2010 15:21    -   \n[   ] mychemistry.zip                    21-Dec-2012 19:54  1.6M  \n[DIR] mychemistry/                       21-Dec-2012 20:03    -   \n[   ] mycv.zip                           21-May-2012 10:53  658K  \n[DIR] mycv/                              21-May-2012 10:53    -   \n[   ] mylatexformat.zip                  13-Feb-2011 01:20  157K  \n[DIR] mylatexformat/                     13-Feb-2011 02:03    -   \n[   ] nag.zip                            03-Dec-2011 11:34  443K  \n[DIR] nag/                               03-Dec-2011 11:43    -   \n[   ] nameauth.zip                       22-Mar-2017 22:48  1.0M  \n[DIR] nameauth/                          22-Mar-2017 22:48    -   \n[   ] namespc.zip                        30-Apr-2005 16:05   88K  \n[DIR] namespc/                           01-Feb-2005 20:43    -   \n[   ] nassflow.zip                       21-Mar-2006 20:08  145K  \n[DIR] nassflow/                          28-May-2009 13:02    -   \n[   ] natbib.zip                         06-Dec-2010 20:08  514K  \n[DIR] natbib/                            06-Dec-2010 20:13    -   \n[   ] natded.zip                         16-Jan-2014 17:37  334K  \n[DIR] natded/                            16-Jan-2014 17:43    -   \n[   ] nath.zip                           30-Apr-2005 16:05  180K  \n[DIR] nath/                              01-Feb-2005 20:43    -   \n[   ] nature.zip                         24-Mar-2011 10:53   13K  \n[DIR] nature/                            24-Mar-2011 11:03    -   \n[   ] navydocs.zip                       06-Jul-2016 08:46  1.1M  \n[DIR] navydocs/                          06-Jul-2016 08:46    -   \n[   ] ncclatex.zip                       20-Jan-2006 01:00  595K  \n[DIR] ncclatex/                          16-Aug-2008 14:46    -   \n[   ] ncctools.zip                       20-Jan-2006 01:00  2.6M  \n[DIR] ncctools/                          16-Aug-2008 14:46    -   \n[   ] nddiss.zip                         23-Aug-2017 18:16  403K  \n[DIR] nddiss/                            23-Aug-2017 18:16    -   \n[   ] ndsu-thesis.zip                    14-Feb-2018 05:47  139K  \n[DIR] ndsu-thesis/                       14-Feb-2018 05:47    -   \n[   ] needspace.zip                      01-Apr-2013 14:33  156K  \n[DIR] needspace/                         01-Apr-2013 14:43    -   \n[   ] nestquot.zip                       30-Apr-2005 16:05  1.7K  \n[DIR] nestquot/                          01-Feb-2005 20:43    -   \n[   ] nevelok.zip                        06-Dec-2015 09:39  209K  \n[DIR] nevelok/                           06-Dec-2015 09:39    -   \n[   ] newalg.zip                         23-May-2005 19:34  217K  \n[DIR] newalg/                            23-Jan-2006 08:44    -   \n[   ] newenviron.zip                     10-Mar-2013 16:16  3.9K  \n[DIR] newenviron/                        10-Mar-2013 16:23    -   \n[   ] newfile.zip                        03-Sep-2009 10:53  156K  \n[DIR] newfile/                           03-Sep-2009 11:03    -   \n[   ] newlfm.zip                         12-Apr-2009 19:30  664K  \n[DIR] newlfm/                            12-Apr-2009 19:30    -   \n[   ] newspaper.zip                      16-Dec-2007 22:52  237K  \n[DIR] newspaper/                         16-Dec-2007 22:53    -   \n[   ] newunicodechar.zip                 13-Nov-2012 17:58  385K  \n[DIR] newunicodechar/                    13-Nov-2012 18:03    -   \n[   ] newvbtm.zip                        17-Sep-2011 10:57   81K  \n[DIR] newvbtm/                           17-Sep-2011 10:57    -   \n[   ] newverbs.zip                       08-May-2012 15:26  182K  \n[DIR] newverbs/                          08-May-2012 15:33    -   \n[   ] nfssext-cfr.zip                    29-Mar-2017 11:56  185K  \n[DIR] nfssext-cfr/                       29-Mar-2017 11:56    -   \n[   ] nicefilelist.zip                   13-Dec-2012 11:09  602K  \n[DIR] nicefilelist/                      13-Dec-2012 11:13    -   \n[   ] niceframe.zip                      17-Jan-2015 10:17  281K  \n[DIR] niceframe/                         17-Jan-2015 10:17    -   \n[   ] nicematrix.zip                     31-Mar-2018 19:06  247K  \n[DIR] nicematrix/                        31-Mar-2018 19:06    -   \n[   ] nicetext.zip                       21-Nov-2015 06:27  2.6M  \n[DIR] nicetext/                          21-Nov-2015 06:27    -   \n[   ] nidanfloat.zip                     09-Mar-2018 17:42  161K  \n[DIR] nidanfloat/                        09-Mar-2018 17:42    -   \n[   ] nih.zip                            29-Sep-2006 16:56   38K  \n[DIR] nih/                               29-Sep-2006 17:03    -   \n[   ] nihbiosketch.zip                   22-Jan-2016 07:34   72K  \n[DIR] nihbiosketch/                      22-Jan-2016 07:34    -   \n[   ] nlctdoc.zip                        14-May-2017 10:09  5.3K  \n[DIR] nlctdoc/                           14-May-2017 10:09    -   \n[   ] nmbib.zip                          27-Jul-2015 22:28  459K  \n[DIR] nmbib/                             27-Jul-2015 22:28    -   \n[   ] noconflict.zip                     27-Apr-2013 00:33  2.3K  \n[DIR] noconflict/                        27-Apr-2013 02:03    -   \n[   ] noindentafter.zip                  30-Nov-2014 22:12  225K  \n[DIR] noindentafter/                     30-Nov-2014 22:12    -   \n[   ] noitcrul.zip                       12-Apr-2006 15:49   81K  \n[DIR] noitcrul/                          12-Apr-2006 16:13    -   \n[   ] nolbreaks.zip                      01-Jun-2012 11:44  124K  \n[DIR] nolbreaks/                         01-Jun-2012 11:53    -   \n[   ] nomencl.zip                        22-Sep-2005 20:52  179K  \n[DIR] nomencl/                           22-Sep-2005 21:13    -   \n[   ] nomentbl.zip                       19-Apr-2006 20:01  180K  \n[DIR] nomentbl/                          19-Apr-2006 20:13    -   \n[   ] nonfloat.zip                       25-May-2005 11:58  310K  \n[DIR] nonfloat/                          25-May-2005 13:13    -   \n[   ] nonumonpart.zip                    15-Apr-2011 12:09  831K  \n[DIR] nonumonpart/                       15-Apr-2011 12:09    -   \n[   ] nopageno.zip                       02-May-2010 22:00  167K  \n[DIR] nopageno/                          02-May-2010 22:03    -   \n[   ] normalcolor.zip                    22-Mar-2016 11:24  156K  \n[DIR] normalcolor/                       22-Mar-2016 11:24    -   \n[   ] nostarch.zip                       10-Jun-2008 14:27  758K  \n[DIR] nostarch/                          10-Jun-2008 14:33    -   \n[   ] notes.zip                          30-Jul-2015 10:55   81K  \n[DIR] notes/                             30-Jul-2015 10:55    -   \n[   ] notes2bib.zip                      11-Jul-2013 12:06  207K  \n[DIR] notes2bib/                         11-Jul-2013 12:13    -   \n[   ] notespages.zip                     21-Aug-2016 23:14  919K  \n[DIR] notespages/                        21-Aug-2016 23:14    -   \n[   ] notestex.zip                       22-Sep-2017 18:22  536K  \n[DIR] notestex/                          22-Sep-2017 18:22    -   \n[   ] notoccite.zip                      02-May-2010 22:15  222K  \n[DIR] notoccite/                         02-May-2010 22:23    -   \n[   ] nowidow.zip                        21-Sep-2011 22:00  173K  \n[DIR] nowidow/                           21-Sep-2011 22:03    -   \n[   ] nox.zip                            13-Jun-2013 07:43  174K  \n[DIR] nox/                               13-Jun-2013 07:43    -   \n[   ] nrc.zip                            04-Feb-2013 16:36  248K  \n[DIR] nrc/                               04-Feb-2013 16:36    -   \n[   ] ntabbing.zip                       02-Jun-2005 07:57   73K  \n[DIR] ntabbing/                          23-Jan-2006 08:44    -   \n[   ] ntgclass.zip                       30-Apr-2005 16:05  1.1M  \n[DIR] ntgclass/                          23-Jan-2006 08:44    -   \n[   ] ntheorem.zip                       06-Sep-2012 12:45  463K  \n[DIR] ntheorem/                          06-Sep-2012 12:45    -   \n[   ] nuc.zip                            29-Apr-2011 07:07   81K  \n[DIR] nuc/                               29-Apr-2011 07:07    -   \n[   ] nucleardata.zip                    19-Oct-2016 19:39  548K  \n[DIR] nucleardata/                       19-Oct-2016 19:39    -   \n[   ] numberedblock.zip                  06-Mar-2014 18:44   74K  \n[DIR] numberedblock/                     06-Mar-2014 18:44    -   \n[   ] numending.zip                      09-May-2015 21:48  166K  \n[DIR] numending/                         09-May-2015 21:48    -   \n[   ] numname.zip                        02-May-2010 22:52  111K  \n[DIR] numname/                           02-May-2010 22:53    -   \n[   ] numnameru.zip                      26-Jul-2017 12:26   69K  \n[DIR] numnameru/                         26-Jul-2017 12:26    -   \n[   ] numprint.zip                       22-Aug-2012 14:07  1.2M  \n[DIR] numprint/                          22-Aug-2012 14:07    -   \n[   ] numspell.zip                       30-Sep-2017 12:49  234K  \n[DIR] numspell/                          30-Sep-2017 12:49    -   \n[   ] nwejm.zip                          14-Feb-2017 21:38  1.8M  \n[DIR] nwejm/                             14-Feb-2017 21:38    -   \n[   ] oberdiek.zip                       30-Mar-2018 17:04   16M  \n[DIR] oberdiek/                          30-Mar-2018 17:04    -   \n[   ] objectz.zip                        02-Jun-2005 09:52  275K  \n[DIR] objectz/                           23-Jan-2006 08:44    -   \n[   ] ocg-p.zip                          11-Jan-2013 11:29  576K  \n[DIR] ocg-p/                             11-Jan-2013 11:29    -   \n[   ] ocgtools.zip                       11-Aug-2013 21:54  4.8M  \n[DIR] ocgtools/                          11-Aug-2013 21:54    -   \n[   ] ocgx.zip                           10-Dec-2012 10:41  1.0M  \n[DIR] ocgx/                              10-Dec-2012 10:41    -   \n[   ] ocgx2.zip                          29-Sep-2017 15:46   15K  \n[DIR] ocgx2/                             29-Sep-2017 15:46    -   \n[   ] ocr-latex.zip                      23-Sep-2006 14:30  173K  \n[DIR] ocr-latex/                         23-Sep-2006 14:33    -   \n[   ] octave.zip                         31-Oct-2017 22:08  252K  \n[DIR] octave/                            31-Oct-2017 22:08    -   \n[   ] octavo.zip                         07-Mar-2007 11:35  119K  \n[DIR] octavo/                            07-Mar-2007 11:43    -   \n[   ] ogonek.zip                         03-Jun-2005 09:57  234K  \n[DIR] ogonek/                            23-Jan-2006 08:44    -   \n[   ] oldstyle.zip                       08-Mar-2009 21:33   55K  \n[DIR] oldstyle/                          08-Mar-2009 21:43    -   \n[   ] onlyamsmath.zip                    10-Jan-2017 23:25  213K  \n[DIR] onlyamsmath/                       10-Jan-2017 23:25    -   \n[   ] onrannual.zip                      26-Sep-2012 18:47  177K  \n[DIR] onrannual/                         14-Mar-2010 20:53    -   \n[   ] opcit.zip                          15-Jun-2007 12:25  278K  \n[DIR] opcit/                             15-Jun-2007 11:33    -   \n[   ] oplotsymbl.zip                     04-Aug-2017 17:51  234K  \n[DIR] oplotsymbl/                        04-Aug-2017 17:51    -   \n[   ] opteng.zip                         30-May-2006 21:04   44K  \n[DIR] opteng/                            30-May-2006 21:13    -   \n[   ] optidef.zip                        29-Nov-2017 19:16  288K  \n[DIR] optidef/                           29-Nov-2017 19:16    -   \n[   ] optional.zip                       02-May-2010 23:58  291K  \n[DIR] optional/                          03-May-2010 02:03    -   \n[   ] options.zip                        06-Dec-2015 06:20  239K  \n[DIR] options/                           06-Dec-2015 06:20    -   \n[   ] ordinalpt.zip                      08-Feb-2007 13:31  258K  \n[DIR] ordinalpt/                         08-Feb-2007 13:33    -   \n[   ] osa.zip                            25-Jul-2005 11:56  544K  \n[DIR] osa/                               01-Feb-2005 20:43    -   \n[   ] ot-tableau.zip                     25-Jul-2017 17:12   81K  \n[DIR] ot-tableau/                        25-Jul-2017 17:12    -   \n[   ] othello.zip                        28-Apr-2005 00:50   24K  \n[DIR] othello/                           16-Aug-2008 14:46    -   \n[   ] othelloboard.zip                   23-Aug-2011 13:09  218K  \n[DIR] othelloboard/                      23-Aug-2011 13:13    -   \n[   ] oubraces.zip                       25-Mar-2011 11:20   61K  \n[DIR] oubraces/                          25-Mar-2011 11:20    -   \n[   ] outline.zip                        19-May-2010 18:19  233K  \n[DIR] outline/                           19-May-2010 18:23    -   \n[   ] outliner.zip                       28-Apr-2005 00:50  3.8K  \n[DIR] outliner/                          01-Feb-2005 20:43    -   \n[   ] outlines.zip                       24-Jan-2012 14:35  129K  \n[DIR] outlines/                          24-Jan-2012 14:35    -   \n[   ] outlining.zip                      25-Oct-2017 11:16  138K  \n[DIR] outlining/                         25-Oct-2017 11:16    -   \n[   ] overlays.zip                       22-Dec-2017 07:33  107K  \n[DIR] overlays/                          22-Dec-2017 07:33    -   \n[   ] overpic.zip                        08-Oct-2017 15:53  344K  \n[DIR] overpic/                           08-Oct-2017 15:53    -   \n[   ] pagecolor.zip                      29-May-2017 13:08  405K  \n[DIR] pagecolor/                         29-May-2017 13:08    -   \n[   ] pagecont.zip                       26-May-2009 22:32   76K  \n[DIR] pagecont/                          26-May-2009 22:43    -   \n[   ] pageno.zip                         29-May-2012 16:41   78K  \n[DIR] pageno/                            29-May-2012 16:43    -   \n[   ] pagenote.zip                       03-Sep-2009 11:22  145K  \n[DIR] pagenote/                          03-Sep-2009 11:23    -   \n[   ] pagerange.zip                      04-Feb-2010 01:47   86K  \n[DIR] pagerange/                         04-Feb-2010 02:03    -   \n[   ] pageslts.zip                       21-Dec-2015 20:10  948K  \n[DIR] pageslts/                          21-Dec-2015 20:10    -   \n[   ] pandora-latex.zip                  23-Sep-2006 14:41  153K  \n[DIR] pandora-latex/                     23-Sep-2006 15:03    -   \n[   ] paper.zip                          01-Jun-2008 17:26  161K  \n[DIR] paper/                             01-Jun-2008 17:33    -   \n[   ] papercdcase.zip                    08-Aug-2006 18:39  141K  \n[DIR] papercdcase/                       08-Aug-2006 18:39    -   \n[   ] papermas.zip                       22-Aug-2011 15:57  417K  \n[DIR] papermas/                          22-Aug-2011 15:57    -   \n[   ] papertex.zip                       30-Jun-2010 22:54  503K  \n[DIR] papertex/                          30-Jun-2010 23:03    -   \n[   ] paracol.zip                        12-Oct-2015 07:42  855K  \n[DIR] paracol/                           12-Oct-2015 07:42    -   \n[   ] parades.zip                        09-Feb-2016 09:57  213K  \n[DIR] parades/                           09-Feb-2016 09:57    -   \n[   ] paralist.zip                       22-Jan-2017 18:27  220K  \n[DIR] paralist/                          22-Jan-2017 18:27    -   \n[   ] parallel.zip                       13-Jan-2007 01:00  128K  \n[DIR] parallel/                          16-Aug-2008 14:46    -   \n[   ] paresse.zip                        16-Feb-2013 13:46  1.6M  \n[DIR] paresse/                           16-Feb-2013 13:53    -   \n[   ] parnotes.zip                       16-Aug-2016 08:33  129K  \n[DIR] parnotes/                          16-Aug-2016 08:33    -   \n[   ] parrun.zip                         30-Apr-2005 16:05  111K  \n[DIR] parrun/                            01-Feb-2005 20:43    -   \n[   ] parselines.zip                     19-Feb-2011 16:36  146K  \n[DIR] parselines/                        19-Feb-2011 16:43    -   \n[   ] parskip.zip                        30-Sep-2010 13:39  172K  \n[DIR] parskip/                           30-Sep-2010 13:43    -   \n[   ] pas-cours.zip                      11-Sep-2016 16:56  709K  \n[DIR] pas-cours/                         11-Sep-2016 16:56    -   \n[   ] pas-crosswords.zip                 03-Dec-2013 15:15  167K  \n[DIR] pas-crosswords/                    03-Dec-2013 15:23    -   \n[   ] pas-cv.zip                         27-Nov-2013 20:42  1.0M  \n[DIR] pas-cv/                            27-Nov-2013 20:43    -   \n[   ] pas-tableur.zip                    01-Feb-2016 13:45  263K  \n[DIR] pas-tableur/                       01-Feb-2016 13:45    -   \n[   ] patchcmd.zip                       03-Jun-2016 08:42  135K  \n[DIR] patchcmd/                          03-Jun-2016 08:42    -   \n[   ] path.zip                           09-Apr-2011 10:19  287K  \n[DIR] path/                              09-Apr-2011 10:23    -   \n[   ] pauldoc.zip                        10-Nov-2009 13:46  144K  \n[DIR] pauldoc/                           10-Nov-2009 13:46    -   \n[   ] pawpict.zip                        30-Apr-2005 16:05   12K  \n[DIR] pawpict/                           01-Feb-2005 20:43    -   \n[DIR] pax/                               23-Apr-2012 14:33    -   \n[   ] pb-diagram.zip                     05-Jun-2005 22:37  164K  \n[DIR] pb-diagram/                        16-Aug-2008 14:46    -   \n[   ] pbox.zip                           08-Dec-2011 01:13  238K  \n[DIR] pbox/                              08-Dec-2011 01:13    -   \n[   ] pbsheet.zip                        30-Apr-2005 16:05  552K  \n[DIR] pbsheet/                           01-Feb-2005 20:43    -   \n[   ] pclnfss.zip                        30-Apr-2005 16:05  578K  \n[DIR] pclnfss/                           01-Feb-2005 20:43    -   \n[   ] pdf14.zip                          26-Mar-2010 22:13  356K  \n[DIR] pdf14/                             26-Mar-2010 22:23    -   \n[   ] pdfcomment.zip                     15-Jun-2016 16:24  1.3M  \n[DIR] pdfcomment/                        15-Jun-2016 16:24    -   \n[   ] pdfcprot.zip                       10-Jun-2005 12:39  396K  \n[DIR] pdfcprot/                          23-Jan-2006 08:44    -   \n[   ] pdfmarginpar.zip                   10-Aug-2011 11:51  455K  \n[DIR] pdfmarginpar/                      10-Aug-2011 11:53    -   \n[   ] pdfpagediff.zip                    24-Jul-2015 15:16  1.1M  \n[DIR] pdfpagediff/                       24-Jul-2015 15:16    -   \n[   ] pdfpages.zip                       31-Oct-2017 16:13  344K  \n[DIR] pdfpages/                          31-Oct-2017 16:13    -   \n[   ] pdfprivacy.zip                     03-Dec-2017 21:49  262K  \n[DIR] pdfprivacy/                        03-Dec-2017 21:49    -   \n[   ] pdfreview.zip                      22-Sep-2017 22:06  511K  \n[DIR] pdfreview/                         22-Sep-2017 22:06    -   \n[   ] pdfscreen.zip                      30-Apr-2005 16:05  742K  \n[DIR] pdfscreen/                         16-Aug-2008 14:46    -   \n[   ] pdfslide.zip                       30-Apr-2005 16:05  221K  \n[DIR] pdfslide/                          16-Aug-2008 14:46    -   \n[   ] pdfsync.zip                        08-Nov-2010 20:55  257K  \n[DIR] pdfsync/                           08-Nov-2010 21:03    -   \n[   ] pdftricks.zip                      24-Nov-2008 12:26  237K  \n[DIR] pdftricks/                         24-Nov-2008 12:33    -   \n[   ] pdfx.zip                           18-May-2017 10:22  5.1M  \n[DIR] pdfx/                              18-May-2017 10:22    -   \n[   ] perfectcut.zip                     03-May-2017 08:18  186K  \n[DIR] perfectcut/                        03-May-2017 08:18    -   \n[   ] perltex.zip                        24-Jul-2010 23:10  305K  \n[DIR] perltex/                           24-Jul-2010 23:13    -   \n[   ] permute.zip                        13-Jan-2007 01:00   82K  \n[DIR] permute/                           16-Aug-2008 14:46    -   \n[   ] petiteannonce.zip                  11-Apr-2012 15:05  266K  \n[DIR] petiteannonce/                     11-Apr-2012 15:13    -   \n[   ] pfarrei.zip                        17-Oct-2013 10:56  500K  \n[DIR] pfarrei/                           17-Oct-2013 11:03    -   \n[   ] pgfkeyx.zip                        21-Apr-2012 23:42  8.3K  \n[DIR] pgfkeyx/                           21-Apr-2012 23:43    -   \n[   ] pgfopts.zip                        11-Jul-2014 18:06  176K  \n[DIR] pgfopts/                           11-Jul-2014 18:13    -   \n[   ] phffullpagefigure.zip              15-Aug-2016 17:52  247K  \n[DIR] phffullpagefigure/                 15-Aug-2016 17:52    -   \n[   ] phfnote.zip                        15-Aug-2016 16:36  659K  \n[DIR] phfnote/                           15-Aug-2016 16:36    -   \n[   ] phfparen.zip                       15-Aug-2016 18:51  307K  \n[DIR] phfparen/                          15-Aug-2016 18:51    -   \n[   ] phfqit.zip                         20-Aug-2017 08:47  403K  \n[DIR] phfqit/                            20-Aug-2017 08:47    -   \n[   ] phfquotetext.zip                   15-Aug-2016 21:42  199K  \n[DIR] phfquotetext/                      15-Aug-2016 21:42    -   \n[   ] phfsvnwatermark.zip                16-Aug-2016 07:40  206K  \n[DIR] phfsvnwatermark/                   16-Aug-2016 07:40    -   \n[   ] phfthm.zip                         16-Aug-2016 08:40  392K  \n[DIR] phfthm/                            16-Aug-2016 08:40    -   \n[   ] philex.zip                         27-Feb-2015 16:05  242K  \n[DIR] philex/                            27-Feb-2015 16:05    -   \n[   ] philosophersimprint.zip            01-Aug-2016 21:54  450K  \n[DIR] philosophersimprint/               01-Aug-2016 21:54    -   \n[   ] phonenumbers.zip                   02-Jan-2018 20:20  3.3M  \n[DIR] phonenumbers/                      02-Jan-2018 20:20    -   \n[   ] phonrule.zip                       21-Apr-2017 12:47   44K  \n[DIR] phonrule/                          21-Apr-2017 12:47    -   \n[   ] photo.zip                          30-Apr-2005 16:06  149K  \n[DIR] photo/                             01-Feb-2005 20:43    -   \n[   ] physics.zip                        20-Dec-2012 17:30  235K  \n[DIR] physics/                           20-Dec-2012 17:33    -   \n[   ] piano.zip                          01-Mar-2011 12:49  2.3K  \n[DIR] piano/                             01-Mar-2011 12:53    -   \n[   ] pict2e.zip                         05-Feb-2016 13:09  806K  \n[DIR] pict2e/                            05-Feb-2016 13:09    -   \n[DIR] pictex2/                           03-Apr-2010 15:21    -   \n[   ] piff.zip                           30-Mar-2011 11:35  714K  \n[DIR] piff/                              30-Mar-2011 11:43    -   \n[   ] pinlabel.zip                       05-Dec-2011 16:50  304K  \n[DIR] pinlabel/                          05-Dec-2011 16:53    -   \n[   ] pittetd.zip                        30-Apr-2005 16:06  360K  \n[DIR] pittetd/                           01-Feb-2005 20:43    -   \n[   ] pitthesis.zip                      30-Apr-2005 16:06   64K  \n[DIR] pitthesis/                         01-Feb-2005 20:43    -   \n[   ] pkgloader.zip                      26-Nov-2017 00:58  477K  \n[DIR] pkgloader/                         26-Nov-2017 00:58    -   \n[   ] pkuthss.zip                        01-Mar-2017 13:44  535K  \n[DIR] pkuthss/                           01-Mar-2017 13:44    -   \n[   ] placeins.zip                       22-Sep-2010 13:58  253K  \n[DIR] placeins/                          22-Sep-2010 14:03    -   \n[   ] plantslabels.zip                   26-Sep-2012 18:53  225K  \n[DIR] plantslabels/                      12-Apr-2010 02:03    -   \n[   ] plari.zip                          21-Jul-2005 15:42  138K  \n[DIR] plari/                             16-Aug-2008 14:46    -   \n[   ] plates.zip                         30-Apr-2005 16:06   93K  \n[DIR] plates/                            01-Feb-2005 20:43    -   \n[   ] play.zip                           10-Jul-2007 01:17  5.5K  \n[DIR] play/                              10-Jul-2007 02:03    -   \n[   ] pm-isomath.zip                     21-Jan-2018 19:25  594K  \n[DIR] pm-isomath/                        21-Jan-2018 19:25    -   \n[DIR] pmat/                              09-Aug-2005 01:10    -   \n[   ] pmgraph.zip                        04-Nov-2008 02:22  141K  \n[DIR] pmgraph/                           04-Nov-2008 02:23    -   \n[   ] poemscol.zip                       24-Jan-2018 05:31  775K  \n[DIR] poemscol/                          24-Jan-2018 05:31    -   \n[   ] poetry.zip                         19-Jun-2017 22:49  274K  \n[DIR] poetry/                            19-Jun-2017 22:49    -   \n[   ] poetrytex.zip                      02-Mar-2016 19:04  298K  \n[DIR] poetrytex/                         02-Mar-2016 19:04    -   \n[   ] pointRuler.zip                     27-Oct-2009 22:41  119K  \n[DIR] pointRuler/                        27-Oct-2009 22:43    -   \n[   ] polexpr.zip                        03-Mar-2018 14:05   62K  \n[DIR] polexpr/                           03-Mar-2018 14:05    -   \n[   ] polski.zip                         05-May-2017 14:45  324K  \n[DIR] polski/                            05-May-2017 14:45    -   \n[   ] polyglossia.zip                    25-Mar-2016 13:42  220K  \n[DIR] polyglossia/                       25-Mar-2016 13:42    -   \n[   ] polynom.zip                        17-Jul-2017 15:14  432K  \n[DIR] polynom/                           17-Jul-2017 15:14    -   \n[   ] polynomial.zip                     18-Mar-2007 19:43  136K  \n[DIR] polynomial/                        19-Mar-2007 15:27    -   \n[   ] polytable.zip                      18-Jul-2013 16:27  301K  \n[DIR] polytable/                         18-Jul-2013 16:33    -   \n[   ] popupmenu.zip                      27-Sep-2010 14:08   79K  \n[DIR] popupmenu/                         27-Sep-2010 14:13    -   \n[   ] postcards.zip                      30-Apr-2005 16:06  2.9K  \n[DIR] postcards/                         01-Feb-2005 20:43    -   \n[   ] powerdot-FUBerlin.zip              25-Jul-2009 10:30  2.1M  \n[DIR] powerdot-FUBerlin/                 25-Jul-2009 10:33    -   \n[   ] powerdot.zip                       28-Aug-2017 22:44  1.0M  \n[DIR] powerdot/                          28-Aug-2017 22:44    -   \n[   ] ppr-prv.zip                        04-Sep-2005 21:32  321K  \n[DIR] ppr-prv/                           04-Sep-2005 21:32    -   \n[   ] pracjourn.zip                      25-Aug-2007 13:50  397K  \n[DIR] pracjourn/                         25-Aug-2007 13:53    -   \n[   ] preprint.zip                       13-May-2013 11:15  794K  \n[DIR] preprint/                          13-May-2013 11:23    -   \n[   ] pressrelease.zip                   10-Sep-2014 20:29  1.0M  \n[DIR] pressrelease/                      10-Sep-2014 20:29    -   \n[   ] prettyref.zip                      05-Nov-2008 15:52   35K  \n[DIR] prettyref/                         05-Nov-2008 15:53    -   \n[   ] preview.zip                        24-Jul-2017 12:34  191K  \n[DIR] preview/                           24-Jul-2017 12:34    -   \n[   ] prftree.zip                        03-Sep-2016 11:58  296K  \n[DIR] prftree/                           03-Sep-2016 11:58    -   \n[   ] printlen.zip                       22-Sep-2010 13:52  240K  \n[DIR] printlen/                          22-Sep-2010 13:53    -   \n[   ] proba.zip                          10-Jun-2008 13:45   76K  \n[DIR] proba/                             10-Jun-2008 12:53    -   \n[   ] probsoln.zip                       10-Jul-2017 15:15  1.1M  \n[DIR] probsoln/                          10-Jul-2017 15:15    -   \n[   ] procIAGssymp.zip                   21-Jul-2005 19:05  5.2K  \n[DIR] procIAGssymp/                      21-Jul-2005 18:13    -   \n[   ] progkeys.zip                       13-Jun-2005 12:16  622K  \n[DIR] progkeys/                          13-Jun-2005 13:43    -   \n[   ] program.zip                        05-May-2017 16:56   64K  \n[DIR] program/                           05-May-2017 16:56    -   \n[   ] progress.zip                       20-May-2006 10:49   87K  \n[DIR] progress/                          20-May-2006 10:13    -   \n[   ] progressbar.zip                    04-May-2014 11:17   89K  \n[DIR] progressbar/                       04-May-2014 11:17    -   \n[   ] proofread.zip                      28-Feb-2017 22:52  323K  \n[DIR] proofread/                         28-Feb-2017 22:52    -   \n[   ] properties.zip                     07-Jul-2009 11:01  2.6K  \n[DIR] properties/                        07-Jul-2009 11:01    -   \n[   ] proposal.zip                       15-Apr-2016 14:28  1.3M  \n[DIR] proposal/                          15-Apr-2016 14:28    -   \n[   ] prosper.zip                        30-Apr-2005 16:06  602K  \n[DIR] prosper/                           01-Feb-2005 20:43    -   \n[   ] protocol.zip                       04-Mar-2012 18:13  323K  \n[DIR] protocol/                          04-Mar-2012 18:23    -   \n[   ] pseudocode.zip                     30-Apr-2005 16:06  135K  \n[DIR] pseudocode/                        01-Feb-2005 20:43    -   \n[   ] psfrag.zip                         15-Jun-2005 17:40  123K  \n[DIR] psfrag/                            27-Aug-2006 11:03    -   \n[   ] psfragx.zip                        07-May-2012 10:50  451K  \n[DIR] psfragx/                           07-May-2012 10:53    -   \n[   ] pslatex.zip                        30-Apr-2005 16:06   18K  \n[DIR] pslatex/                           16-Aug-2008 14:46    -   \n[DIR] psnfss-addons/                     05-Apr-2010 11:13    -   \n[DIR] psnfssx/                           28-Jun-2016 10:53    -   \n[   ] pspicture.zip                      20-Nov-2005 01:00   49K  \n[DIR] pspicture/                         16-Aug-2008 14:47    -   \n[   ] pst-calculate.zip                  04-Feb-2018 20:51   35K  \n[DIR] pst-calculate/                     04-Feb-2018 20:51    -   \n[   ] pst-pdf.zip                        22-Jun-2017 13:21  1.4M  \n[DIR] pst-pdf/                           22-Jun-2017 13:21    -   \n[   ] pst-vowel.zip                      28-Jan-2012 08:43   83K  \n[DIR] pst-vowel/                         28-Jan-2012 08:43    -   \n[   ] pstool.zip                         20-Jan-2018 10:05  370K  \n[DIR] pstool/                            20-Jan-2018 10:05    -   \n[   ] pstring.zip                        03-Jan-2017 19:42  130K  \n[DIR] pstring/                           03-Jan-2017 19:42    -   \n[   ] psu-thesis.zip                     17-Sep-2008 22:10  271K  \n[DIR] psu-thesis/                        17-Sep-2008 22:13    -   \n[   ] ptptex.zip                         21-Nov-2008 13:36  221K  \n[DIR] ptptex/                            21-Nov-2008 13:43    -   \n[   ] punk-latex.zip                     23-Sep-2006 14:38  148K  \n[DIR] punk-latex/                        23-Sep-2006 15:03    -   \n[   ] pxcjkcat.zip                       22-Sep-2012 16:16   17K  \n[DIR] pxcjkcat/                          22-Sep-2012 16:16    -   \n[   ] pxgreeks.zip                       26-Mar-2011 12:45   61K  \n[DIR] pxgreeks/                          26-Mar-2011 12:45    -   \n[   ] pxtatescale.zip                    21-Jan-2017 16:14  2.3K  \n[DIR] pxtatescale/                       21-Jan-2017 16:14    -   \n[   ] pygmentex.zip                      12-Aug-2014 17:32  654K  \n[DIR] pygmentex/                         12-Aug-2014 17:43    -   \n[   ] python.zip                         12-Jun-2012 18:07  2.3K  \n[DIR] python/                            12-Jun-2012 18:13    -   \n[   ] pythonhighlight.zip                09-Feb-2017 14:32  3.4K  \n[DIR] pythonhighlight/                   09-Feb-2017 14:32    -   \n[   ] pythontex.zip                      21-Jul-2017 08:10  1.7M  \n[DIR] pythontex/                         21-Jul-2017 08:10    -   \n[   ] qcm.zip                            01-Mar-2005 01:25  105K  \n[DIR] qcm/                               01-Feb-2005 20:43    -   \n[   ] qobitree.zip                       29-Nov-2008 17:35  6.7K  \n[DIR] qobitree/                          29-Nov-2008 17:35    -   \n[   ] qrcode.zip                         14-Jan-2015 22:21  271K  \n[DIR] qrcode/                            14-Jan-2015 22:21    -   \n[   ] qstest.zip                         24-Feb-2007 14:09  246K  \n[DIR] qstest/                            24-Feb-2007 14:09    -   \n[   ] qsymbols.zip                       25-Jun-2009 23:54  140K  \n[DIR] qsymbols/                          26-Jun-2009 02:03    -   \n[   ] qtree.zip                          24-Jan-2009 14:18  219K  \n[DIR] qtree/                             24-Jan-2009 14:23    -   \n[   ] quicktype.zip                      28-Sep-2016 21:03  177K  \n[DIR] quicktype/                         28-Sep-2016 21:03    -   \n[   ] quotchap.zip                       20-Oct-2012 22:17  293K  \n[DIR] quotchap/                          20-Oct-2012 22:23    -   \n[   ] quoting.zip                        29-Jan-2014 17:40  306K  \n[DIR] quoting/                           29-Jan-2014 17:43    -   \n[   ] quotmark.zip                       19-Dec-2007 18:30  151K  \n[DIR] quotmark/                          19-Dec-2007 18:33    -   \n[   ] r_und_s.zip                        01-Dec-2005 14:28   39K  \n[DIR] r_und_s/                           01-Dec-2005 14:43    -   \n[   ] ran_toks.zip                       18-May-2017 22:30  223K  \n[DIR] ran_toks/                          18-May-2017 22:30    -   \n[   ] randbild.zip                       16-May-2007 07:57   79K  \n[DIR] randbild/                          16-Aug-2008 14:47    -   \n[   ] randomwalk.zip                     29-Nov-2017 21:53  471K  \n[DIR] randomwalk/                        29-Nov-2017 21:53    -   \n[   ] randtext.zip                       02-Oct-2010 16:57  198K  \n[DIR] randtext/                          02-Oct-2010 17:03    -   \n[   ] rangen.zip                         20-Feb-2016 15:57  187K  \n[DIR] rangen/                            20-Feb-2016 15:57    -   \n[   ] rccol.zip                          29-Dec-2007 17:38  151K  \n[DIR] rccol/                             29-Dec-2007 17:38    -   \n[   ] rcs-multi.zip                      03-Apr-2011 11:06  659K  \n[DIR] rcs-multi/                         03-Apr-2011 11:06    -   \n[   ] rcs.zip                            06-Jun-2007 15:33  174K  \n[DIR] rcs/                               16-Aug-2008 14:47    -   \n[   ] rcsinfo.zip                        25-Feb-2005 18:06  165K  \n[DIR] rcsinfo/                           25-Feb-2005 09:38    -   \n[   ] readarray.zip                      07-Nov-2016 22:59  481K  \n[DIR] readarray/                         07-Nov-2016 22:59    -   \n[   ] realboxes.zip                      16-Aug-2011 11:53  181K  \n[DIR] realboxes/                         16-Aug-2011 11:53    -   \n[   ] realscripts.zip                    13-Feb-2016 06:58  106K  \n[DIR] realscripts/                       13-Feb-2016 06:58    -   \n[   ] rec-thy.zip                        14-Feb-2018 23:01  124K  \n[DIR] rec-thy/                           14-Feb-2018 23:01    -   \n[   ] recipe.zip                         28-Oct-2006 18:03   26K  \n[DIR] recipe/                            28-Oct-2006 17:13    -   \n[   ] recipebook.zip                     22-Apr-2015 09:13  1.6M  \n[DIR] recipebook/                        22-Apr-2015 09:13    -   \n[   ] recipecard.zip                     28-Oct-2006 13:47  199K  \n[DIR] recipecard/                        28-Oct-2006 13:53    -   \n[   ] rectopma.zip                       02-Oct-2010 17:02  113K  \n[DIR] rectopma/                          02-Oct-2010 17:03    -   \n[   ] refcheck.zip                       15-Feb-2013 11:31   45K  \n[DIR] refcheck/                          15-Feb-2013 11:33    -   \n[   ] refenums.zip                       07-Oct-2016 20:58  190K  \n[DIR] refenums/                          07-Oct-2016 20:58    -   \n[   ] reflectgraphics.zip                07-Jul-2015 17:41  266K  \n[DIR] reflectgraphics/                   07-Jul-2015 17:41    -   \n[   ] refman.zip                         27-Sep-2012 18:26  688K  \n[DIR] refman/                            16-Aug-2008 14:47    -   \n[   ] refstyle.zip                       03-Nov-2010 15:37  711K  \n[DIR] refstyle/                          03-Nov-2010 15:43    -   \n[   ] regcount.zip                       02-Oct-2010 17:19  195K  \n[DIR] regcount/                          02-Oct-2010 17:23    -   \n[   ] regexpatch.zip                     31-Mar-2018 19:58  466K  \n[DIR] regexpatch/                        31-Mar-2018 19:58    -   \n[   ] register.zip                       18-Jan-2011 23:31  183K  \n[DIR] register/                          18-Jan-2011 23:33    -   \n[   ] regstats.zip                       08-Jan-2012 11:56  400K  \n[DIR] regstats/                          08-Jan-2012 11:56    -   \n[   ] reledmac.zip                       28-Feb-2018 20:42  3.3M  \n[DIR] reledmac/                          28-Feb-2018 20:42    -   \n[   ] relenc.zip                         06-Apr-2011 08:23   76K  \n[DIR] relenc/                            06-Apr-2011 08:33    -   \n[   ] relsize.zip                        26-May-2013 12:53  306K  \n[DIR] relsize/                           26-May-2013 12:53    -   \n[   ] renditions.zip                     06-Feb-2010 13:34   58K  \n[DIR] renditions/                        06-Feb-2010 13:43    -   \n[   ] repeatindex.zip                    30-Apr-2005 16:14  3.0K  \n[DIR] repeatindex/                       30-Apr-2005 16:14    -   \n[   ] repltext.zip                       13-Apr-2014 08:17  291K  \n[DIR] repltext/                          13-Apr-2014 08:17    -   \n[   ] resphilosophica.zip                22-Feb-2018 13:18  537K  \n[DIR] resphilosophica/                   22-Feb-2018 13:18    -   \n[DIR] resume/                            03-Apr-2010 23:06    -   \n[   ] revnum.zip                         14-Dec-2008 14:27   59K  \n[DIR] revnum/                            14-Dec-2008 14:33    -   \n[   ] revquantum.zip                     15-Mar-2017 13:39  255K  \n[DIR] revquantum/                        15-Mar-2017 13:39    -   \n[   ] revtex.zip                         12-Aug-2010 13:08  4.0M  \n[DIR] revtex/                            12-Aug-2010 13:13    -   \n[   ] ribbonproofs.zip                   08-Jul-2013 10:41  338K  \n[DIR] ribbonproofs/                      08-Jul-2013 10:43    -   \n[   ] richtext.zip                       18-Oct-2016 14:23  1.7M  \n[DIR] richtext/                          18-Oct-2016 14:23    -   \n[   ] rjlparshap.zip                     13-Jul-2009 00:00  117K  \n[DIR] rjlparshap/                        13-Jul-2009 00:00    -   \n[   ] rmannot.zip                        13-Oct-2016 13:06  7.0M  \n[DIR] rmannot/                           13-Oct-2016 13:06    -   \n[   ] rmathbr.zip                        10-Apr-2016 23:34  221K  \n[DIR] rmathbr/                           10-Apr-2016 23:34    -   \n[   ] rmpage.zip                         04-Oct-2010 11:08  625K  \n[DIR] rmpage/                            04-Oct-2010 11:23    -   \n[   ] robustcommand.zip                  11-Apr-2006 18:27   61K  \n[DIR] robustcommand/                     11-Apr-2006 18:43    -   \n[   ] robustindex.zip                    02-Oct-2017 15:36  460K  \n[DIR] robustindex/                       02-Oct-2017 15:36    -   \n[   ] romanbar.zip                       02-Jan-2012 13:57  359K  \n[DIR] romanbar/                          02-Jan-2012 13:57    -   \n[   ] romanbarpagenumber.zip             08-Feb-2015 06:14  210K  \n[DIR] romanbarpagenumber/                08-Feb-2015 06:14    -   \n[   ] romanneg.zip                       13-Oct-2010 12:04  179K  \n[DIR] romanneg/                          13-Oct-2010 12:13    -   \n[   ] romannum.zip                       03-Sep-2009 12:55  131K  \n[DIR] romannum/                          03-Sep-2009 13:03    -   \n[   ] rotfloat.zip                       31-Jul-2005 16:50  217K  \n[DIR] rotfloat/                          31-Jul-2005 16:13    -   \n[   ] rotpages.zip                       30-Apr-2005 16:07  174K  \n[DIR] rotpages/                          23-Jan-2006 08:44    -   \n[   ] roundbox.zip                       06-Apr-2013 09:48  1.8K  \n[DIR] roundbox/                          04-Apr-2013 12:21    -   \n[   ] rpg-module.zip                     26-Apr-2016 17:56  8.3M  \n[DIR] rpg-module/                        26-Apr-2016 17:56    -   \n[   ] rrgtrees.zip                       30-Apr-2005 16:07  101K  \n[DIR] rrgtrees/                          01-Feb-2005 20:43    -   \n[   ] rsc.zip                            22-Aug-2016 22:06  197K  \n[DIR] rsc/                               22-Aug-2016 22:06    -   \n[   ] rst.zip                            21-Mar-2006 19:47  164K  \n[DIR] rst/                               28-May-2009 13:05    -   \n[   ] rterface.zip                       21-Apr-2013 12:55   53K  \n[DIR] rterface/                          21-Apr-2013 12:55    -   \n[   ] rtkinenc.zip                       04-Oct-2010 11:18  257K  \n[DIR] rtkinenc/                          13-Oct-2010 14:14    -   \n[   ] rtklage.zip                        06-Feb-2006 17:30   63K  \n[DIR] rtklage/                           16-Aug-2008 14:47    -   \n[   ] rtsched.zip                        29-Sep-2011 15:37   74K  \n[DIR] rtsched/                           29-Sep-2011 15:37    -   \n[   ] rubik.zip                          28-Feb-2018 14:44  3.4M  \n[DIR] rubik/                             28-Feb-2018 14:44    -   \n[   ] russ.zip                           25-Jan-2012 23:56  329K  \n[DIR] russ/                              25-Jan-2012 23:56    -   \n[   ] rutitlepage.zip                    30-May-2017 17:35  159K  \n[DIR] rutitlepage/                       30-May-2017 17:35    -   \n[   ] rviewport.zip                      28-Aug-2011 17:17  243K  \n[DIR] rviewport/                         28-Aug-2011 17:17    -   \n[   ] rvwrite.zip                        27-Aug-2010 14:41   80K  \n[DIR] rvwrite/                           27-Aug-2010 14:43    -   \n[   ] ryethesis.zip                      09-May-2014 11:42  468K  \n[DIR] ryethesis/                         09-May-2014 11:43    -   \n[   ] sae.zip                            30-Apr-2005 16:07   21K  \n[DIR] sae/                               28-Aug-2000 06:14    -   \n[   ] saferef.zip                        10-Apr-2006 14:31  6.4K  \n[DIR] saferef/                           10-Apr-2006 13:43    -   \n[   ] sageep.zip                         15-Jan-2009 01:04  349K  \n[DIR] sageep/                            15-Jan-2009 02:04    -   \n[   ] sagetex.zip                        20-Jun-2009 09:05  488K  \n[DIR] sagetex/                           20-Jun-2009 09:05    -   \n[   ] sanitize-umlaut.zip                28-May-2016 13:16  363K  \n[DIR] sanitize-umlaut/                   28-May-2016 13:16    -   \n[   ] sansmath.zip                       22-Apr-2010 21:13  181K  \n[DIR] sansmath/                          22-Apr-2010 21:23    -   \n[   ] sapthesis.zip                      04-Dec-2015 18:28  263K  \n[DIR] sapthesis/                         04-Dec-2015 18:28    -   \n[   ] sasnrdisplay.zip                   01-Dec-2017 15:27  214K  \n[DIR] sasnrdisplay/                      01-Dec-2017 15:27    -   \n[   ] sauerj.zip                         30-Apr-2005 16:07  716K  \n[DIR] sauerj/                            23-Jan-2006 08:44    -   \n[   ] sauterfonts.zip                    30-Apr-2005 16:07  6.1K  \n[DIR] sauterfonts/                       01-Feb-2005 20:43    -   \n[   ] savefnmark.zip                     22-Jun-2005 19:43  174K  \n[DIR] savefnmark/                        23-Jan-2006 08:44    -   \n[DIR] savesym/                           02-Sep-2013 17:33    -   \n[   ] savetrees.zip                      14-Apr-2016 10:38  507K  \n[DIR] savetrees/                         14-Apr-2016 10:38    -   \n[   ] scale.zip                          30-Apr-2005 16:08   11K  \n[DIR] scale/                             01-Feb-2005 20:43    -   \n[   ] scalebar.zip                       30-Apr-2005 16:08   56K  \n[DIR] scalebar/                          01-Feb-2005 20:43    -   \n[   ] scalerel.zip                       29-Dec-2016 15:59  326K  \n[DIR] scalerel/                          29-Dec-2016 15:59    -   \n[   ] scanpages.zip                      02-Dec-2016 22:25  141K  \n[DIR] scanpages/                         02-Dec-2016 22:25    -   \n[   ] schedule.zip                       14-Jan-2007 15:02  126K  \n[DIR] schedule/                          16-Aug-2008 14:47    -   \n[   ] schule.zip                         07-May-2015 21:55  3.0M  \n[DIR] schule/                            07-May-2015 21:55    -   \n[   ] schwalbe-chess.zip                 08-Jan-2016 10:55  180K  \n[DIR] schwalbe-chess/                    08-Jan-2016 10:55    -   \n[   ] scientific-thesis-cover.zip        30-Dec-2017 20:18   69K  \n[DIR] scientific-thesis-cover/           30-Dec-2017 20:18    -   \n[DIR] scientificpaper/                   03-Apr-2010 15:21    -   \n[   ] sciposter.zip                      18-Aug-2006 16:49  226K  \n[DIR] sciposter/                         18-Aug-2006 16:53    -   \n[   ] sciwordconv.zip                    30-Apr-2005 16:08  3.1K  \n[DIR] sciwordconv/                       01-Feb-2005 20:43    -   \n[   ] sclang-prettifier.zip              01-Sep-2014 14:33  509K  \n[DIR] sclang-prettifier/                 01-Sep-2014 14:33    -   \n[   ] scratch.zip                        30-Dec-2017 17:39  457K  \n[DIR] scratch/                           30-Dec-2017 17:39    -   \n[   ] scratchx.zip                       28-Jul-2017 16:35  448K  \n[DIR] scratchx/                          28-Jul-2017 16:35    -   \n[   ] screenplay-pkg.zip                 06-Aug-2017 08:06  162K  \n[DIR] screenplay-pkg/                    06-Aug-2017 08:06    -   \n[   ] screenplay.zip                     02-Jul-2012 22:27  171K  \n[DIR] screenplay/                        02-Jul-2012 22:33    -   \n[   ] script.zip                         30-Apr-2005 16:08   18K  \n[DIR] script/                            01-Feb-2005 20:43    -   \n[   ] scrjrnl.zip                        24-Sep-2012 22:33  124K  \n[DIR] scrjrnl/                           24-Sep-2012 22:43    -   \n[   ] scrlttr2copy.zip                   14-Feb-2016 10:16   87K  \n[DIR] scrlttr2copy/                      14-Feb-2016 10:16    -   \n[   ] sdrt.zip                           05-Jul-2009 15:30  179K  \n[DIR] sdrt/                              05-Jul-2009 15:33    -   \n[   ] sduthesis.zip                      13-Jun-2016 07:46  3.0M  \n[DIR] sduthesis/                         13-Jun-2016 07:46    -   \n[   ] secdot.zip                         25-Oct-2010 17:05  250K  \n[DIR] secdot/                            25-Oct-2010 17:13    -   \n[   ] section.zip                        21-Oct-2010 10:54  357K  \n[DIR] section/                           21-Oct-2010 11:03    -   \n[   ] sectionbox.zip                     21-Jan-2006 17:32  359K  \n[DIR] sectionbox/                        21-Jan-2006 17:43    -   \n[   ] sectionbreak.zip                   04-Jan-2018 11:44   41K  \n[DIR] sectionbreak/                      04-Jan-2018 11:44    -   \n[   ] sectsty.zip                        27-Jun-2005 13:47  235K  \n[DIR] sectsty/                           23-Jan-2006 08:44    -   \n[   ] seealso.zip                        24-Mar-2017 05:43  257K  \n[DIR] seealso/                           24-Mar-2017 05:43    -   \n[   ] selectp.zip                        24-Oct-2010 13:58  276K  \n[DIR] selectp/                           24-Oct-2010 14:03    -   \n[   ] semantic-markup.zip                28-Oct-2016 20:57  270K  \n[DIR] semantic-markup/                   28-Oct-2016 20:57    -   \n[   ] semantic.zip                       27-Jun-2005 17:04  387K  \n[DIR] semantic/                          23-Jan-2006 08:44    -   \n[   ] seminar.zip                        13-May-2014 16:25  422K  \n[DIR] seminar/                           13-May-2014 16:33    -   \n[   ] semioneside.zip                    21-Sep-2005 17:53  134K  \n[DIR] semioneside/                       21-Sep-2005 18:13    -   \n[   ] semproc.zip                        16-Jun-2015 11:55  360K  \n[DIR] semproc/                           16-Jun-2015 11:55    -   \n[   ] sepfootnotes.zip                   19-Jul-2016 15:57  206K  \n[DIR] sepfootnotes/                      19-Jul-2016 15:57    -   \n[   ] sepnum.zip                         24-Oct-2010 14:23  346K  \n[DIR] sepnum/                            24-Oct-2010 14:33    -   \n[   ] seqsplit.zip                       08-Aug-2006 15:58  115K  \n[DIR] seqsplit/                          08-Aug-2006 16:03    -   \n[   ] serbian-def-cyr.zip                28-Aug-2011 17:23  236K  \n[DIR] serbian-def-cyr/                   28-Aug-2011 17:23    -   \n[   ] serbianpart.zip                    19-Jul-2010 13:59  193K  \n[DIR] serbianpart/                       19-Jul-2010 14:03    -   \n[   ] serial.zip                         30-Apr-2005 16:08  7.9K  \n[DIR] serial/                            01-Feb-2005 20:43    -   \n[   ] sesamanuel.zip                     24-Mar-2015 04:12  938K  \n[DIR] sesamanuel/                        24-Mar-2015 04:12    -   \n[   ] sesstime.zip                       17-Jan-2018 13:53  319K  \n[DIR] sesstime/                          17-Jan-2018 13:53    -   \n[   ] setspace.zip                       19-Dec-2011 18:41  8.4K  \n[DIR] setspace/                          19-Dec-2011 18:43    -   \n[   ] seuthesis.zip                      24-Feb-2014 07:27  3.9M  \n[DIR] seuthesis/                         24-Feb-2014 07:27    -   \n[   ] seuthesix.zip                      20-Mar-2016 07:50  6.0M  \n[DIR] seuthesix/                         20-Mar-2016 07:50    -   \n[   ] sf298.zip                          07-Jul-2016 19:25  431K  \n[DIR] sf298/                             07-Jul-2016 19:25    -   \n[   ] sffms.zip                          30-Apr-2005 16:08  171K  \n[DIR] sffms/                             01-Feb-2005 20:43    -   \n[   ] sfg.zip                            25-Oct-2010 17:08  384K  \n[DIR] sfg/                               25-Oct-2010 17:13    -   \n[   ] sfheaders.zip                      31-Dec-2008 13:59  1.5K  \n[DIR] sfheaders/                         31-Dec-2008 14:03    -   \n[DIR] sfmath/                            28-Aug-2007 09:50    -   \n[   ] sgame.zip                          26-Jun-2013 19:49   77K  \n[DIR] sgame/                             26-Jun-2013 19:49    -   \n[   ] shadbox.zip                        30-Apr-2005 16:08  2.5K  \n[DIR] shadbox/                           01-Feb-2005 20:43    -   \n[   ] shadethm.zip                       04-Nov-2010 00:14  358K  \n[DIR] shadethm/                          04-Nov-2010 02:03    -   \n[   ] shadow.zip                         01-Nov-2010 12:00  219K  \n[DIR] shadow/                            01-Nov-2010 12:03    -   \n[   ] shadowtext.zip                     18-May-2012 19:09  142K  \n[DIR] shadowtext/                        18-May-2012 19:09    -   \n[   ] shapepar.zip                       26-May-2013 12:52  186K  \n[DIR] shapepar/                          26-May-2013 12:52    -   \n[   ] shdoc.zip                          04-Sep-2016 18:25  546K  \n[DIR] shdoc/                             04-Sep-2016 18:25    -   \n[   ] shipunov.zip                       26-Oct-2010 12:52  2.0M  \n[DIR] shipunov/                          26-Oct-2010 12:53    -   \n[   ] shortlst.zip                       15-Jul-2005 13:14  279K  \n[DIR] shortlst/                          23-Jan-2006 08:44    -   \n[   ] shorttoc.zip                       15-Jul-2005 14:08  193K  \n[DIR] shorttoc/                          23-Jan-2006 08:44    -   \n[   ] show2e.zip                         13-Mar-2008 18:42   71K  \n[DIR] show2e/                            13-Mar-2008 18:43    -   \n[   ] showcharinbox.zip                  04-Apr-2013 12:17   74K  \n[DIR] showcharinbox/                     04-Apr-2013 12:23    -   \n[   ] showdim.zip                        23-Jan-2013 12:35  2.1K  \n[DIR] showdim/                           23-Jan-2013 12:43    -   \n[   ] showexpl.zip                       11-Dec-2016 13:52  587K  \n[DIR] showexpl/                          11-Dec-2016 13:52    -   \n[   ] showlabels.zip                     09-Jun-2016 19:34  181K  \n[DIR] showlabels/                        09-Jun-2016 19:34    -   \n[   ] showtags.zip                       05-Nov-2010 08:45  208K  \n[DIR] showtags/                          05-Nov-2010 08:53    -   \n[   ] siam.zip                           03-Jul-2010 04:51  229K  \n[DIR] siam/                              19-Apr-2012 04:45    -   \n[   ] sidecap.zip                        21-Jul-2005 09:50  159K  \n[DIR] sidecap/                           23-Jan-2006 08:44    -   \n[   ] sidenotes.zip                      21-Apr-2016 18:45  296K  \n[DIR] sidenotes/                         21-Apr-2016 18:45    -   \n[   ] sides.zip                          03-Jun-2005 14:01   46K  \n[DIR] sides/                             03-Jun-2005 16:13    -   \n[   ] siggraph.zip                       30-Apr-2005 16:08   14K  \n[DIR] siggraph/                          01-Feb-2005 20:43    -   \n[   ] signchart.zip                      13-Feb-2016 06:24  305K  \n[DIR] signchart/                         13-Feb-2016 06:24    -   \n[   ] silence.zip                        04-Jul-2012 10:24  476K  \n[DIR] silence/                           04-Jul-2012 10:24    -   \n[   ] simplecd.zip                       28-Feb-2013 20:34  925K  \n[DIR] simplecd/                          28-Feb-2013 20:34    -   \n[   ] simplecv.zip                       07-Nov-2014 13:06  290K  \n[DIR] simplecv/                          07-Nov-2014 13:06    -   \n[   ] simpleinvoice.zip                  02-Nov-2017 17:41  342K  \n[DIR] simpleinvoice/                     02-Nov-2017 17:41    -   \n[   ] simpler-wick.zip                   11-Dec-2015 13:38   61K  \n[DIR] simpler-wick/                      11-Dec-2015 13:38    -   \n[   ] simplewick.zip                     26-Nov-2007 00:08   75K  \n[DIR] simplewick/                        26-Nov-2007 00:08    -   \n[   ] sistyle.zip                        16-Jul-2008 15:58  387K  \n[DIR] sistyle/                           16-Jul-2008 16:03    -   \n[   ] sitem.zip                          19-Apr-2011 09:49   73K  \n[DIR] sitem/                             19-Apr-2011 09:49    -   \n[   ] siunitx.zip                        20-Mar-2018 20:38  708K  \n[DIR] siunitx/                           20-Mar-2018 20:38    -   \n[DIR] skak/                              08-Jan-2018 21:22    -   \n[   ] skb.zip                            03-Jun-2011 15:36  1.5M  \n[DIR] skb/                               03-Jun-2011 15:36    -   \n[   ] skdoc.zip                          07-Feb-2017 21:58  323K  \n[DIR] skdoc/                             07-Feb-2017 21:58    -   \n[   ] skeycommand.zip                    20-Nov-2011 11:30  329K  \n[DIR] skeycommand/                       20-Nov-2011 11:33    -   \n[   ] skeyval.zip                        18-May-2013 14:17  491K  \n[DIR] skeyval/                           18-May-2013 14:23    -   \n[   ] skmath.zip                         08-Jan-2017 17:14  219K  \n[DIR] skmath/                            08-Jan-2017 17:14    -   \n[   ] skrapport.zip                      14-Sep-2017 09:35  295K  \n[DIR] skrapport/                         14-Sep-2017 09:35    -   \n[   ] slantsc.zip                        02-Jan-2012 14:12  381K  \n[DIR] slantsc/                           02-Jan-2012 14:12    -   \n[   ] slashbox.zip                       30-Apr-2005 16:08  1.9K  \n[DIR] slashbox/                          03-Nov-2010 12:03    -   \n[   ] slidenotes.zip                     28-Aug-2005 20:24  165K  \n[DIR] slidenotes/                        23-Jan-2006 08:44    -   \n[   ] smallcap.zip                       30-Apr-2005 16:08  1.7K  \n[DIR] smallcap/                          01-Feb-2005 20:43    -   \n[   ] smalltableof.zip                   05-Nov-2010 12:06  173K  \n[DIR] smalltableof/                      05-Nov-2010 12:13    -   \n[   ] smartref.zip                       01-Nov-2010 15:41  315K  \n[DIR] smartref/                          01-Nov-2010 15:43    -   \n[   ] smartunits.zip                     05-Feb-2016 07:31  334K  \n[DIR] smartunits/                        05-Feb-2016 07:31    -   \n[   ] smflatex.zip                       30-Apr-2005 16:08   59K  \n[DIR] smflatex/                          16-Aug-2008 14:47    -   \n[   ] snapshot.zip                       15-Jun-2005 19:21  115K  \n[DIR] snapshot/                          23-Jan-2006 08:44    -   \n[   ] snotez.zip                         09-May-2013 13:27  453K  \n[DIR] snotez/                            09-May-2013 13:27    -   \n[   ] songbook.zip                       27-Sep-2012 17:35  1.5M  \n[DIR] songbook/                          28-Sep-2012 04:45    -   \n[   ] songs.zip                          10-Jun-2017 08:48  1.3M  \n[DIR] songs/                             10-Jun-2017 08:48    -   \n[   ] soton.zip                          13-Oct-2009 14:34  1.8K  \n[DIR] soton/                             13-Oct-2009 14:43    -   \n[   ] soul.zip                           30-Apr-2005 16:08  347K  \n[DIR] soul/                              01-Feb-2005 20:43    -   \n[   ] soup.zip                           17-Jan-2017 22:46  129K  \n[DIR] soup/                              17-Jan-2017 22:46    -   \n[   ] spalign.zip                        06-Oct-2016 21:18  130K  \n[DIR] spalign/                           06-Oct-2016 21:18    -   \n[   ] sphack.zip                         23-Dec-2010 14:30  238K  \n[DIR] sphack/                            23-Dec-2010 14:33    -   \n[   ] sphdthesis.zip                     22-Jun-2014 20:23  564K  \n[DIR] sphdthesis/                        22-Jun-2014 20:23    -   \n[   ] spie.zip                           25-Apr-2007 13:56  263K  \n[DIR] spie/                              16-Aug-2008 14:47    -   \n[   ] splitbib.zip                       22-Dec-2005 18:00  158K  \n[DIR] splitbib/                          22-Dec-2005 18:00    -   \n[   ] splitindex.zip                     18-Feb-2016 18:14  452K  \n[DIR] splitindex/                        18-Feb-2016 18:14    -   \n[   ] spotcolor.zip                      15-Nov-2006 15:07   94K  \n[DIR] spotcolor/                         15-Nov-2006 15:07    -   \n[   ] spreadtab.zip                      01-Jan-2018 20:46  1.2M  \n[DIR] spreadtab/                         01-Jan-2018 20:46    -   \n[DIR] springer/                          31-Jan-2016 09:01    -   \n[   ] sprite.zip                         01-Jan-2006 01:00  2.1K  \n[DIR] sprite/                            16-Aug-2008 14:47    -   \n[   ] spverbatim.zip                     22-Aug-2009 18:08  105K  \n[DIR] spverbatim/                        22-Aug-2009 18:13    -   \n[   ] srbook-mem.zip                     09-Jun-2011 16:48  271K  \n[DIR] srbook-mem/                        09-Jun-2011 16:48    -   \n[   ] srcltx.zip                         07-Dec-2006 01:00  118K  \n[DIR] srcltx/                            16-Aug-2008 14:47    -   \n[   ] sseq.zip                           06-Sep-2013 14:57  225K  \n[DIR] sseq/                              06-Sep-2013 14:57    -   \n[   ] sslides.zip                        01-Dec-2013 06:44   29K  \n[DIR] sslides/                           01-Dec-2013 06:44    -   \n[   ] ssqquote.zip                       30-Apr-2005 16:09  8.8K  \n[DIR] ssqquote/                          01-Feb-2005 20:43    -   \n[   ] stack.zip                          30-Apr-2005 16:09  4.2K  \n[DIR] stack/                             01-Feb-2005 20:43    -   \n[   ] stackengine.zip                    13-Feb-2017 14:00  338K  \n[DIR] stackengine/                       13-Feb-2017 14:00    -   \n[   ] stage.zip                          27-Apr-2017 23:19  152K  \n[DIR] stage/                             27-Apr-2017 23:19    -   \n[   ] standalone.zip                     26-Mar-2018 21:12  307K  \n[DIR] standalone/                        26-Mar-2018 21:12    -   \n[   ] statex.zip                         03-Nov-2010 11:43  176K  \n[DIR] statex/                            03-Nov-2010 11:53    -   \n[   ] statex2.zip                        27-Sep-2012 21:05  177K  \n[DIR] statex2/                           14-Sep-2011 18:02    -   \n[   ] statistik.zip                      05-Nov-2010 12:17   96K  \n[DIR] statistik/                         05-Nov-2010 12:23    -   \n[   ] statmath.zip                       10-Mar-2018 11:29  203K  \n[DIR] statmath/                          10-Mar-2018 11:29    -   \n[   ] statrep.zip                        15-Sep-2015 22:43  1.6M  \n[DIR] statrep/                           15-Sep-2015 22:43    -   \n[   ] stdclsdv.zip                       04-Sep-2009 11:45  132K  \n[DIR] stdclsdv/                          04-Sep-2009 11:45    -   \n[   ] stdpage.zip                        31-Mar-2005 10:56  111K  \n[DIR] stdpage/                           31-Mar-2005 10:56    -   \n[   ] stealcaps.zip                      24-Jan-2018 21:06  2.9M  \n[DIR] stealcaps/                         24-Jan-2018 21:06    -   \n[   ] steinmetz.zip                      15-Jun-2009 19:30  106K  \n[DIR] steinmetz/                         15-Jun-2009 19:33    -   \n[   ] stellenbosch.zip                   01-Apr-2015 17:17  4.5M  \n[DIR] stellenbosch/                      01-Apr-2015 17:17    -   \n[   ] stex.zip                           07-Apr-2016 19:58  7.1M  \n[DIR] stex/                              07-Apr-2016 19:58    -   \n[DIR] stmaryrd/                          08-Apr-2011 18:03    -   \n[   ] storebox.zip                       21-Dec-2011 11:25  195K  \n[DIR] storebox/                          21-Dec-2011 11:25    -   \n[   ] storecmd.zip                       27-Oct-2011 10:25  242K  \n[DIR] storecmd/                          27-Oct-2011 10:33    -   \n[   ] streetex.zip                       31-Dec-2008 20:37  172K  \n[DIR] streetex/                          31-Dec-2008 20:43    -   \n[   ] stringstrings.zip                  02-Feb-2015 22:11  426K  \n[DIR] stringstrings/                     02-Feb-2015 22:11    -   \n[   ] struktex.zip                       07-Mar-2018 21:10  934K  \n[DIR] struktex/                          07-Mar-2018 21:10    -   \n[   ] sttools.zip                        03-Apr-2017 11:24  1.0M  \n[DIR] sttools/                           03-Apr-2017 11:24    -   \n[   ] stubs.zip                          19-Dec-2005 14:31  330K  \n[DIR] stubs/                             16-Aug-2008 14:47    -   \n[   ] studenthandouts.zip                16-Mar-2017 19:54  318K  \n[DIR] studenthandouts/                   16-Mar-2017 19:54    -   \n[   ] subdepth.zip                       03-Sep-2007 13:22   98K  \n[DIR] subdepth/                          03-Sep-2007 13:23    -   \n[   ] subeqn.zip                         30-Apr-2005 16:09   82K  \n[DIR] subeqn/                            01-Feb-2005 20:43    -   \n[   ] subeqnarray.zip                    30-Apr-2005 16:09  115K  \n[DIR] subeqnarray/                       01-Feb-2005 20:43    -   \n[   ] subfig.zip                         08-Jul-2005 14:38  517K  \n[DIR] subfig/                            08-Jul-2005 16:43    -   \n[   ] subfigmat.zip                      03-Nov-2010 11:52  281K  \n[DIR] subfigmat/                         03-Nov-2010 11:53    -   \n[   ] subfiles.zip                       23-May-2012 21:21   57K  \n[DIR] subfiles/                          23-May-2012 21:21    -   \n[   ] subfloat.zip                       17-Jun-2008 14:05   97K  \n[DIR] subfloat/                          17-Jun-2008 13:13    -   \n[   ] substances.zip                     09-May-2016 12:25  571K  \n[DIR] substances/                        09-May-2016 12:25    -   \n[   ] substitutefont.zip                 04-Nov-2013 19:47  1.4M  \n[DIR] substitutefont/                    04-Nov-2013 19:47    -   \n[   ] substr.zip                         20-Oct-2009 21:32   20K  \n[DIR] substr/                            20-Oct-2009 21:33    -   \n[   ] subsupscripts.zip                  27-Oct-2009 20:51  101K  \n[DIR] subsupscripts/                     27-Oct-2009 20:53    -   \n[   ] sudoku.zip                         25-Mar-2006 20:19   59K  \n[DIR] sudoku/                            25-Mar-2006 20:43    -   \n[   ] sudokubundle.zip                   20-Feb-2006 01:00  305K  \n[DIR] sudokubundle/                      16-Aug-2008 14:48    -   \n[   ] suftesi.zip                        04-Apr-2016 15:45  1.7M  \n[DIR] suftesi/                           04-Apr-2016 15:45    -   \n[   ] supertabular.zip                   30-Apr-2005 16:09  154K  \n[DIR] supertabular/                      12-Mar-2005 00:00    -   \n[   ] susy.zip                           25-Oct-2006 19:09   54K  \n[DIR] susy/                              25-Oct-2006 19:13    -   \n[   ] svgcolor.zip                       23-Dec-2006 01:00  4.7K  \n[DIR] svgcolor/                          16-Aug-2008 14:48    -   \n[   ] svn-multi.zip                      06-May-2012 14:49  436K  \n[DIR] svn-multi/                         06-May-2012 14:53    -   \n[   ] svn-prov.zip                       24-Apr-2010 22:26  252K  \n[DIR] svn-prov/                          24-Apr-2010 22:33    -   \n[   ] svn.zip                            26-Sep-2007 01:43  438K  \n[DIR] svn/                               26-Sep-2007 02:03    -   \n[   ] svninfo.zip                        23-Mar-2010 21:29  267K  \n[DIR] svninfo/                           23-Mar-2010 21:33    -   \n[   ] swimgraf.zip                       20-Feb-2012 12:20  132K  \n[DIR] swimgraf/                          20-Feb-2012 12:23    -   \n[   ] syllogism.zip                      29-Oct-2008 14:31  334K  \n[DIR] syllogism/                         29-Oct-2008 14:33    -   \n[   ] symbolindex.zip                    30-Aug-2005 13:42  4.1K  \n[DIR] symbolindex/                       30-Aug-2005 13:42    -   \n[   ] sympytexpackage.zip                20-May-2014 23:12  699K  \n[DIR] sympytexpackage/                   20-May-2014 23:13    -   \n[   ] synproof.zip                       05-Jul-2009 15:38   63K  \n[DIR] synproof/                          05-Jul-2009 15:43    -   \n[   ] syntax.zip                         13-Jul-2005 11:52   86K  \n[DIR] syntax/                            23-Jan-2006 08:44    -   \n[   ] syntrace.zip                       13-Mar-2007 15:16   52K  \n[DIR] syntrace/                          13-Mar-2007 15:23    -   \n[   ] synttree.zip                       30-Nov-2009 09:19  143K  \n[DIR] synttree/                          30-Nov-2009 09:19    -   \n[   ] t-angles.zip                       14-Aug-2006 14:44  122K  \n[DIR] t-angles/                          14-Aug-2006 14:53    -   \n[   ] t2.zip                             30-Apr-2005 16:09  148K  \n[DIR] t2/                                23-Jan-2006 08:44    -   \n[   ] tabfigures.zip                     25-Jan-2012 23:39  246K  \n[DIR] tabfigures/                        25-Jan-2012 23:39    -   \n[   ] tableaux.zip                       28-Sep-2008 13:24   63K  \n[DIR] tableaux/                          28-Sep-2008 12:33    -   \n[   ] tablefootnote.zip                  27-Jan-2014 08:41  504K  \n[DIR] tablefootnote/                     27-Jan-2014 08:43    -   \n[   ] tableof.zip                        11-Mar-2015 06:04   65K  \n[DIR] tableof/                           11-Mar-2015 06:04    -   \n[   ] tablestyles.zip                    28-Jun-2014 21:37  450K  \n[DIR] tablestyles/                       28-Jun-2014 21:43    -   \n[   ] tablists.zip                       04-Aug-2009 22:15  225K  \n[DIR] tablists/                          04-Aug-2009 22:23    -   \n[   ] tablor.zip                         07-Oct-2013 18:37  527K  \n[DIR] tablor/                            07-Oct-2013 18:43    -   \n[   ] tabls.zip                          26-Feb-2010 22:28  225K  \n[DIR] tabls/                             26-Feb-2010 22:33    -   \n[   ] tabriz-thesis.zip                  17-Mar-2013 16:29  266K  \n[DIR] tabriz-thesis/                     17-Mar-2013 16:33    -   \n[   ] tabstackengine.zip                 05-Mar-2018 20:10  573K  \n[DIR] tabstackengine/                    05-Mar-2018 20:10    -   \n[   ] tabto.zip                          25-May-2013 16:30  119K  \n[DIR] tabto/                             25-May-2013 16:30    -   \n[   ] tabu.zip                           26-Feb-2011 22:34  1.5M  \n[DIR] tabu/                              26-Feb-2011 22:43    -   \n[   ] tabularborder.zip                  15-Apr-2010 17:15  103K  \n[DIR] tabularborder/                     15-Apr-2010 17:15    -   \n[   ] tabularcalc.zip                    21-Apr-2009 22:17  815K  \n[DIR] tabularcalc/                       21-Apr-2009 22:24    -   \n[   ] tabularew.zip                      01-Jun-2009 14:51  147K  \n[DIR] tabularew/                         01-Jun-2009 14:53    -   \n[   ] tabulary.zip                       22-Jun-2014 00:25  256K  \n[DIR] tabulary/                          22-Jun-2014 02:03    -   \n[   ] tabvar.zip                         22-Jan-2013 17:36  592K  \n[DIR] tabvar/                            22-Jan-2013 17:36    -   \n[   ] tagging.zip                        29-Aug-2011 00:26   85K  \n[DIR] tagging/                           29-Aug-2011 02:03    -   \n[   ] tagpair.zip                        23-Sep-2016 21:00   70K  \n[DIR] tagpair/                           23-Sep-2016 21:00    -   \n[   ] talk.zip                           04-Aug-2007 13:44  135K  \n[DIR] talk/                              04-Aug-2007 13:53    -   \n[   ] tamefloats.zip                     28-Apr-2005 17:15  6.9K  \n[DIR] tamefloats/                        28-Apr-2005 17:15    -   \n[   ] tasks.zip                          13-Aug-2016 22:19  461K  \n[DIR] tasks/                             13-Aug-2016 22:19    -   \n[   ] taupin.zip                         19-Jul-2012 17:59   31K  \n[DIR] taupin/                            01-Feb-2005 20:43    -   \n[DIR] tcldoc/                            04-Jul-2005 12:47    -   \n[   ] tclldoc.zip                        26-Jul-2005 10:23  513K  \n[DIR] tclldoc/                           04-Jul-2005 12:47    -   \n[   ] tcolorbox.zip                      22-Mar-2018 20:53  5.4M  \n[DIR] tcolorbox/                         22-Mar-2018 20:53    -   \n[   ] tdclock.zip                        24-Feb-2014 19:14  244K  \n[DIR] tdclock/                           24-Feb-2014 19:14    -   \n[   ] tdsfrmath.zip                      22-Jun-2009 16:19  745K  \n[DIR] tdsfrmath/                         22-Jun-2009 16:23    -   \n[   ] technica.zip                       20-Nov-2006 22:48  2.1M  \n[DIR] technica/                          20-Nov-2006 22:53    -   \n[   ] technics.zip                       16-Jan-2007 01:00   84K  \n[DIR] technics/                          16-Aug-2008 14:48    -   \n[   ] ted.zip                            07-Mar-2008 22:31  187K  \n[DIR] ted/                               07-Mar-2008 22:33    -   \n[   ] templatetools.zip                  28-Jun-2014 21:39  435K  \n[DIR] templatetools/                     28-Jun-2014 21:43    -   \n[   ] tengwarscript.zip                  13-Jul-2014 00:07  538K  \n[DIR] tengwarscript/                     13-Jul-2014 02:03    -   \n[   ] tensor.zip                         30-Apr-2005 16:09   99K  \n[DIR] tensor/                            01-Feb-2005 20:43    -   \n[   ] termcal-de.zip                     24-Mar-2018 00:15  116K  \n[DIR] termcal-de/                        24-Mar-2018 00:15    -   \n[   ] termcal.zip                        17-May-2011 01:51   84K  \n[DIR] termcal/                           17-May-2011 02:03    -   \n[   ] termlist.zip                       12-Jun-2010 13:26  161K  \n[DIR] termlist/                          12-Jun-2010 13:33    -   \n[   ] testhyphens.zip                    23-Nov-2015 10:51  381K  \n[DIR] testhyphens/                       23-Nov-2015 10:51    -   \n[   ] testidx.zip                        11-Aug-2017 14:22  5.0M  \n[DIR] testidx/                           11-Aug-2017 14:22    -   \n[   ] teubner.zip                        31-Mar-2016 19:18  1.0M  \n[DIR] teubner/                           31-Mar-2016 19:18    -   \n[   ] tex-label.zip                      08-Dec-2009 14:10   38K  \n[DIR] tex-label/                         08-Dec-2009 14:13    -   \n[DIR] texlogos/                          11-Jan-2006 01:31    -   \n[   ] texmate.zip                        21-Sep-2006 18:56  241K  \n[DIR] texmate/                           21-Sep-2006 19:03    -   \n[   ] texments.zip                       27-Dec-2008 22:41   91K  \n[DIR] texments/                          27-Dec-2008 22:41    -   \n[   ] texpower.zip                       30-Apr-2005 16:14  408K  \n[DIR] texpower/                          21-Mar-2006 04:14    -   \n[   ] texshade.zip                       06-Feb-2018 20:16  845K  \n[DIR] texshade/                          06-Feb-2018 20:16    -   \n[   ] textcase.zip                       29-Sep-2005 14:36  159K  \n[DIR] textcase/                          29-Sep-2005 13:44    -   \n[   ] textfit.zip                        28-Nov-2010 20:15  162K  \n[DIR] textfit/                           28-Nov-2010 20:23    -   \n[   ] textglos.zip                       27-May-2013 23:19  417K  \n[DIR] textglos/                          27-May-2013 23:19    -   \n[   ] textgreek.zip                      13-Oct-2011 09:47  464K  \n[DIR] textgreek/                         13-Oct-2011 09:47    -   \n[   ] textmerg.zip                       03-Dec-2010 20:29  255K  \n[DIR] textmerg/                          03-Dec-2010 20:33    -   \n[   ] textopo.zip                        01-Sep-2011 15:01  647K  \n[DIR] textopo/                           01-Sep-2011 15:01    -   \n[   ] textpos.zip                        08-Jun-2016 08:28  325K  \n[DIR] textpos/                           08-Jun-2016 08:28    -   \n[   ] textualicomma.zip                  03-Dec-2017 21:13   55K  \n[DIR] textualicomma/                     03-Dec-2017 21:13    -   \n[   ] texvc.zip                          05-Mar-2018 12:25  249K  \n[DIR] texvc/                             05-Mar-2018 12:25    -   \n[   ] thaienum.zip                       01-May-2017 15:34  184K  \n[DIR] thaienum/                          01-May-2017 15:34    -   \n[   ] thalie.zip                         24-Apr-2017 23:27  415K  \n[DIR] thalie/                            24-Apr-2017 23:27    -   \n[   ] theatre.zip                        20-Sep-2017 20:06  126K  \n[DIR] theatre/                           20-Sep-2017 20:06    -   \n[   ] theoremref.zip                     22-May-2013 20:04  332K  \n[DIR] theoremref/                        22-May-2013 20:13    -   \n[   ] thesis-ekf.zip                     03-Feb-2018 17:38  1.1M  \n[DIR] thesis-ekf/                        03-Feb-2018 17:38    -   \n[   ] thesis-gwu.zip                     02-Feb-2018 18:04  589K  \n[DIR] thesis-gwu/                        02-Feb-2018 18:04    -   \n[   ] thesis-titlepage-fhAC.zip          07-Apr-2006 08:34  145K  \n[DIR] thesis-titlepage-fhAC/             16-Aug-2008 14:48    -   \n[   ] thesis.zip                         12-Feb-2008 11:38  186K  \n[DIR] thesis/                            12-Feb-2008 11:43    -   \n[   ] thinsp.zip                         10-Feb-2016 22:08  291K  \n[DIR] thinsp/                            10-Feb-2016 22:08    -   \n[   ] thmbox.zip                         25-Apr-2005 20:28  101K  \n[DIR] thmbox/                            25-Apr-2005 21:43    -   \n[   ] threadcol.zip                      06-Jan-2013 08:46  378K  \n[DIR] threadcol/                         06-Jan-2013 08:46    -   \n[   ] threeparttable.zip                 07-Mar-2010 19:32  278K  \n[DIR] threeparttable/                    07-Mar-2010 19:33    -   \n[   ] threeparttablex.zip                22-May-2014 12:46   65K  \n[DIR] threeparttablex/                   22-May-2014 12:46    -   \n[   ] thucoursework.zip                  01-Apr-2018 09:00  408K  \n[DIR] thucoursework/                     01-Apr-2018 09:00    -   \n[   ] thumb.zip                          21-Jun-2005 12:04  203K  \n[DIR] thumb/                             23-Jan-2006 08:44    -   \n[   ] thumbs.zip                         09-Mar-2014 20:22  715K  \n[DIR] thumbs/                            09-Mar-2014 20:23    -   \n[   ] thumby.zip                         15-Jan-2010 14:14  159K  \n[DIR] thumby/                            15-Jan-2010 14:23    -   \n[   ] thuthesis.zip                      24-Dec-2017 08:53  2.2M  \n[DIR] thuthesis/                         24-Dec-2017 08:53    -   \n[   ] ticket.zip                         11-Oct-2016 17:34  505K  \n[DIR] ticket/                            11-Oct-2016 17:34    -   \n[   ] timbreicmc.zip                     15-Dec-2017 10:19  416K  \n[DIR] timbreicmc/                        15-Dec-2017 10:19    -   \n[   ] timing.zip                         28-Jun-2005 13:50  104K  \n[DIR] timing/                            23-Jan-2006 08:44    -   \n[   ] titlecaps.zip                      30-Jan-2015 14:58  260K  \n[DIR] titlecaps/                         30-Jan-2015 14:58    -   \n[   ] titlefoot.zip                      30-Apr-2005 16:09  2.7K  \n[DIR] titlefoot/                         01-Feb-2005 20:43    -   \n[   ] titlepage-uni-dortmund.zip         14-Aug-2006 10:24  1.0M  \n[DIR] titlepage-uni-dortmund/            14-Aug-2006 10:24    -   \n[   ] titlepic.zip                       14-Mar-2017 12:38  122K  \n[DIR] titlepic/                          14-Mar-2017 12:38    -   \n[   ] titleref.zip                       03-Jun-2010 16:14  198K  \n[DIR] titleref/                          03-Jun-2010 16:23    -   \n[   ] titlesec.zip                       21-Mar-2016 21:25  374K  \n[DIR] titlesec/                          21-Mar-2016 21:25    -   \n[   ] titling.zip                        04-Sep-2009 11:47  188K  \n[DIR] titling/                           04-Sep-2009 11:47    -   \n[   ] tkz-doc.zip                        05-Jun-2011 20:59  9.0K  \n[DIR] tkz-doc/                           05-Jun-2011 20:59    -   \n[DIR] tkz/                               10-Mar-2016 10:53    -   \n[   ] tocbibind.zip                      13-Oct-2010 11:39  315K  \n[DIR] tocbibind/                         13-Oct-2010 11:43    -   \n[   ] tocdata.zip                        02-Dec-2016 12:41  1.6M  \n[DIR] tocdata/                           02-Dec-2016 12:41    -   \n[   ] tocloft.zip                        31-Aug-2017 05:26  513K  \n[DIR] tocloft/                           31-Aug-2017 05:26    -   \n[   ] tocvsec2.zip                       10-Mar-2014 12:01  301K  \n[DIR] tocvsec2/                          10-Mar-2014 12:03    -   \n[   ] todo.zip                           01-Apr-2010 01:21  186K  \n[DIR] todo/                              01-Apr-2010 02:03    -   \n[   ] todonotes.zip                      02-Nov-2016 14:55  432K  \n[DIR] todonotes/                         02-Nov-2016 14:55    -   \n[   ] tokenizer.zip                      08-Jun-2005 18:22   74K  \n[DIR] tokenizer/                         23-Jan-2006 08:44    -   \n[   ] toolbox.zip                        27-Nov-2013 08:54  161K  \n[DIR] toolbox/                           27-Nov-2013 09:03    -   \n[   ] topfloat.zip                       17-Jan-2007 09:50   42K  \n[DIR] topfloat/                          17-Jan-2007 09:53    -   \n[   ] toptesi.zip                        21-Jan-2018 18:45  6.6M  \n[DIR] toptesi/                           21-Jan-2018 18:45    -   \n[   ] totcount.zip                       25-Jan-2011 20:17  284K  \n[DIR] totcount/                          25-Jan-2011 20:23    -   \n[   ] totpages.zip                       20-Sep-2005 17:24  185K  \n[DIR] totpages/                          20-Sep-2005 17:43    -   \n[   ] tpcmfont.zip                       30-Apr-2005 16:10  8.7K  \n[DIR] tpcmfont/                          01-Feb-2005 20:43    -   \n[   ] tqft.zip                           01-Jun-2017 14:36  740K  \n[DIR] tqft/                              01-Jun-2017 14:36    -   \n[DIR] tracking/                          03-Apr-2010 15:21    -   \n[   ] tram.zip                           04-Apr-2013 12:25   31K  \n[DIR] tram/                              04-Apr-2013 12:25    -   \n[   ] translations.zip                   31-Aug-2017 19:26  517K  \n[DIR] translations/                      31-Aug-2017 19:26    -   \n[   ] translator.zip                     05-Jan-2018 09:14  270K  \n[DIR] translator/                        05-Jan-2018 09:14    -   \n[   ] treesvr.zip                        22-Jul-2005 09:45   51K  \n[DIR] treesvr/                           23-Jan-2006 08:44    -   \n[   ] trfsigns.zip                       29-Jun-2005 21:08  204K  \n[DIR] trfsigns/                          16-Aug-2008 14:48    -   \n[   ] trimspaces.zip                     17-Sep-2009 13:53  149K  \n[DIR] trimspaces/                        17-Sep-2009 14:03    -   \n[   ] trivfloat.zip                      24-Apr-2009 01:07  135K  \n[DIR] trivfloat/                         24-Apr-2009 02:03    -   \n[   ] truncate.zip                       18-May-2010 23:12  156K  \n[DIR] truncate/                          18-May-2010 23:13    -   \n[DIR] tsemlines/                         25-Jun-2011 11:44    -   \n[   ] tucv.zip                           06-Dec-2010 20:16  255K  \n[DIR] tucv/                              06-Dec-2010 20:23    -   \n[   ] tudscr.zip                         30-May-2017 22:25  5.0M  \n[DIR] tudscr/                            30-May-2017 22:25    -   \n[   ] tufte-latex.zip                    22-Jun-2015 09:17  628K  \n[DIR] tufte-latex/                       22-Jun-2015 09:17    -   \n[   ] tugboat.zip                        07-Nov-2017 10:36  820K  \n[DIR] tugboat/                           07-Nov-2017 10:36    -   \n[   ] tui.zip                            30-Jul-2012 16:59  274K  \n[DIR] tui/                               30-Jul-2012 16:59    -   \n[   ] turabian-formatting.zip            04-Nov-2017 23:17  120K  \n[DIR] turabian-formatting/               04-Nov-2017 23:17    -   \n[   ] turabian.zip                       16-Feb-2015 17:43  6.1K  \n[DIR] turabian/                          16-Feb-2015 17:43    -   \n[   ] turnstile.zip                      07-Sep-2007 13:53  617K  \n[DIR] turnstile/                         07-Sep-2007 14:03    -   \n[   ] turnthepage.zip                    03-Sep-2011 09:32   85K  \n[DIR] turnthepage/                       03-Sep-2011 09:33    -   \n[   ] twoinone.zip                       13-Feb-2010 21:50   72K  \n[DIR] twoinone/                          13-Feb-2010 21:53    -   \n[   ] twoup.zip                          27-Feb-2007 14:35  181K  \n[DIR] twoup/                             27-Feb-2007 14:43    -   \n[   ] txgreeks.zip                       26-Mar-2011 12:45   61K  \n[DIR] txgreeks/                          26-Mar-2011 12:45    -   \n[   ] type1cm.zip                        24-Mar-2011 10:36  321K  \n[DIR] type1cm/                           24-Mar-2011 10:43    -   \n[   ] typed-checklist.zip                10-Apr-2016 18:06  402K  \n[DIR] typed-checklist/                   10-Apr-2016 18:06    -   \n[   ] typedref.zip                       27-Mar-2013 12:20  195K  \n[DIR] typedref/                          27-Mar-2013 12:23    -   \n[   ] typeface.zip                       19-Jun-2012 16:29   17M  \n[DIR] typeface/                          19-Jun-2012 16:29    -   \n[   ] typehtml.zip                       19-Feb-2010 10:19  171K  \n[DIR] typehtml/                          19-Feb-2010 10:23    -   \n[   ] typoaid.zip                        07-May-2017 16:05  330K  \n[DIR] typoaid/                           07-May-2017 16:05    -   \n[   ] typogrid.zip                       01-Jan-2012 15:09  292K  \n[DIR] typogrid/                          01-Jan-2012 15:09    -   \n[   ] uaclasses.zip                      05-Jan-2009 21:06  218K  \n[DIR] uaclasses/                         05-Jan-2009 21:13    -   \n[   ] uafthesis.zip                      11-Dec-2012 15:06   44K  \n[DIR] uafthesis/                         11-Dec-2012 15:13    -   \n[   ] uantwerpendocs.zip                 02-Mar-2018 13:22  2.2M  \n[DIR] uantwerpendocs/                    02-Mar-2018 13:22    -   \n[   ] uassign.zip                        23-Sep-2015 22:46  107K  \n[DIR] uassign/                           23-Sep-2015 22:46    -   \n[   ] ucbthesis.zip                      16-Jun-2015 05:08  172K  \n[DIR] ucbthesis/                         16-Jun-2015 05:08    -   \n[   ] ucdavisthesis.zip                  26-Apr-2016 08:09  1.7M  \n[DIR] ucdavisthesis/                     26-Apr-2016 08:09    -   \n[   ] ucharcat.zip                       20-Nov-2015 05:45  157K  \n[DIR] ucharcat/                          20-Nov-2015 05:45    -   \n[   ] ucs.zip                            14-May-2013 10:45  1.8M  \n[DIR] ucs/                               14-May-2013 10:53    -   \n[   ] ucthesis.zip                       27-Apr-2005 00:46   39K  \n[DIR] ucthesis/                          01-Feb-2005 20:43    -   \n[   ] udesoftec.zip                      28-Mar-2018 12:08  644K  \n[DIR] udesoftec/                         28-Mar-2018 12:08    -   \n[   ] uebungsblatt.zip                   25-Oct-2006 18:50  227K  \n[DIR] uebungsblatt/                      25-Oct-2006 18:53    -   \n[   ] uestcthesis.zip                    24-Feb-2015 13:42  4.2M  \n[DIR] uestcthesis/                       24-Feb-2015 13:42    -   \n[   ] uhhassignment.zip                  24-Apr-2017 08:21  378K  \n[DIR] uhhassignment/                     24-Apr-2017 08:21    -   \n[   ] uhrzeit.zip                        02-Feb-2016 17:51  205K  \n[DIR] uhrzeit/                           02-Feb-2016 17:51    -   \n[   ] uiucredborder.zip                  14-Apr-2013 14:30  325K  \n[DIR] uiucredborder/                     14-Apr-2013 14:33    -   \n[   ] uiucthesis.zip                     17-May-2005 16:04  251K  \n[DIR] uiucthesis/                        17-May-2005 18:13    -   \n[   ] ulem.zip                           01-Jun-2012 11:33  108K  \n[DIR] ulem/                              01-Jun-2012 11:43    -   \n[   ] ulqda.zip                          11-Jun-2009 13:47  275K  \n[DIR] ulqda/                             11-Jun-2009 13:53    -   \n[   ] ulthese.zip                        01-Jun-2017 19:15  345K  \n[DIR] ulthese/                           01-Jun-2017 19:15    -   \n[   ] umbclegislation.zip                10-Jun-2016 10:33   18K  \n[DIR] umbclegislation/                   10-Jun-2016 10:33    -   \n[   ] umich-thesis.zip                   27-Apr-2005 00:46  6.3K  \n[DIR] umich-thesis/                      01-Feb-2005 20:43    -   \n[   ] umlaute.zip                        02-Feb-2006 01:00  111K  \n[DIR] umlaute/                           16-Aug-2008 14:48    -   \n[   ] umoline.zip                        30-Jul-2005 13:21  215K  \n[DIR] umoline/                           30-Jul-2005 12:43    -   \n[   ] umthesis.zip                       17-Sep-2009 18:58  104K  \n[DIR] umthesis/                          17-Sep-2009 19:03    -   \n[   ] unamth-template.zip                22-Apr-2014 18:31  5.1M  \n[DIR] unamth-template/                   22-Apr-2014 18:33    -   \n[   ] unamthesis.zip                     29-Mar-2017 05:25  807K  \n[DIR] unamthesis/                        29-Mar-2017 05:25    -   \n[   ] underlin.zip                       09-Sep-2006 13:16   72K  \n[DIR] underlin/                          09-Sep-2006 13:10    -   \n[   ] underoverlap.zip                   03-Feb-2013 18:52  269K  \n[DIR] underoverlap/                      03-Feb-2013 18:53    -   \n[   ] underscore.zip                     11-May-2010 22:10  245K  \n[DIR] underscore/                        11-May-2010 22:13    -   \n[   ] undertilde.zip                     23-Jun-2005 11:26  160K  \n[DIR] undertilde/                        16-Aug-2008 14:48    -   \n[   ] undolabl.zip                       30-Mar-2015 15:48  357K  \n[DIR] undolabl/                          30-Mar-2015 15:48    -   \n[   ] unicode-math.zip                   01-Feb-2018 15:18  2.1M  \n[DIR] unicode-math/                      01-Feb-2018 15:18    -   \n[   ] unitn-bimrep.zip                   22-Oct-2017 12:56  1.1M  \n[DIR] unitn-bimrep/                      22-Oct-2017 12:56    -   \n[   ] units.zip                          30-Jul-2005 13:20  212K  \n[DIR] units/                             23-Jan-2006 08:44    -   \n[   ] unitsdef.zip                       27-Apr-2005 00:46  639K  \n[DIR] unitsdef/                          01-Feb-2005 20:43    -   \n[   ] univie-ling.zip                    02-Mar-2018 12:19  2.7M  \n[DIR] univie-ling/                       02-Mar-2018 12:19    -   \n[   ] unravel.zip                        30-Sep-2015 07:37  736K  \n[DIR] unravel/                           30-Sep-2015 07:37    -   \n[   ] unswcover.zip                      22-Mar-2013 09:12  164K  \n[DIR] unswcover/                         22-Mar-2013 09:12    -   \n[   ] unswthesis.zip                     31-Mar-2015 09:44   11K  \n[DIR] unswthesis/                        31-Mar-2015 09:44    -   \n[   ] uothesis.zip                       09-Feb-2012 17:28  625K  \n[DIR] uothesis/                          09-Feb-2012 17:33    -   \n[   ] uowthesis.zip                      25-Jul-2010 17:10  147K  \n[DIR] uowthesis/                         25-Jul-2010 17:13    -   \n[   ] uowthesistitlepage.zip             11-Aug-2017 08:51  2.1M  \n[DIR] uowthesistitlepage/                11-Aug-2017 08:51    -   \n[   ] upmethodology.zip                  10-Dec-2017 23:09  623K  \n[DIR] upmethodology/                     10-Dec-2017 23:09    -   \n[   ] upquote.zip                        19-Apr-2012 20:52  163K  \n[DIR] upquote/                           19-Apr-2012 20:52    -   \n[   ] urcls.zip                          10-Apr-2017 10:51  921K  \n[DIR] urcls/                             10-Apr-2017 10:51    -   \n[   ] uri.zip                            04-Mar-2011 21:12  391K  \n[DIR] uri/                               04-Mar-2011 21:12    -   \n[   ] url.zip                            31-Dec-2013 14:56  264K  \n[DIR] url/                               31-Dec-2013 14:56    -   \n[   ] usebib.zip                         13-Apr-2012 23:50  253K  \n[DIR] usebib/                            13-Apr-2012 23:53    -   \n[   ] ushort.zip                         27-Nov-2013 06:49   75K  \n[DIR] ushort/                            27-Nov-2013 06:49    -   \n[   ] uspace.zip                         06-Nov-2016 22:30  397K  \n[DIR] uspace/                            06-Nov-2016 22:30    -   \n[   ] uspatent.zip                       19-Sep-2012 17:52  2.4M  \n[DIR] uspatent/                          19-Sep-2012 17:52    -   \n[   ] ut-thesis.zip                      01-Sep-2015 20:47   11K  \n[DIR] ut-thesis/                         01-Sep-2015 20:47    -   \n[   ] utorontothesis.zip                 27-Apr-2005 00:46  4.2K  \n[DIR] utorontothesis/                    01-Feb-2005 20:43    -   \n[   ] utthesis.zip                       27-Apr-2005 00:46  624K  \n[DIR] utthesis/                          01-Feb-2005 20:43    -   \n[   ] uwmslide.zip                       27-Apr-2005 00:46   17K  \n[DIR] uwmslide/                          23-Jan-2006 08:44    -   \n[   ] uwthesis.zip                       14-Jul-2008 00:03  147K  \n[DIR] uwthesis/                          13-Jul-2008 23:13    -   \n[   ] varindex.zip                       27-Nov-2013 07:29  260K  \n[DIR] varindex/                          27-Nov-2013 07:29    -   \n[   ] varsfromjobname.zip                01-May-2017 23:09  182K  \n[DIR] varsfromjobname/                   01-May-2017 23:09    -   \n[   ] varwidth.zip                       26-Sep-2011 11:11   30K  \n[DIR] varwidth/                          26-Sep-2011 11:13    -   \n[   ] vdm.zip                            07-Apr-2006 19:43  189K  \n[DIR] vdm/                               07-Apr-2006 19:13    -   \n[   ] vdmlisting.zip                     14-Apr-2013 10:17   69K  \n[DIR] vdmlisting/                        14-Apr-2013 10:17    -   \n[   ] vector.zip                         13-Aug-2005 02:00  166K  \n[DIR] vector/                            16-Aug-2008 14:48    -   \n[   ] venndiagram.zip                    16-Mar-2016 23:37  340K  \n[DIR] venndiagram/                       16-Mar-2016 23:37    -   \n[   ] verbasef.zip                       02-Apr-2011 14:56  332K  \n[DIR] verbasef/                          02-Apr-2011 15:03    -   \n[   ] verbatimbox.zip                    12-Mar-2014 19:16  244K  \n[DIR] verbatimbox/                       12-Mar-2014 19:23    -   \n[   ] verbatimcopy.zip                   17-Nov-2008 13:48  164K  \n[DIR] verbatimcopy/                      17-Nov-2008 13:53    -   \n[   ] verbdef.zip                        23-Feb-2010 21:27   55K  \n[DIR] verbdef/                           23-Feb-2010 21:33    -   \n[   ] verbments.zip                      22-Aug-2011 13:52   77K  \n[DIR] verbments/                         22-Aug-2011 13:52    -   \n[   ] verse.zip                          11-May-2014 07:41  426K  \n[DIR] verse/                             11-May-2014 07:41    -   \n[   ] version.zip                        02-Apr-2011 15:39  298K  \n[DIR] version/                           02-Apr-2011 15:43    -   \n[   ] versions.zip                       02-Apr-2011 19:37  350K  \n[DIR] versions/                          02-Apr-2011 19:43    -   \n[   ] versonotes.zip                     09-Dec-2015 07:55  195K  \n[DIR] versonotes/                        09-Dec-2015 07:55    -   \n[   ] vertbars.zip                       27-Nov-2010 12:51   36K  \n[DIR] vertbars/                          27-Nov-2010 12:53    -   \n[   ] vgrid.zip                          20-Dec-2013 18:40   25K  \n[DIR] vgrid/                             20-Dec-2013 18:43    -   \n[   ] vhistory.zip                       21-Apr-2013 16:50  374K  \n[DIR] vhistory/                          21-Apr-2013 16:50    -   \n[   ] viiptart.zip                       27-Apr-2005 00:46  6.7K  \n[DIR] viiptart/                          01-Feb-2005 20:43    -   \n[   ] vita.zip                           27-Apr-2005 00:46   12K  \n[DIR] vita/                              23-Jan-2006 08:44    -   \n[   ] vmargin.zip                        27-Apr-2005 00:46  164K  \n[DIR] vmargin/                           01-Feb-2005 20:43    -   \n[   ] volumes.zip                        29-Jul-2005 18:48  155K  \n[DIR] volumes/                           29-Jul-2005 19:13    -   \n[   ] vpe.zip                            01-Aug-2006 11:47   15K  \n[DIR] vpe/                               16-Jul-2012 11:10    -   \n[   ] vrsion.zip                         22-Jun-2005 11:40  257K  \n[DIR] vrsion/                            23-Jan-2006 08:44    -   \n[   ] vruler.zip                         03-Mar-2011 10:32  222K  \n[DIR] vruler/                            03-Mar-2011 10:33    -   \n[   ] vwcol.zip                          10-Feb-2015 12:58  277K  \n[DIR] vwcol/                             10-Feb-2015 12:58    -   \n[   ] wallpaper.zip                      21-Apr-2006 20:29  1.2M  \n[DIR] wallpaper/                         21-Apr-2006 20:44    -   \n[   ] warning.zip                        08-Apr-2011 17:39  250K  \n[DIR] warning/                           08-Apr-2011 17:43    -   \n[   ] warpcol.zip                        21-Nov-2007 17:34   88K  \n[DIR] warpcol/                           21-Nov-2007 17:43    -   \n[   ] was.zip                            15-Feb-2011 08:47  662K  \n[DIR] was/                               15-Feb-2011 08:53    -   \n[   ] wasysym.zip                        27-Apr-2005 00:45   98K  \n[DIR] wasysym/                           01-Feb-2005 20:43    -   \n[   ] widetable.zip                      09-Sep-2017 10:46  379K  \n[DIR] widetable/                         09-Sep-2017 10:46    -   \n[   ] williams.zip                       30-Jan-2009 13:40  3.2K  \n[DIR] williams/                          30-Jan-2009 13:43    -   \n[   ] withargs.zip                       20-Dec-2016 06:50  469K  \n[DIR] withargs/                          20-Dec-2016 06:50    -   \n[   ] witharrows.zip                     12-Feb-2018 13:33  277K  \n[DIR] witharrows/                        12-Feb-2018 13:33    -   \n[   ] withesis.zip                       27-Apr-2005 00:45  108K  \n[DIR] withesis/                          23-Jan-2006 08:44    -   \n[   ] wnri-latex.zip                     06-May-2011 00:45  199K  \n[DIR] wnri-latex/                        06-May-2011 02:03    -   \n[   ] wordcount.zip                      03-Jun-2016 08:20  5.7K  \n[DIR] wordcount/                         03-Jun-2016 08:20    -   \n[   ] wordlike.zip                       30-Mar-2006 09:55  116K  \n[DIR] wordlike/                          16-Aug-2008 14:48    -   \n[   ] wrapfig.zip                        09-Apr-2011 11:24  338K  \n[DIR] wrapfig/                           09-Apr-2011 11:33    -   \n[   ] wsemclassic.zip                    27-Aug-2013 14:51  399K  \n[DIR] wsemclassic/                       27-Aug-2013 14:53    -   \n[   ] wtref.zip                          17-Jan-2017 12:20  337K  \n[DIR] wtref/                             17-Jan-2017 12:20    -   \n[   ] xargs.zip                          24-Mar-2008 21:05  211K  \n[DIR] xargs/                             24-Mar-2008 21:05    -   \n[   ] xassoccnt.zip                      04-Jan-2018 09:47  1.2M  \n[DIR] xassoccnt/                         04-Jan-2018 09:47    -   \n[   ] xcite.zip                          03-Sep-2011 00:23  204K  \n[DIR] xcite/                             03-Sep-2011 02:03    -   \n[   ] xcjk2uni.zip                       30-Jan-2018 20:00  133K  \n[DIR] xcjk2uni/                          30-Jan-2018 20:00    -   \n[   ] xcntperchap.zip                    05-Jan-2018 22:15  363K  \n[DIR] xcntperchap/                       05-Jan-2018 22:15    -   \n[   ] xcolor-material.zip                16-Oct-2016 08:45  578K  \n[DIR] xcolor-material/                   16-Oct-2016 08:45    -   \n[   ] xcolor-solarized.zip               05-Aug-2016 23:14  462K  \n[DIR] xcolor-solarized/                  05-Aug-2016 23:14    -   \n[   ] xcolor.zip                         11-May-2016 08:30  752K  \n[DIR] xcolor/                            11-May-2016 08:30    -   \n[   ] xcookybooky.zip                    04-Mar-2015 06:01  1.1M  \n[DIR] xcookybooky/                       04-Mar-2015 06:01    -   \n[   ] xdoc.zip                           01-Mar-2005 01:24  916K  \n[DIR] xdoc/                              23-Jan-2006 08:44    -   \n[   ] xduthesis.zip                      11-Feb-2016 05:43  814K  \n[DIR] xduthesis/                         11-Feb-2016 05:43    -   \n[   ] xellipsis.zip                      20-Dec-2016 22:07  346K  \n[DIR] xellipsis/                         20-Dec-2016 22:07    -   \n[   ] xfor.zip                           05-Feb-2009 23:15  105K  \n[DIR] xfor/                              05-Feb-2009 23:23    -   \n[   ] xhfill.zip                         15-May-2011 00:35   39K  \n[DIR] xhfill/                            15-May-2011 02:03    -   \n[   ] xifthen.zip                        23-Nov-2015 13:32  471K  \n[DIR] xifthen/                           23-Nov-2015 13:32    -   \n[   ] xkeyval.zip                        03-Dec-2014 21:38  436K  \n[DIR] xkeyval/                           03-Dec-2014 21:38    -   \n[   ] xltabular.zip                      26-Oct-2017 13:21   73K  \n[DIR] xltabular/                         26-Oct-2017 13:21    -   \n[   ] xltxtra.zip                        21-Jan-2016 09:00  135K  \n[DIR] xltxtra/                           21-Jan-2016 09:00    -   \n[   ] xmpincl.zip                        10-May-2008 13:51  105K  \n[DIR] xmpincl/                           10-May-2008 13:53    -   \n[   ] xnewcommand.zip                    24-Apr-2007 03:02  261K  \n[DIR] xnewcommand/                       24-Apr-2007 03:13    -   \n[   ] xoptarg.zip                        23-Apr-2007 13:42  362K  \n[DIR] xoptarg/                           23-Apr-2007 13:43    -   \n[   ] xpatch.zip                         05-Oct-2012 00:21  446K  \n[DIR] xpatch/                            05-Oct-2012 02:03    -   \n[   ] xpeek.zip                          17-Aug-2012 11:59  551K  \n[DIR] xpeek/                             17-Aug-2012 12:03    -   \n[   ] xpiano.zip                         23-May-2015 16:57  548K  \n[DIR] xpiano/                            23-May-2015 16:57    -   \n[   ] xpicture.zip                       02-Jan-2013 13:57  1.3M  \n[DIR] xpicture/                          02-Jan-2013 14:03    -   \n[   ] xpinyin.zip                        30-Jan-2018 21:39  212K  \n[DIR] xpinyin/                           30-Jan-2018 21:39    -   \n[   ] xprintlen.zip                      28-Dec-2014 11:17  137K  \n[DIR] xprintlen/                         28-Dec-2014 11:17    -   \n[   ] xpunctuate.zip                     24-May-2012 06:55  200K  \n[DIR] xpunctuate/                        24-May-2012 06:55    -   \n[   ] xsavebox.zip                       29-Mar-2018 18:45  368K  \n[DIR] xsavebox/                          29-Mar-2018 18:45    -   \n[   ] xsim.zip                           14-Feb-2018 13:22  2.6M  \n[DIR] xsim/                              14-Feb-2018 13:22    -   \n[   ] xskak.zip                          02-Jan-2015 17:09  628K  \n[DIR] xskak/                             02-Jan-2015 17:09    -   \n[   ] xtab.zip                           31-Jul-2011 15:57  372K  \n[DIR] xtab/                              31-Jul-2011 15:57    -   \n[   ] xtcapts.zip                        10-Jan-2007 17:40  101K  \n[DIR] xtcapts/                           16-Aug-2008 14:48    -   \n[   ] xtuthesis.zip                      20-Mar-2018 20:16  1.3M  \n[DIR] xtuthesis/                         20-Mar-2018 20:16    -   \n[   ] xurl.zip                           09-Jan-2018 11:06   42K  \n[DIR] xurl/                              09-Jan-2018 11:06    -   \n[   ] xwatermark.zip                     26-Oct-2012 10:05  600K  \n[DIR] xwatermark/                        26-Oct-2012 10:13    -   \n[   ] xyling.zip                         01-Aug-2006 09:51  157K  \n[DIR] xyling/                            01-Aug-2006 09:51    -   \n[   ] xymtex.zip                         11-Oct-2013 19:13   15M  \n[DIR] xymtex/                            11-Oct-2013 19:13    -   \n[DIR] xypic/                             06-Oct-2013 18:03    -   \n[   ] xytree.zip                         29-Aug-2006 02:34  235K  \n[DIR] xytree/                            29-Aug-2006 02:43    -   \n[   ] yafoot.zip                         01-Mar-2005 01:24   18K  \n[DIR] yafoot/                            11-Jan-2006 18:13    -   \n[   ] yagusylo.zip                       27-Sep-2012 19:11  2.2M  \n[DIR] yagusylo/                          27-Feb-2009 10:07    -   \n[   ] yaletter.zip                       01-Jan-2017 22:53  503K  \n[DIR] yaletter/                          01-Jan-2017 22:53    -   \n[   ] yathesis.zip                       09-Dec-2016 21:40   12M  \n[DIR] yathesis/                          09-Dec-2016 21:40    -   \n[   ] ycbook.zip                         02-Jan-2018 23:31  126K  \n[DIR] ycbook/                            02-Jan-2018 23:31    -   \n[   ] ydoc.zip                           03-May-2012 17:12  330K  \n[DIR] ydoc/                              03-May-2012 17:13    -   \n[   ] yfonts.zip                         01-Mar-2005 01:24   13K  \n[DIR] yfonts/                            23-Jan-2006 08:44    -   \n[DIR] yhmath/                            31-Jan-2018 15:59    -   \n[   ] york-thesis.zip                    13-Jun-2011 23:57  122K  \n[DIR] york-thesis/                       14-Jun-2011 02:03    -   \n[   ] youngtab.zip                       30-Mar-2010 14:40  157K  \n[DIR] youngtab/                          30-Mar-2010 14:43    -   \n[   ] yplan.zip                          01-Mar-2005 01:24   14K  \n[DIR] yplan/                             16-Dec-2006 09:13    -   \n[   ] yt4pdf.zip                         13-Oct-2016 15:31  1.5M  \n[DIR] yt4pdf/                            13-Oct-2016 15:31    -   \n[   ] ytableau.zip                       16-Aug-2012 11:10  366K  \n[DIR] ytableau/                          16-Aug-2012 11:10    -   \n[   ] zebra-goodies.zip                  06-Dec-2017 09:47  2.6K  \n[DIR] zebra-goodies/                     06-Dec-2017 09:47    -   \n[   ] zed-csp.zip                        06-Aug-2005 16:28  243K  \n[DIR] zed-csp/                           09-Aug-2005 01:10    -   \n[   ] zhlipsum.zip                       06-Jan-2018 10:25  313K  \n[DIR] zhlipsum/                          06-Jan-2018 10:25    -   \n[   ] zhnumber.zip                       29-Jan-2018 20:33  277K  \n[DIR] zhnumber/                          29-Jan-2018 20:33    -   \n[   ] ziffer.zip                         30-Nov-2013 00:51  2.0K  \n[DIR] ziffer/                            30-Nov-2013 02:03    -   \n[   ] zwgetfdate.zip                     22-Jun-2008 19:52  243K  \n[DIR] zwgetfdate/                        22-Jun-2008 19:53    -   \n[   ] zwpagelayout.zip                   06-Jul-2013 22:22  732K  \n[DIR] zwpagelayout/                      06-Jul-2013 22:23    -   \n\n"  # CTAN-Mirror RWTH-Aachen FTP Folder content
  w12 = "http://vesta.informatik.rwth-aachen.de/ftp/pub/mirror/ctan/macros/latex/contrib/"  # CTAN-Mirror RWTH-Aachen
  n1 = disable-structure shown="Disabled" {
    disable-tunnel: w12 -> [w17 _]
    frame Disabled {
      n2 = call <vilib>:"OpenHandle.vi"() -> ("client handle out"=w18:T1, "error out"=w19:errorcluster)  [unwired: 14 in]
      n3 = call <vilib>:"GET.vi"("client handle"=w18, "url"=w17, "error in (no error)"=w19, "timeout (10000)"=100000) -> ("client handle out"=w16:T1, "headers"=→"headers":string, "body"=→"body":string, "error out"=w20:errorcluster)  [unwired: 8 in]
      n4 = call <vilib>:"CloseHandle.vi"("client handle"=w16, "error in (no error)"=w20) -> ()  [unwired: 13 in, 1 out]
    }
    frame Enabled {
    }
  }
  n5 = Spreadsheet String To Array(format string="", spreadsheet string=w11, array type (2D Dbl)=string[][] [] ("Array String 2")) -> (array=w8:string[][])  [unwired: 1 in]
  "Array String" <- w8
  n6 = Index Array(array=w8, index (col)=0 ("disabled index (col)")) -> (element=w3:string[])  [unwired: 1 in]
  n7 = for {
    tunnel: w3 -> [w21] mode=indexing
    tunnel: [w26] -> w6 mode=indexing if=w24
    tunnel: [w25] -> w5 mode=indexing if=w24
    tunnel: "[a-zA-z0-9\\-\\_\\%\\ß\\?]+\\.zip" ("regular expression") -> [w23]
    i -> [w26]
    n8 = xnode "Match Regular Expression"("input string"=w21, "regular expression"=w23, "offset (0)"=6) -> ("whole match"=w25:string, "offset past match"=w27:i32)  [unwired: 3 in, 3 out]
    n9 = Greater Or Equal To 0?(x=w27) -> (x >= 0?=w24:bool)
  }
  "Array" <- w6
  "Array 2" <- w5
  n10 = for {
    tunnel: w3 -> [w147] mode=indexing
    tunnel: ".zip" ("regular expression") -> [w150]
    tunnel: [w142] -> w1 mode=indexing if=w148
    n11 = String Subset(string=w147, offset (0)=6) -> (substring=w145:string)  [unwired: 1 in]
    n12 = Match Pattern(string=w145, regular expression=w150) -> (before substring=w144:string, match substring=w143:string, offset past match=w149:i32)  [unwired: 1 in, 1 out]
    n13 = Concatenate Strings(w144, w143) -> (w142:string)
    n14 = Greater Or Equal To 0?(x=w149) -> (x >= 0?=w148:bool)
  }
  "Array 3" <- w1
